vi "state machine plantenna with internal test V2.vi"() -> ()   [LabVIEW 2018]
uses:
  wobbe statemachine.ctl
  Control 1.ctl
  D:/projects/plantenna/stomata programs/plantenna/plantenna/Kinesis_with_LabVIEW_Examples_LV12 - v3/Thorlabs.MotionControl.Controls.dll
  Kinesis_with_LabVIEW_Examples_LV12 - v3/Thorlabs.MotionControl.Controls.dll
  <vilib>/userdefined/High Color/IMAQdx.ctl
  D:/projects/plantenna/stomata programs/plantenna/plantenna/Kinesis_with_LabVIEW_Examples_LV12 - v3/ThorLabs.MotionControl.KCube.DCServoCLI.dll
  Kinesis_with_LabVIEW_Examples_LV12 - v3/ThorLabs.MotionControl.KCube.DCServoCLI.dll
  <vilib>/vision/Image Controls.llb/IMAQ Image.ctl
  <vilib>/Analysis/6fits.llb/Curve Fitting Criteria.ctl
  read settings control.ctl
  write camera.ctl
  <vilib>/Utility/error.llb/DialogType.ctl
  LightStudio 485/labview light studio/chan select.ctl
  <vilib>/vision/driver/IMAQdx.llb/IMAQdx Camera Control Mode.ctl
  <vilib>/Platform/TimedLoop/XDataNode/timing_clust.ctl
  <vilib>/Platform/TimedLoop/XDataNode/nitl_modes.ctl
  <vilib>/Platform/TimedLoop/XDataNode/wakeup.ctl
  <vilib>/DAQmx/write.llb/DAQmx Write (Analog DBL 1Chan 1Samp).vi
  <vilib>/Instr/_visa.llb/VISA Configure Serial Port (Instr).vi
  <vilib>/DAQmx/miscellaneous.llb/DAQmx Fill In Error Info.vi
  <vilib>/Utility/file.llb/Write Delimited Spreadsheet (DBL).vi
  <vilib>/Utility/file.llb/Read Delimited Spreadsheet (string).vi
  <vilib>/platform/TimedLoop/XDataNode/XDataNode.xnode
  <vilib>/vision/driver/NI_Vision_Acquisition_Software.lvlib
  <vilib>/vision/NI_Vision_Development_Module.lvlib
  <vilib>/Analysis/NI_AALPro.lvlib
  <vilib>/Platform/TimedLoop/XDataNode/XDNodeRunTimeDep.lvlib
  <resource>/objmgr/imaqdx.rc
panel:
  out "move error":bool
  out "current state ( setup is idle)":T1=enum."camera settings"
  in  "stopprogram":bool
  in  "User Interface":bool
  in  "control tab":T2(tab)
  in  "blue":bool
  in  "green":bool
  in  "red":bool
  in  "blue":dbl(slide) scale=0.0..100.0
  in  "green":dbl(slide) min=0.0 max=100.0 step=1.0 scale=0.0..100.0
  in  "red":dbl(slide) scale=0.0..100.0
  in  "between meas":bool
  in  "plant light %":dbl(knob) min=0.0 max=100.0 step=0.1 scale=0.0..100.0
  in  "camera settings":bool
  in  "Set ROI":bool
  in  "Microscope light on/off":bool
  in  "StopROI":bool
  in  "use ROI":bool=TRUE
  in  "pics saved":bool
  in  "extra number of steps \nbottom side":dbl=100.0
  in  "extra scan depth \nbottom side(mm)":dbl=0.1
  in  "extra  steps":bool
  in  "extra number of steps \ntop side":dbl=100.0
  in  "extra stepsize (mm)":dbl=0.001
  in  "extra scan depth \ntop side(mm)":dbl=0.1
  out "total scan depth":dbl
  out "total nr of steps":dbl=100.0
  out "step nr":dbl
  out "start":dbl
  out "end":dbl
  in  "set position":dbl
  out "real position":dbl
  in  "number of steps":dbl=100.0
  in  "stepsize (mm)":dbl=0.001 step=0.001
  in  "focus point":dbl step=0.01
  in  "scan depth (mm)":dbl=0.1 min=0.001 step=0.01
  in  "use nonlin steps":bool
  in  "rough extra number \nof steps both sides":dbl=100.0
  in  "rough stepsize (mm)":dbl=0.001
  in  "rough extra scan depth \nboth sides(mm)":dbl=0.1
  in  "max alowed offset":dbl=0.0005
  in  "backlash offset":dbl=0.1
  in  "Test scan\n(no pic. saved)":bool
  in  "Camera settings write":T3={"Pixel format"=1, "exposure time [microsec]"=20.0, "Exposure time setting"=1, "gain [dB]"=0.0, "Auto Gain"=1, "Gamma enable"=FALSE, "gamma "=0.25, "ISP enable "=FALSE, "black level clamping enabled"=FALSE, "black level (%)"=0.0, "binning vertical"=1, "binning hor"=1, "vertical binning mode"=1, "horizontal  binning mode"=1, "width"=8.0, "height "=4.0} {"height" min=0.0 max=2300.0 step=4.0; "width" min=0.0 max=2660.0 step=4.0; "horizontal  binning mode" items=["Additive", "Average"]; "vertical binning mode" items=["Additive", "Average"]; "binning hor" items=["1", "2", "4"]; "binning vertical" items=["1", "2", "4"]; "black level (%)" min=-5.0 max=10.0; "gamma" min=0.25 max=4.0 step=0.1; "Auto Gain" items=["Continuous", "Once", "Off"]; "gain [dB]" min=0.0 max=47.0; "Exposure time setting" items=["Continuous", "Once", "Off"]; "exposure time [microsec]" min=20.0 max=30000000.0; "Pixel format" items=["Mono8", "Mono16", "Mono10Packed", "Mono12Packed", "Mono10p", "Mono12p"]}
  in  "Test Camera settings":bool
  in  "apply settings":bool
  in  "save focus data":bool
  in  "edge detection settings":T4(ring)
  in  "inverse gausian":bool
  in  "Gausian fit method":T5 items=["Least Square", "Least Absolute Residual", "Bisquare"]
  in  "Maximum standard deviation":dbl=0.1
  out "standard deviation 2":dbl
  in  "used for focuspoint":bool=TRUE
  in  "Run with \nexternal \ntiming settings":bool
  out "finished late !\nraise rep time":bool
  in  "start meas now":bool
  out "current time":timestamp format="%<%H:%M:%S>T"
  in  "start fast timer":bool
  in  "start at":timestamp=timestamp(3684335014.687392 s since 1904-01-01) format="%<%H:%M:%S>T"
  out "Last scan time (s)":dbl
  out "rep nr":i32
  out "elapsed time bar  (red idle time)":cluster{dbl, dbl, dbl}(slide)={0.0, 9e-323, 0.0} scale=0.0..60000.0
  out "Elapsed Time (s)":dbl
  in  "nr of repetitions":i32=10 min=1
  in  "repetition time [s]":i64=60 min=1
  in  "load external\n timing settings":bool
  out "plight [%]":i32=1
  out "mlight [%]":i32=1
  in  "serial psi channel":refnum<visa-resource-name>="COM4"
  in  "testrun without psi light":bool
  in  "testrun with pinocam":bool
  in  "Hide test feat.":bool
  in  "testrun without minipam":bool
  in  "testrun without motor":bool
  out "temp rep scan  state array":T1[](array[typedef])
  in  "IR Camera":T6="cam1"
  out "Splitter Position":i32
  in  "motor Serial Number":T7="27600724"
  out "motor prop ref":refnum<k24>
  out "Motor device ref":refnum<k24>
  out "IR camera session ref":T6 caption="Session Out"
  out "filtered image mem loc":T8
  out "Live image mem loc":T8
  out "ROI Mask mem loc":T8
  out "Filename with position":string
  out "filtered image":T8
  out "contrast value array":sgl[](array[numeric])
  out "real position array":dbl[](array[numeric])
  in  "selected path":path
  out "path":path
  out "start time":u32
  out "last scan time (tabs)":u32
  out "rep start time":u32
  in  "first timerscan run ?":bool
  in  "testrun without daq":bool
  in  "plight 100% voltage":dbl=10.0 caption="PLight100%volt" format="%0.2f"
  in  "wait control loop untill init":bool
  out "nrfrep":i32
  out "stop setup loop":bool
  out "rep time":i32
  in  "error in":errorcluster
  out "Initial State":T1=enum."camera settings"
  out "temp scan state array":T1[](array[typedef])
  out "state array":T1[](array[typedef])
  out "cam set read":T9={"Pixel format"=1, "exposure time [microsec]"=20.0, "Exposure time setting"=1, "gain [dB]"=0.0, "Auto Gain"=1, "Gamma enable"=FALSE, "gamma "=0.25, "ISP enable "=FALSE, "black level clamping enabled"=FALSE, "black level (%)"=0.0, "binning vertical"=1, "binning hor"=1, "vertical binning mode"=1, "horizontal  binning mode"=1, "width"=8.0, "height "=4.0, "max width"=8.0, "max height"=8.0, "exposure time vis"=enum."Enabled", "gain vis"=enum."Enabled", "vert binning vis"=[], "hor bin  vis"=[], "gamma vis"=enum."Enabled", "black level vis"=enum."Enabled"} {"max height" min=0.0 max=1330.0; "max width" min=0.0 max=1150.0; "height" min=0.0 max=1330.0; "horizontal  binning mode" items=["Additive", "Average"]; "vertical binning mode" items=["Additive", "Average"]; "binning hor" items=["1", "2", "4"]; "binning vertical" items=["1", "2", "4"]; "black level (%)" min=-5.0 max=10.0; "gamma" min=0.25 max=4.0 step=0.1; "Auto Gain" items=["Continuous", "Once", "Off"]; "gain [dB]" min=0.0 max=47.0; "Exposure time setting" items=["Continuous", "Once", "Off"]; "exposure time [microsec]" min=20.0 max=30000000.0; "Pixel format" items=["Mono8", "Mono16", "Mono10Packed", "Mono12Packed", "Mono10p", "Mono12p"]}
  in  "TIFF Options":T10={"Rows Per Strip"=0, "Photometric"=1, "Compression Type"=0} {"Compression Type" items=["None", "JPEG", "Run Length Encoded", "Zip"]; "Photometric" items=["WhiteIsZero", "BlackIsZero"]}
  out "temp test scan":bool
  out "rep start time 2":timestamp
  in  "io page Visible":bool=TRUE
  out "ROI Descriptor":T11 {"Contours"."Type" items=["No Selection", "Point", "Line", "Rectangle", "Oval", "Polygon", "Freehand Region", "Annulus", "Unused2", "Unused3", "Broken Line", "Freehand Line", "Rotated Rectangle"]}
  in  "encoder counts/rev":i32=34555
  in  "waveform tab":T12(tab)
  out "Waveform Graph":T13(graph)
  out "Live image setup tab":T8(plugin-control)
  in  "initalize motor":refnum<k24>(container)
  out "histogram Mean":sgl format="%#.2f"
  out "histogram Standard Deviation":sgl format="%#.2f"
  out "current time 2":timestamp format="%<%H:%M:%S>T"
  out "timer graph":cluster{cluster{timestamp, dbl}[]}[](graph)
  out "Timer settings array":string[][](array[string])
  out "date from file":string
  out "time from file":string
  out "current date and time":timestamp
  out "next function":string
  out "next function argument":string
  out "focus drift":dbl(graph)
  out "XY Graph":T14(graph)
  out "Gausian fit center":dbl
  out "standard deviation":dbl
  out "max position":dbl
  out "contrast value \n( high is better)":sgl format="%.2f"
  out "Live image camera tab":T8(plugin-control)
  # "nog te doen : microscoop lamp uit tussen de metingen"
  # "PSI light"
  # "settings file: \nYYYY-MM-DD\t    hh:mm:ss    \"command\"    [set]   OR\nDeltaT   hh:mm:ss    \"command\"    [set]\ncommands:\nmlight [on,off, 0-100%] microscope light on/off\nplight     [on,off, 0-100%]  plant light intesity change\nmpam    []  minipam pulse\nredpsiplight[on,off,0-100%] red channel PSI plant light intesity change\ngreenpsiplight[on,off,0-100%] green channel PSI plant light intesity change\nbluepsiplight[on,off,0-100%] blue channel PSI plant light intesity change \nfstack [] do a focus teststack without saving pictures\nrfstack []  do a nonliniar teststack without saving pics\nrstack []  do a single rough non lin stack\nrstack []  do a single stack\nrscan [ number of repetitions   time between meas(sec)] do a single non liniar scan and save the pics \nscan [number of repetitions   time between meas] do a scan and save pics\nexample :\n2020-09-21\t14:08:06\t plight\t80\n2020-09-21\t14:10:00\t mpam\n2020-09-21\t14:10:50  mlight on \n2020-09-21\t14:11:06\t rscan 10  120\n2020-09-21\t14:35:06  fstack\n\nOR\nDeltaT\t 14:08:06\t plight\t80\nDeltaT\t 14:10:00\t mpam\nDeltaT\t\t20:10:50  mlight on \nDeltaT\t 25:11:06\t rscan 10  120\nDeltaT\t\t114:35:06  fstack"
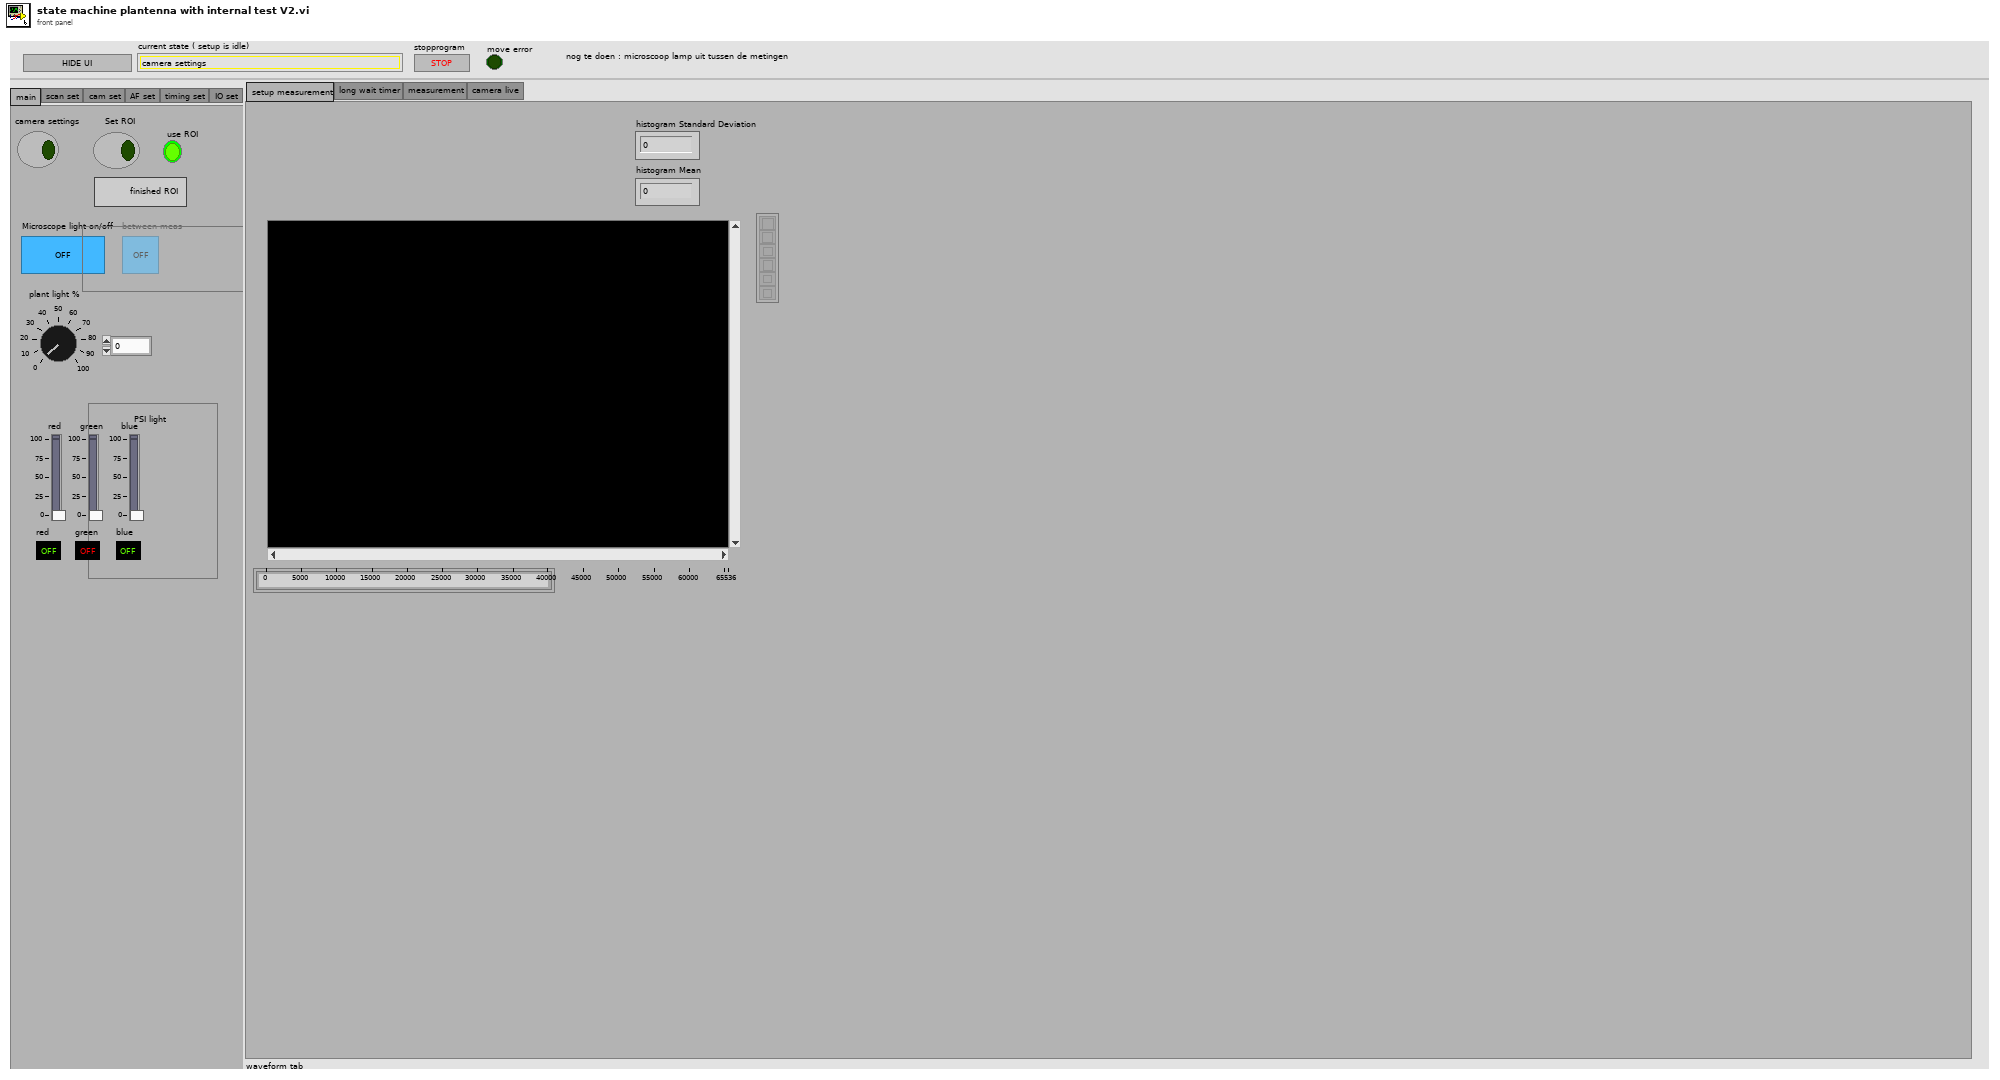
[diagram p1: front panel]
types:
  T1 = typedef "wobbe statemachine.ctl" = enum16{"Initialize", "set up measurement", "camera settings", "set roi", "ad curr date and time to save path", "plight", "mlight", "move to start ", "grab picture without save", "Minipam pulse", "do scan", "do non lin scan", "do test scan", "do non lin test scan", "select save path", "move to position", "grab picture", "focus calculation", "Stop", "timerset", "stop scan timer", "start scan timer", "write scan time", "do multi point scan ", "simple timer", "timerscan", "read temp scan array", "write temp scan state array", "bluepsilight", "greenpsilight", "redpsilight"}
  T2 = enum32{"main", "scan set", "cam set", "AF set", "timing set", "IO set"}
  T3 = typedef "write camera.ctl" = cluster{"Pixel format":u16, "exposure time [microsec]":dbl, "Exposure time setting":u16, "gain [dB]":dbl, "Auto Gain":u16, "Gamma enable":bool, "gamma ":dbl, "ISP enable ":bool, "black level clamping enabled":bool, "black level (%)":dbl, "binning vertical":u16, "binning hor":u16, "vertical binning mode":u16, "horizontal  binning mode":u16, "width":dbl, "height ":dbl}
  T4 = enum16{"Convolution", "Differentiation", "Gradient", "Prewitt", "Roberts", "Sigma", "Sobel"}
  T5 = typedef "NI_AALPro.lvlib/Curve Fitting Criteria.ctl" = u16
  T6 = typedef "IMAQdx.ctl" = refnum<k21>
  T7 = typedef "Control 1.ctl" = string
  T8 = typedef "IMAQ Image.ctl" = refnum<image>
  T9 = typedef "read settings control.ctl" = cluster{"Pixel format":u16, "exposure time [microsec]":dbl, "Exposure time setting":u16, "gain [dB]":dbl, "Auto Gain":u16, "Gamma enable":bool, "gamma ":dbl, "ISP enable ":bool, "black level clamping enabled":bool, "black level (%)":dbl, "binning vertical":u16, "binning hor":u16, "vertical binning mode":u16, "horizontal  binning mode":u16, "width":dbl, "height ":dbl, "max width":dbl, "max height":dbl, "exposure time vis":enum8{"Enabled", "Disabled", "Disabled and Grayed Out"}, "gain vis":enum8{"Enabled", "Disabled", "Disabled and Grayed Out"}, "vert binning vis":i32[], "hor bin  vis":i32[], "gamma vis":enum8{"Enabled", "Disabled", "Disabled and Grayed Out"}, "black level vis":enum8{"Enabled", "Disabled", "Disabled and Grayed Out"}}
  T10 = cluster{"Rows Per Strip":i32, "Photometric":i32, "Compression Type":i32}
  T11 = typedef "ROI Descriptor" = cluster{"Global Rectangle":i32[], "Contours":cluster{"ID":enum32{"External", "Internal"}, "Type":u32, "Coordinates":i32[]}[]}
  T12 = enum32{"setup measurement", "long wait timer", "measurement", "camera live"}
  T13 = cluster{"Starting Value":sgl, "Incremental Value":sgl, "Histogram":u32[]}
  T14 = cluster{"real position array":dbl[], "Best Gaussian Fit":dbl[]}[]
  T15 = enum8{"Enabled", "Disabled", "Disabled and Grayed Out"}
  T16 = typedef "NI_Vision_Acquisition_Software.lvlib/IMAQdx Camera Control Mode.ctl" = enum32{"Controller", "Listener"}
  T17 = typedef "chan select.ctl" = enum16{"red", "green", "blue"}
  T18 = enum32{"Differentiation", "Gradient", "Prewitt", "Roberts", "Sigma", "Sobel"}
  T19 = typedef "XDNodeRunTimeDep.lvlib/timing_clust.ctl" = cluster{"Expected End [f-1]":u64, "Actual End [f-1]":u64, "Finished Late? [f-1]":bool, "Expected End [i-1]":u64, "Actual End [i-1]":u64, "Finished Late? [i-1]":bool, "Expected Start [i]":u64, "Actual Start [i]":u64, "Expected Start [f]":u64, "Actual Start [f]":u64, "Source Name":string, "Structure Name":string, "Period":i64, "Deadline":i64, "Offset":i64, "Start":i64, "Priority":i32, "Timeout":i32, "Mode":T20, "Wakeup Reason":T21, "Error":errorcluster, "Source Type":string, "Secondary Source Type":string, "Global End Time":u64, "Global Start Time":u64, "Frame Duration":u64, "Iteration Duration":u64, "Assigned CPU":i32, "I/O Scan Engine Mode":u32}
  T20 = typedef "XDNodeRunTimeDep.lvlib/nitl_modes.ctl" = enum32{"No Change", "Process missed periods, maintain original phase", "Discard missed periods, maintain original phase", "Process missed periods, ignore original phase", "Discard missed periods, ignore original phase"}
  T21 = typedef "XDNodeRunTimeDep.lvlib/wakeup.ctl" = enum32{"Normal", "Aborted", "Asynchronous wakeup", "Timing source error", "Timed loop error", "Timeout"}
  T22 = enum16{"open", "replace", "create", "open or create", "replace or create", "replace or create with confirmation"}
  T23 = typedef "Image Type" = u32
  T24 = cluster{"last scan time (tabs)":u32, "last scan time (tabs)":u32, u32}
  T25 = typedef "IMAQ Rectangle" = cluster{"Left":i32, "Top":i32, "Right":i32, "Bottom":i32, "Rotation":dbl}
  T26 = cluster{"Global Rectangle":i32[], "Contours":cluster{"Contour Type":u32, "ROI Type":u32, "Points":i32[]}[]}
  T27 = cluster{"real position array":dbl[], "contrast value array":sgl[]}
  T28 = cluster{"real position array":dbl[], "Best Gaussian Fit":dbl[]}
  T29 = cluster{"Timer settings array[0]":string, "Timer settings array[1]":string, "Timer settings array[2]":string, "Timer settings array[3]":string}
  T30 = cluster{"Timer settings array[0]":string, "Timer settings array[1]":string}
  T31 = cluster{"Timer settings array[0]":string, "Timer settings array[1]":string, "Timer settings array[2]":string, "Timer settings array[3]":string, "Timer settings array[4]":string}
  T32 = enum32{"main", "scan set", "camera set", "AF set", "timing set", "IO set"}
  T33 = typedef "DialogType.ctl" = u16
  T34 = enum16{"Always On", "Always Off", "Off While Running"}
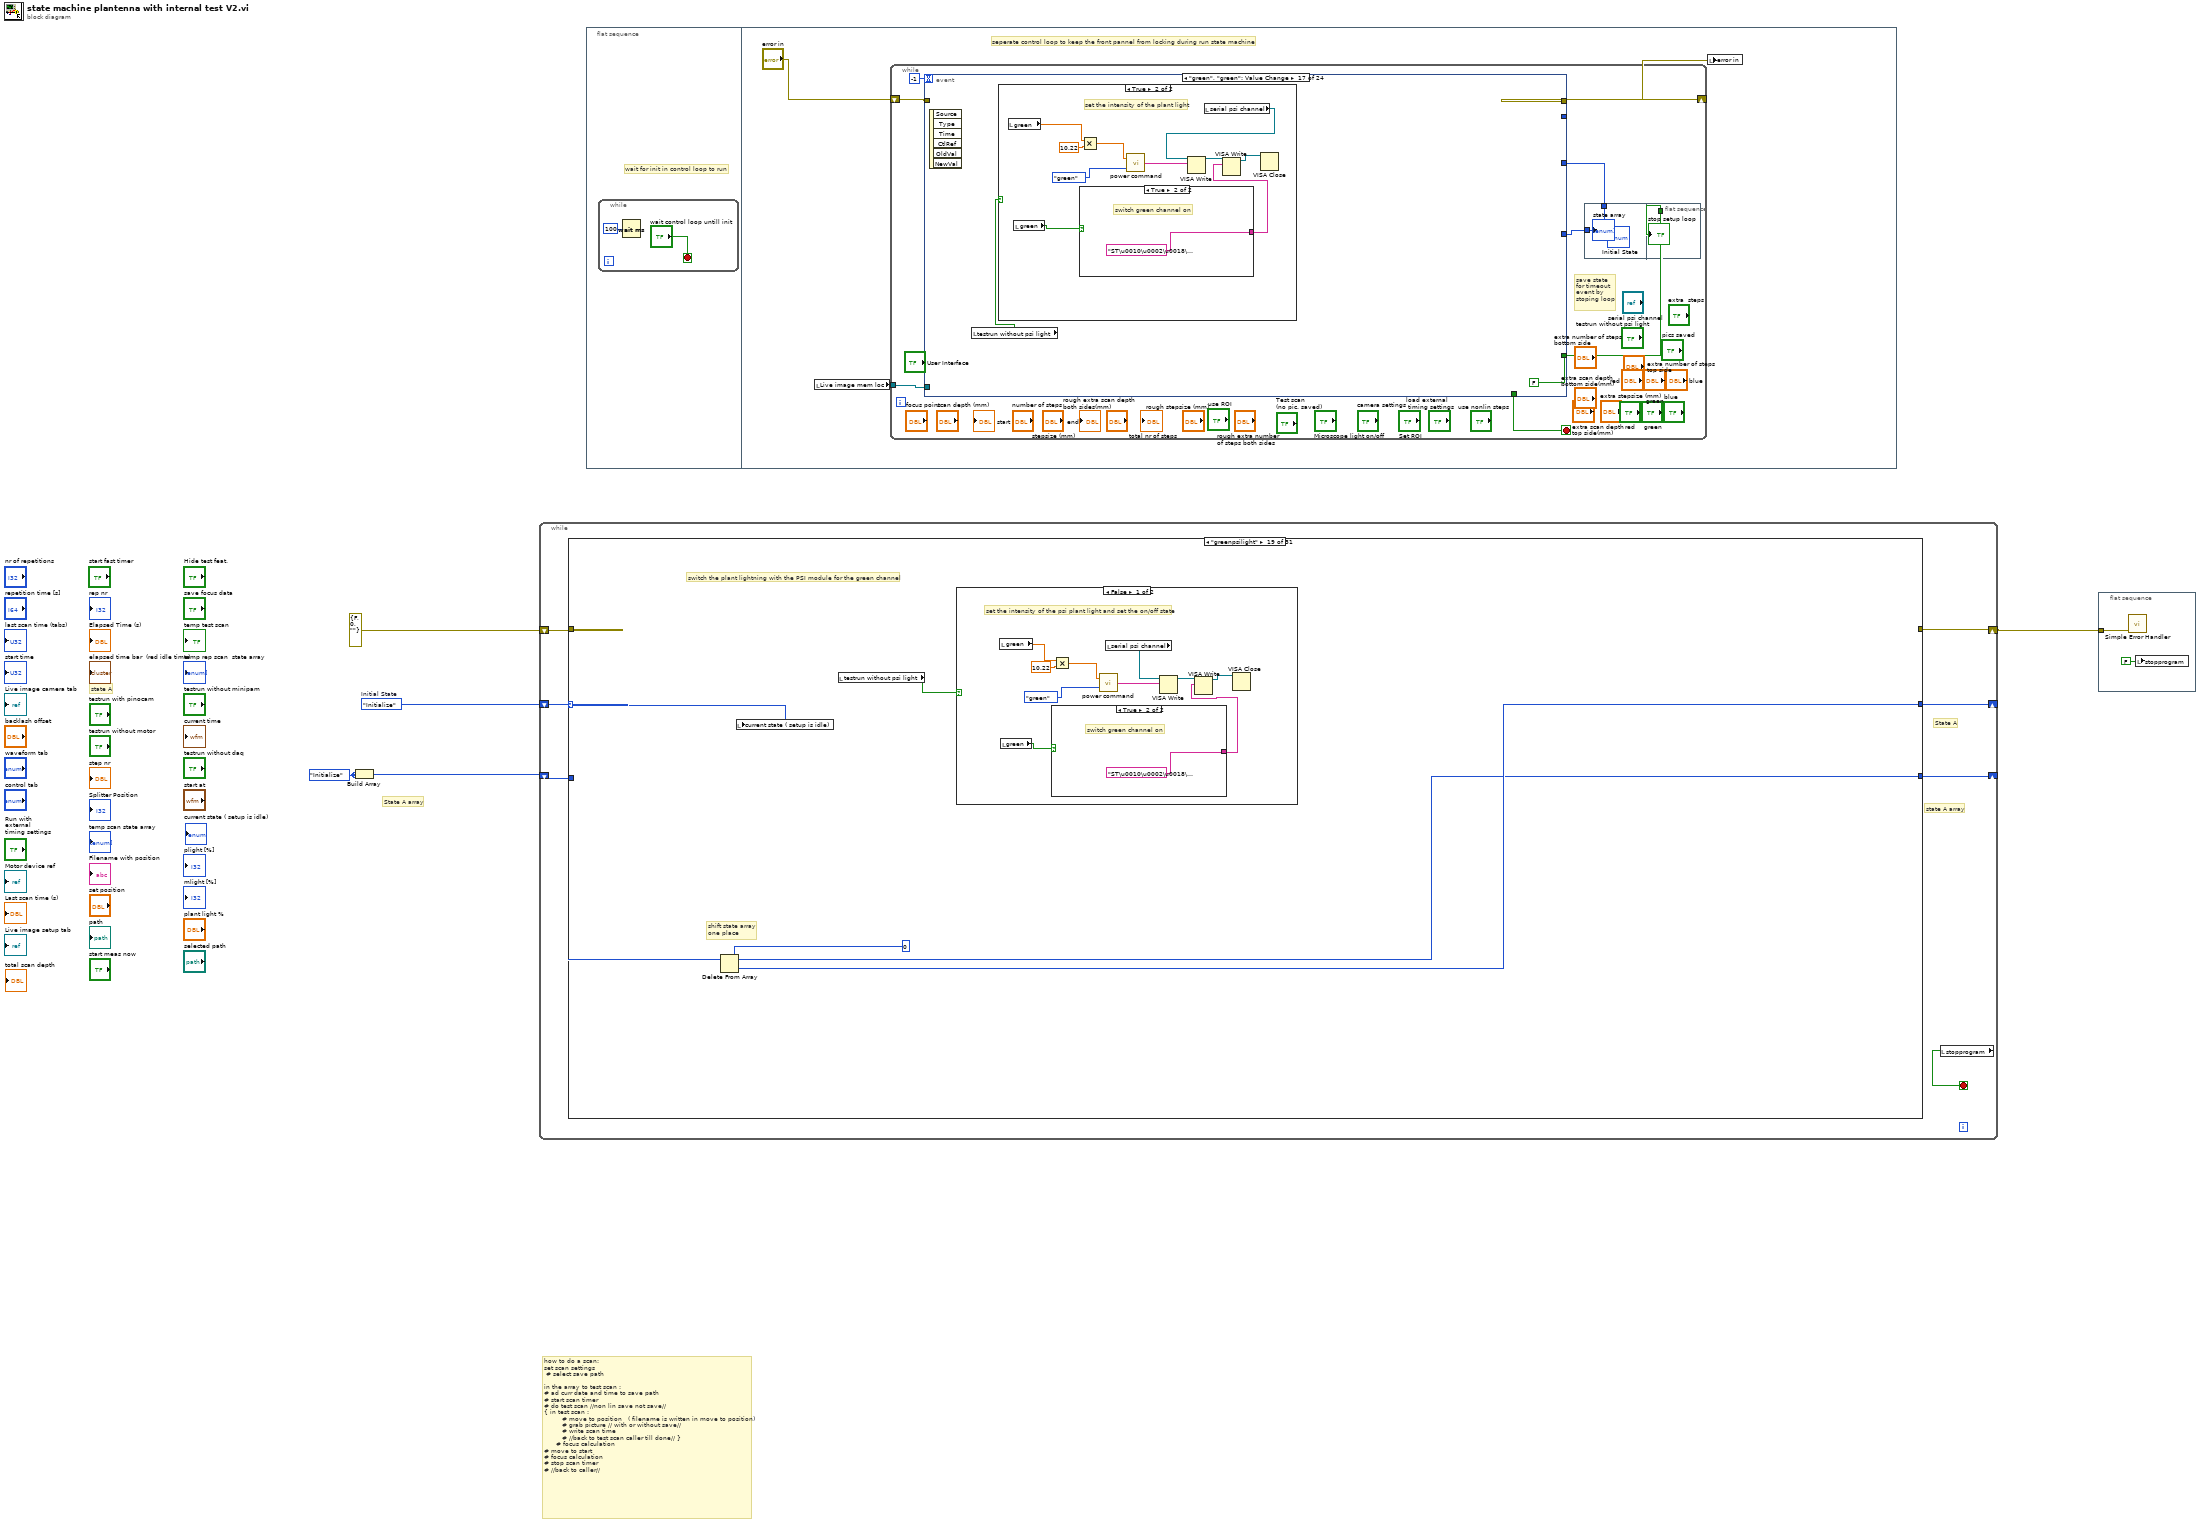
[diagram p0: block diagram]
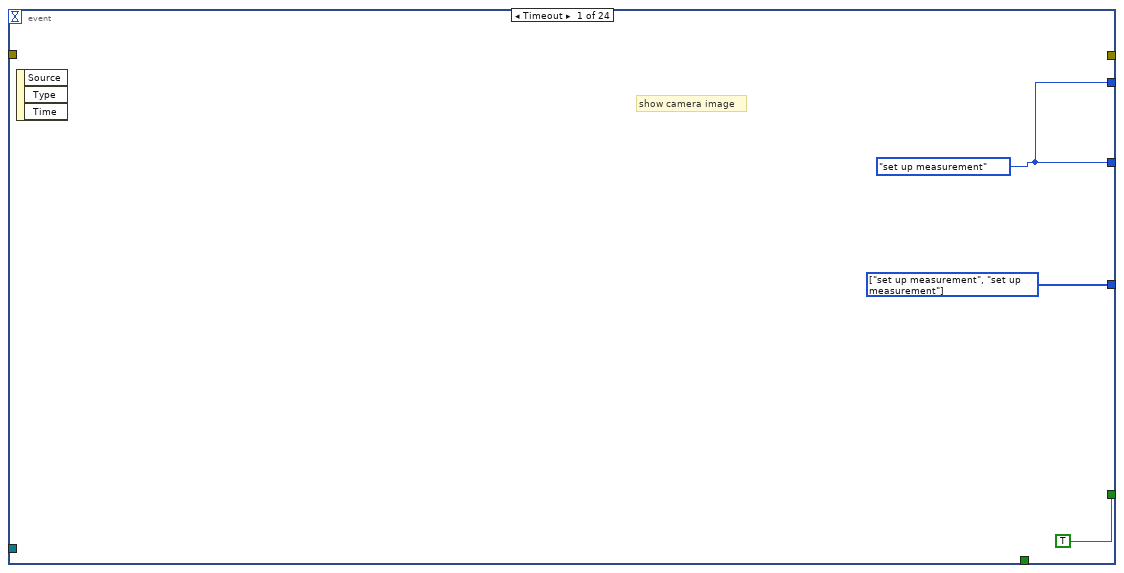
[diagram p2: hidden frame]
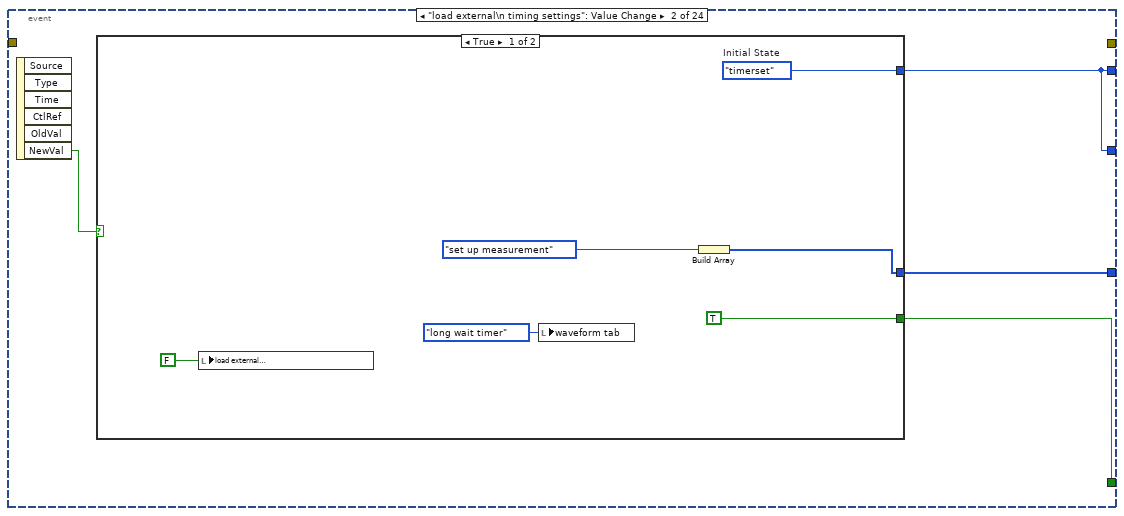
[diagram p3: hidden frame]
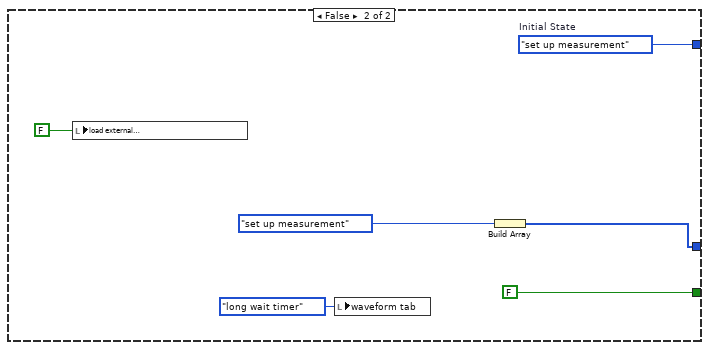
[diagram p4: hidden frame]
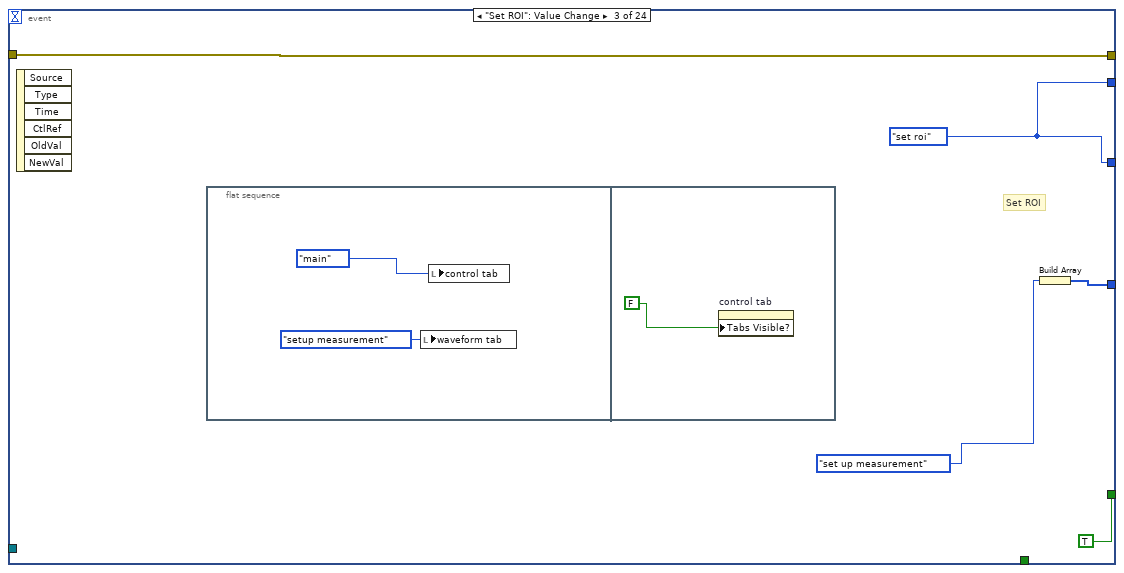
[diagram p5: hidden frame]
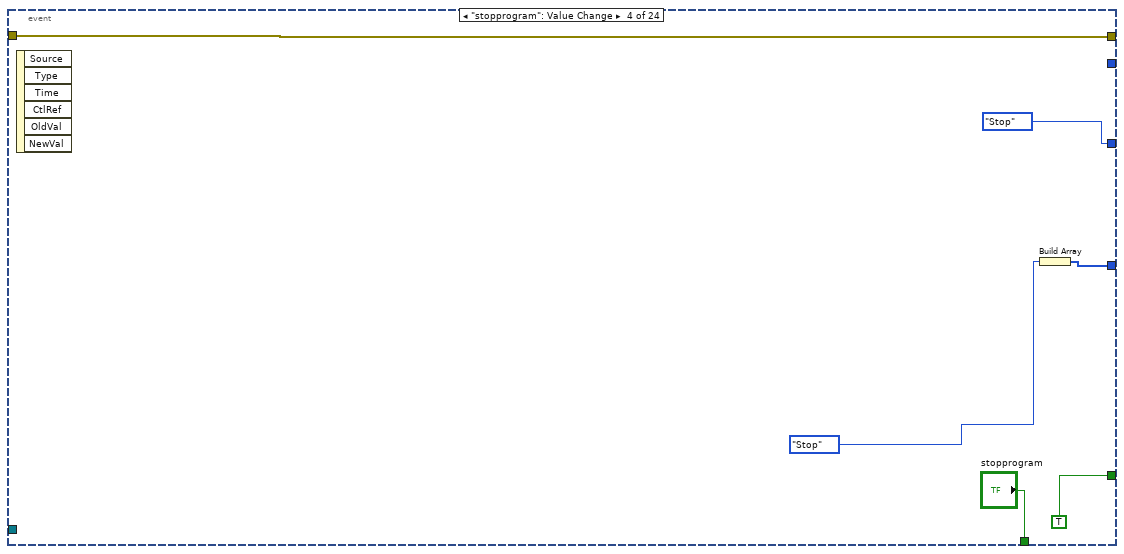
[diagram p6: hidden frame]
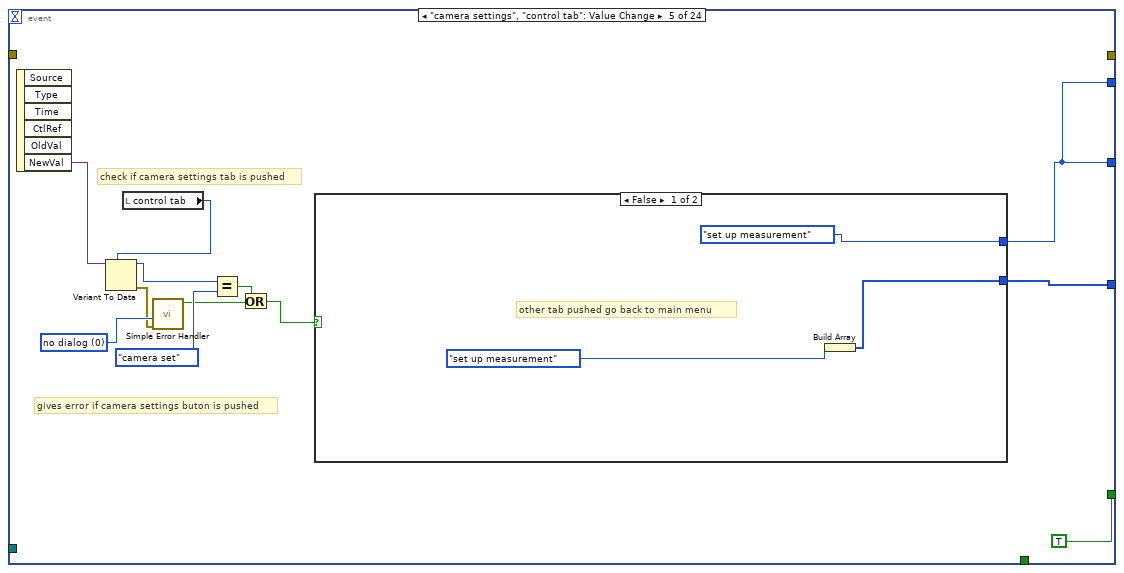
[diagram p7: hidden frame]
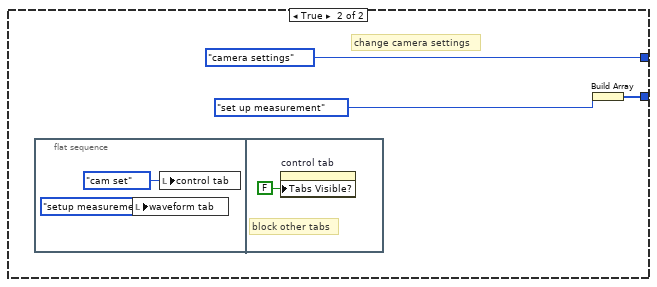
[diagram p8: hidden frame]
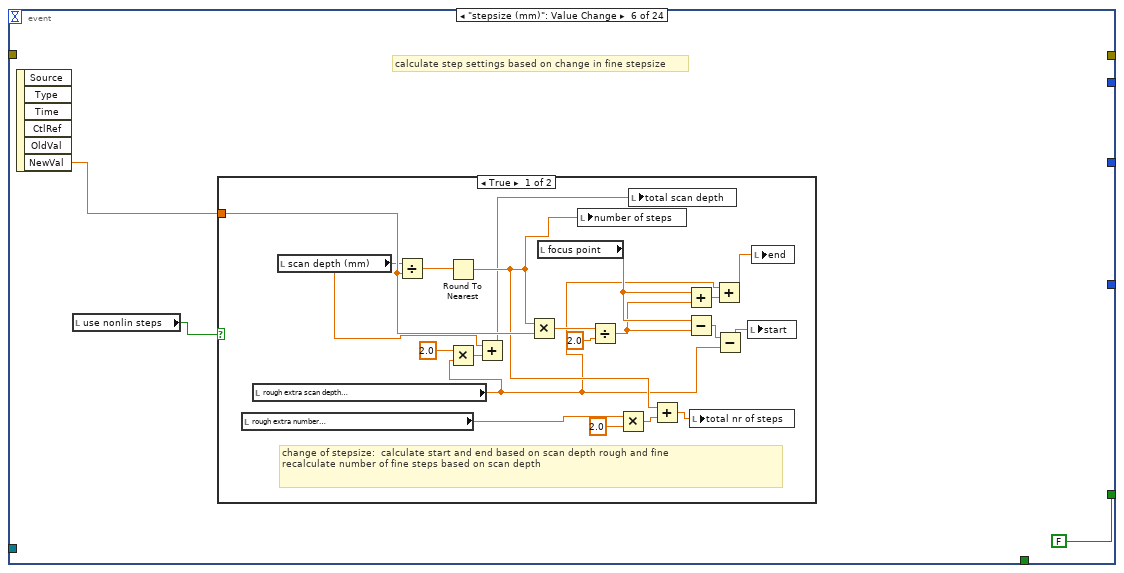
[diagram p9: hidden frame]
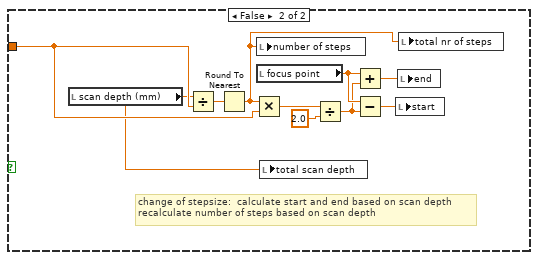
[diagram p10: hidden frame]
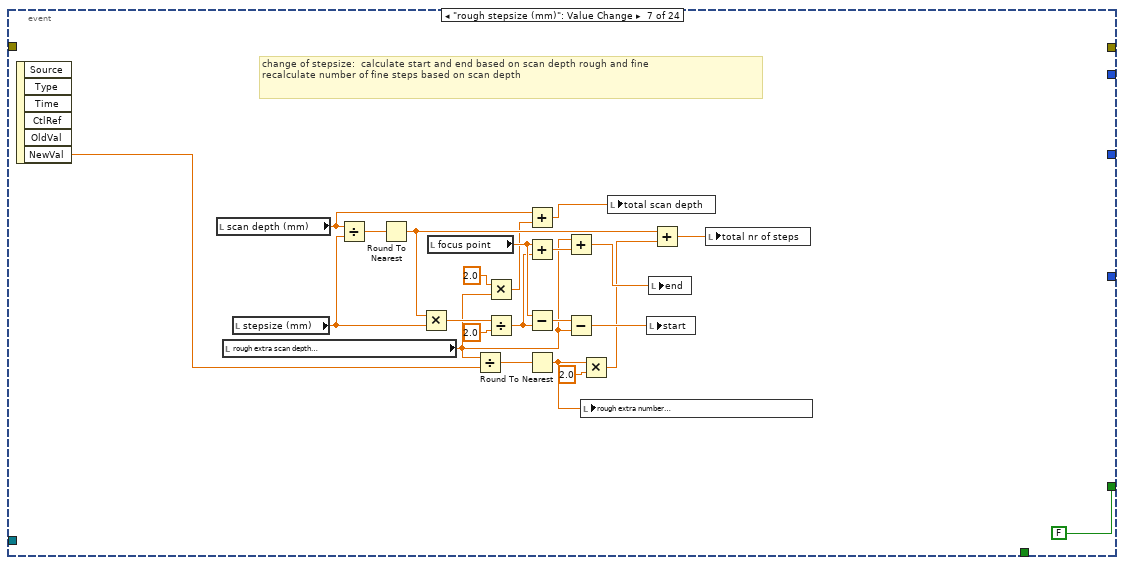
[diagram p11: hidden frame]
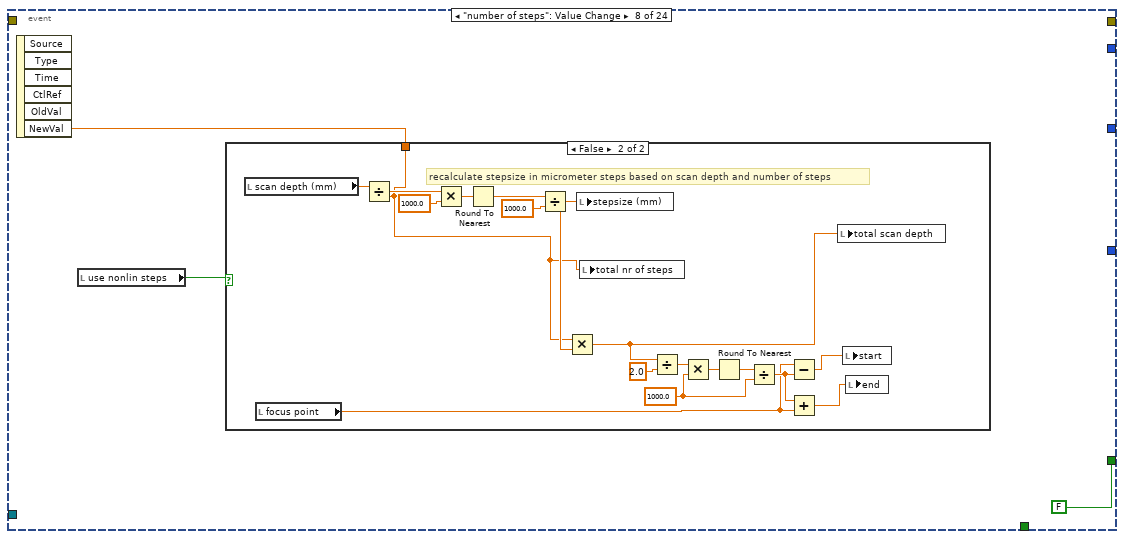
[diagram p12: hidden frame]
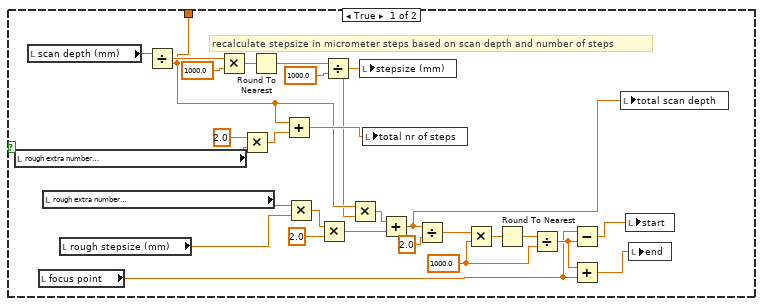
[diagram p13: hidden frame]
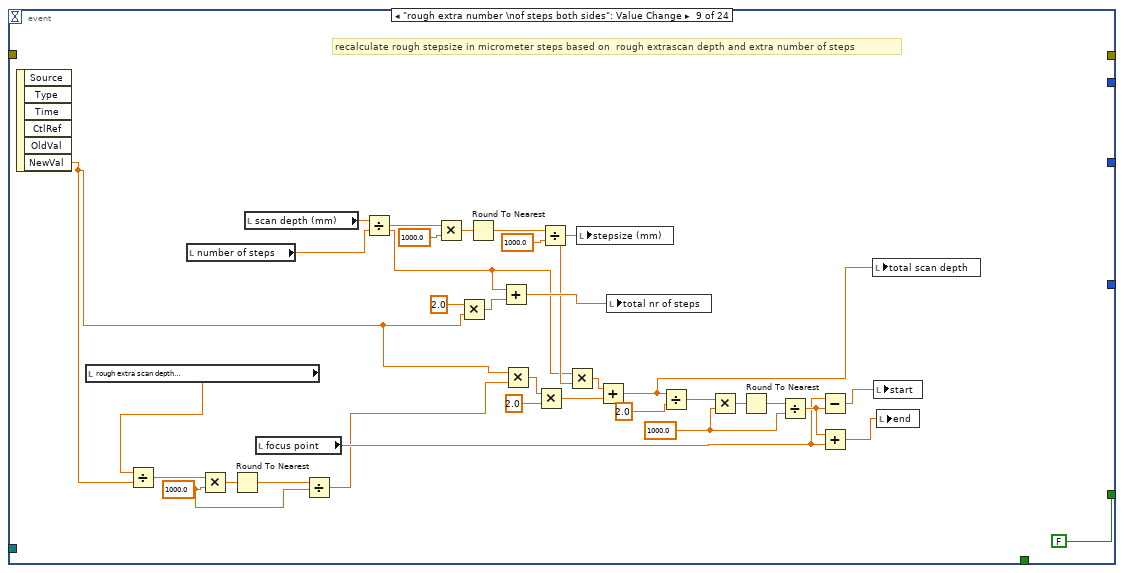
[diagram p14: hidden frame]
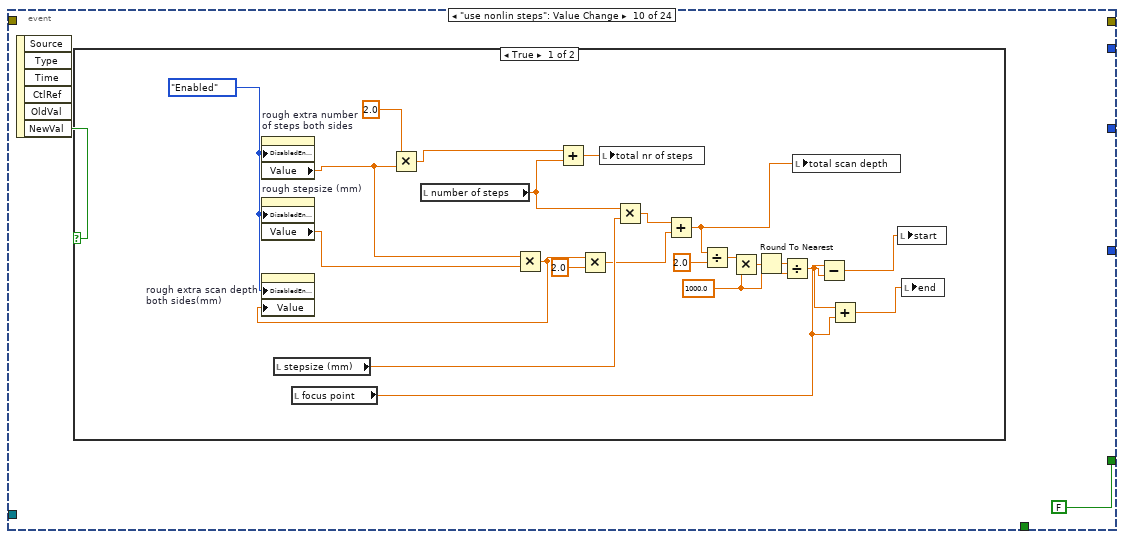
[diagram p15: hidden frame]
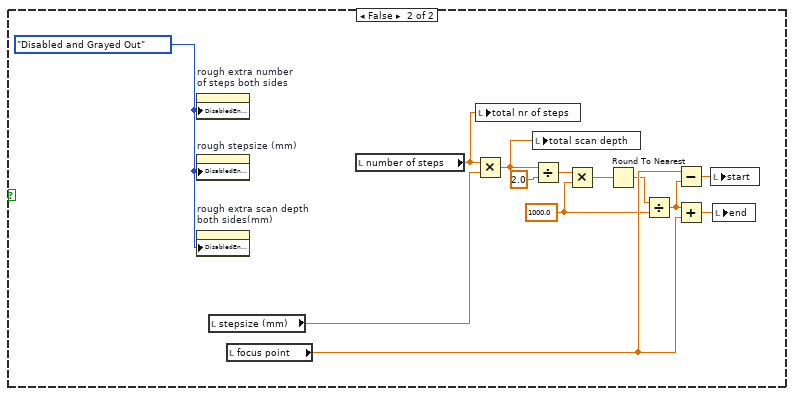
[diagram p16: hidden frame]
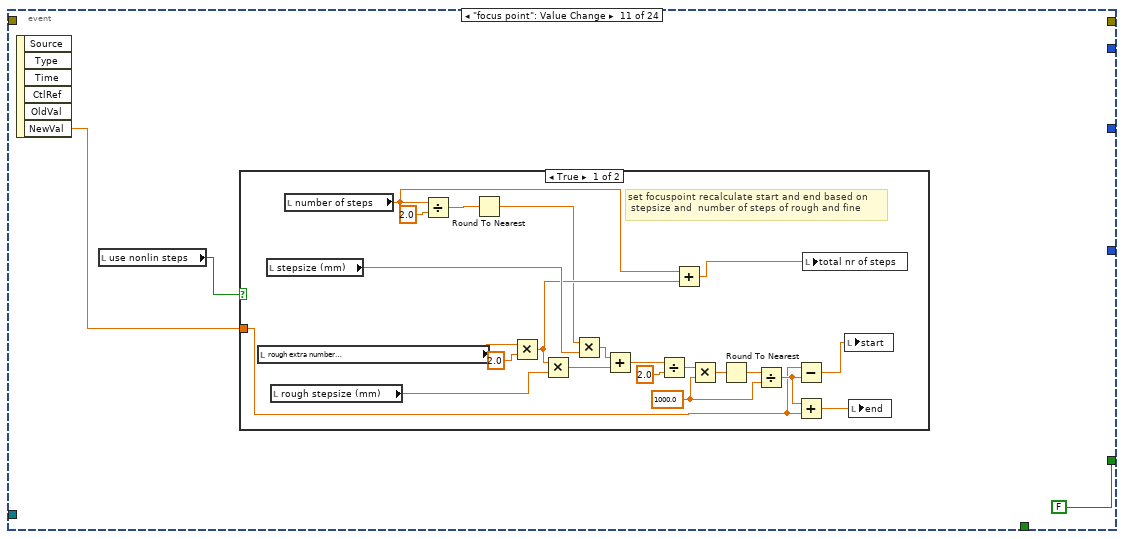
[diagram p17: hidden frame]
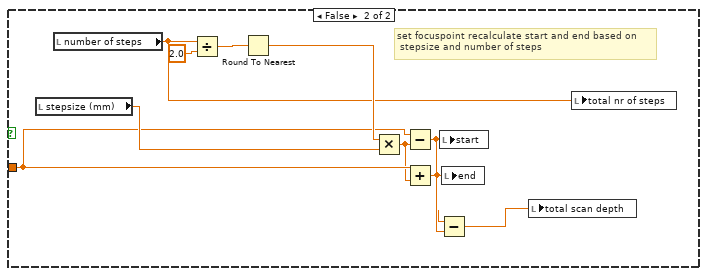
[diagram p18: hidden frame]
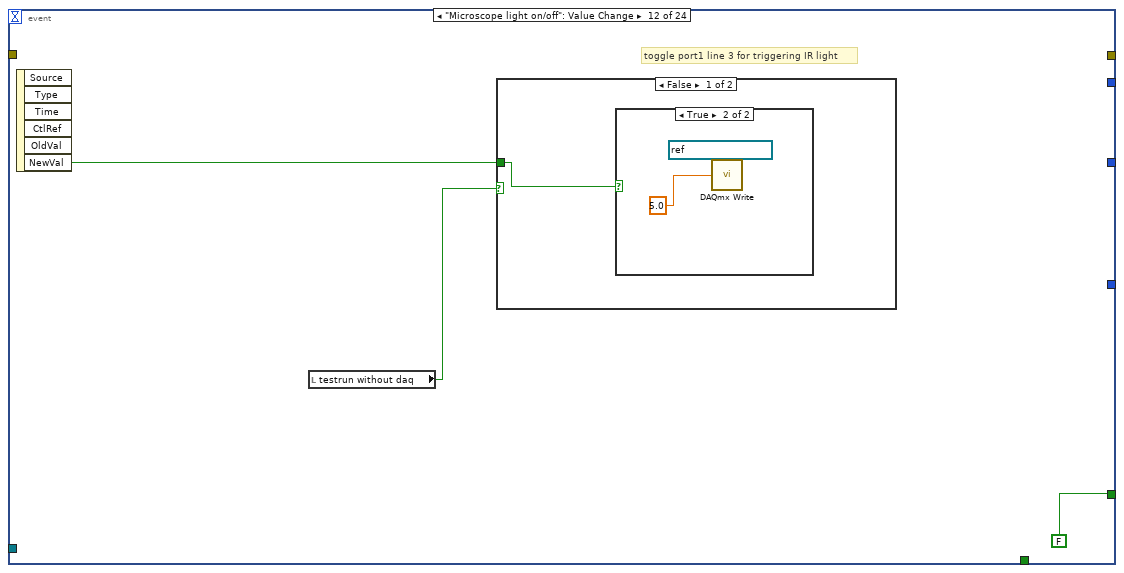
[diagram p19: hidden frame]
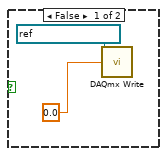
[diagram p20: hidden frame]
diagram:
  w5 = wobbe_statemachine."Initialize" ("Initial State")
  w2 = wobbe_statemachine."Initialize"  # Initial State
  # "how to do a scan:\nset scan settings   \n # select save path\n  \nin the array to test scan : \n# ad curr date and time to save path\n# start scan timer \n# do test scan //non lin save not save//\n{ in test scan :\n         # move to position   ( filename is written in move to position)\n         # grab picture // with or without save//\n         # write scan time\n         # //back to test scan caller till done// }\n      # focus calculation  \n# move to start \n# focus calculation\n# stop scan timer\n# //back to caller//"
  # "State A array"
  # "state A"
  n1 = Build Array(w5, w5) -> (w4:T1[])
  n2 = while {
    shift-right: [w10] -> _
    shift-left: w2 -> [w12]
    shift-right: [w9] -> _
    shift-left: w4 -> [w11]
    shift-right: [w8] -> w1
    shift-left: errorcluster {"status"=FALSE, "code"=0, "source"=""} ("error out") -> [w7]
    stop <- w6 stop-if-true
    # "State A"
    # "state A array"
    n3 = case shown="\"greenpsilight\"" w12 {
      selector: w12 -> [w44 w97 w131 w261 w290 w319 w381 w458 w526 w531 w536 w545 w587 w599 w611 w612 w619 w631 w649 w667 w685 w691 w712 w841 w915 w987 w1059 w1086 w1103 w1118 w1356]
      tunnel: [w42 w100 w143 w257 w286 w316 w378 w455 w523 w528 w534 w541 w584 w596 w608 w614 w621 w633 w651 w669 w687 w693 w706 w838 w912 w972 w1056 w1083 w1105 w1116 wobbe_statemachine."Stop" ("Initial State")] -> w10
      tunnel: w11 -> [w43 _ w146 w256 w285 w315 w377 w454 w524 w529 _ w543 w585 w597 w609 w615 w622 w634 w652 w670 w688 w694 w708 w839 w913 w985 w1057 w1084 w1106 w1115 _]
      tunnel: [w43 w101 w144 w258 w287 w317 w379 w456 w522 w527 w533 w540 w583 w595 w607 w613 w620 w632 w650 w668 w686 w692 w707 w837 w911 w984 w1055 w1082 w1104 w1117 w1353] -> w9
      tunnel: [w19 w98 w130 w253 w282 w312 w374 w453 _ _ _ _ _ _ _ _ _ _ _ _ _ _ w710 w825 w903 w969 _ w1080 _ w1114 _] -> w8
      tunnel: w7 -> [w39 w102 w132 w253 w282 w312 w374 w453 _ _ _ _ _ _ _ _ _ _ _ _ _ _ w711 w833 w907 w980 _ w1081 _ w1114 _]
      frame "Initialize", Default {
        w36 = T23 7 items=["Grayscale (U8)", "Grayscale (I16)", "Grayscale (SGL)", "Complex (CSG)", "RGB (U32)", "HSL (U32)", "RGB (U64)", "Grayscale (U16)"] ("Image Type")
        w42 = wobbe_statemachine."set up measurement"  # Initial State
        n4 = local write "current state ( setup is idle)"(w44) -> ()
        n5 = local read "testrun without psi light"() -> (w13:bool)
        n6 = case shown="False" w13 {
          frame False {
            w51 = u16 0 items=["None", "XON/XOFF", "RTS/CTS", "XON/XOFF & RTS/CTS", "DTR/DSR", "XON/XOFF & DTR/DSR"] ("flow control (0:none)")
            w52 = u16 10 items=["1.0"=10, "1.5"=15, "2.0"=20] ("stop bits (10: 1 bit)")
            n7 = local read "serial psi channel"() -> (w47:refnum<visa-resource-name>)
            n8 = call-poly "VISA Configure Serial Port"("VISA resource name"=w47, "timeout (10sec)"=u32 10000, "termination char\n(0xA = '\\n' = LF)"=u8 10 ("termination char\n(0xA = '\\n' = LF)"), "Enable Termination\nChar (T)"=FALSE ("Enable Termination\nChar (T)"), "baud rate (9600)"=u32 28800, "data bits (8)"=u16 8, "parity (0:none)"=enum16{"None", "Odd", "Even", "Mark", "Space"}."None", "stop bits (10: 1 bit)"=w52, "flow control (0:none)"=w51) -> ("VISA resource name out"=w46:refnum<visa-resource-name>)  [unwired: 5 in, 1 out]
            n9 = local write "serial psi channel"(w46) -> ()
          }
          frame True {
          }
        }
        n10 = local write "rep nr"(0 ("rep nr")) -> ()
        n11 = local write "stop setup loop"(FALSE ("stop setup loop")) -> ()
        n12 = local write "temp test scan"(FALSE ("temp test scan")) -> ()
        n13 = local write "stopprogram"(FALSE ("stop")) -> ()
        n14 = local write "first timerscan run ?"(TRUE ("first timerscan run ?")) -> ()
        n15 = local read "testrun without motor"() -> (w26:bool)
        n16 = local write "Timer settings array"(string[][] [] ("Timer settings array")) -> ()
        n17 = case shown="False" w26 {
          tunnel: [w88 w95] -> w41
          tunnel: w39 -> [w87 w95]
          frame False {
            # "init stage control"
            n18 = property class="KCubeDCServoControl"(reference="initalize motor", error in=w87, "SerialNumber"="motor Serial Number") -> (reference out=w94:refnum<k24>, error out=w91:errorcluster)
            n19 = invoke class="KCubeDCServoControl" method="CreateDevice"(reference=w94, error in=w91) -> (reference out=w93:refnum<k24>, error out=w90:errorcluster)  [unwired: 1 in, 1 out]
            n20 = property class="KCubeDCServoControl"(reference=w93, error in=w90) -> (reference out=→"motor prop ref":refnum<k24>, error out=w88:errorcluster, "Device"=w85:refnum<k24>)
            n21 = local write "Motor device ref"(w85) -> ()
          }
          frame True {
          }
        }
        n22 = local write "step nr"(0.0 ("step nr")) -> ()
        n23 = property on="Splitter 2" class="Splitter"() -> ("Position"=w45:i32)  [unwired: 2 in, 2 out]
        n24 = local write "control tab"(T2."main" ("control tab")) -> ()
        n25 = local write "Splitter Position"(w45) -> ()
        n26 = call "IMAQ Create"("Image Name"="live image", "Image Type"=w36) -> ("New Image"=→"Live image mem loc":T8)  [unwired: 3 in, 1 out]
        n27 = call "IMAQ Create"("Image Name"="filtered image", "Image Type"=w36) -> ("New Image"=→"filtered image mem loc":T8)  [unwired: 3 in, 1 out]
        n28 = call "IMAQ Create"("Image Name"=" Mask") -> ("New Image"=→"ROI Mask mem loc":T8)  [unwired: 4 in, 1 out]
        n29 = property on="focus drift" class="WFChart (strict)"("History Data"=dbl[] []) -> ()  [unwired: 2 in, 2 out]
        n30 = property on="control tab" class="TabCtl (strict)"() -> ("Pages"=w17:refnum<vi>[])  [unwired: 2 in, 2 out]
        n31 = Index Array(array=w17, index=5) -> (element=w14:refnum<vi>)
        n32 = local read "testrun with pinocam"() -> (w23:bool)
        n33 = property class="Page"(reference=w14, "PageVis"="io page Visible") -> ()  [unwired: 1 in, 2 out]
        n34 = case shown="True" w23 {
          tunnel: w41 -> [w71 w83]
          tunnel: "IR Camera" -> [w70 w82]
          tunnel: [w69 w79] -> w25
          tunnel: [w68 w78] -> w20
          frame True {
            # "init camera"
            n35 = property on="control tab" class="TabCtl (strict)"() -> ("Pages"=w61:refnum<vi>[])  [unwired: 2 in, 2 out]
            n36 = call <vilib>:"IMAQdx Open Camera.vi"("Camera Control Mode"=IMAQdx_Camera_Control_Mode."Controller", "error in"=w71, "Session In"=w70) -> ("error out"=w64:errorcluster, "Session Out"=w66:T6)  [unwired: 7 in]
            n37 = Index Array(array=w61, index=2) -> (element=w62:refnum<vi>)
            n38 = property class="IMAQdx"(reference=w66, error in=w64, "VideoMode"=u32 25) -> (reference out=w65:T6, error out=w63:errorcluster)
            n39 = property class="Page"(reference=w62, "PageVis"=FALSE ("Page Visible")) -> ()  [unwired: 1 in, 2 out]
            n40 = property on="camera settings" class="Bool"("DisabledEnum"=T15."Disabled and Grayed Out" ("Disabled")) -> ()  [unwired: 2 in, 2 out]
            n41 = call <vilib>:"IMAQdx Configure Grab.vi"("error in"=w63, "Session In"=w65) -> ("error out"=w68:errorcluster, "Session Out"=w69:T6)  [unwired: 8 in]
          }
          frame False {
            # "init camera"
            n42 = property on="control tab" class="TabCtl (strict)"() -> ("Pages"=w76:refnum<vi>[])  [unwired: 2 in, 2 out]
            n43 = call <vilib>:"IMAQdx Open Camera.vi"("Camera Control Mode"=IMAQdx_Camera_Control_Mode."Controller", "error in"=w83, "Session In"=w82) -> ("error out"=w80:errorcluster, "Session Out"=w81:T6)  [unwired: 7 in]
            n44 = Index Array(array=w76, index=2) -> (element=w77:refnum<vi>)
            n45 = property class="Page"(reference=w77, "PageVis"=TRUE ("Page Visible")) -> ()  [unwired: 1 in, 2 out]
            n46 = property on="camera settings" class="Bool"("DisabledEnum"=T15."Enabled" ("Disabled")) -> ()  [unwired: 2 in, 2 out]
            n47 = call <vilib>:"IMAQdx Configure Grab.vi"("error in"=w80, "Session In"=w81) -> ("error out"=w78:errorcluster, "Session Out"=w79:T6)  [unwired: 8 in]
          }
        }
        "IR camera session ref" <- w25
        n48 = flat-sequence {
          tunnel: w20 -> [w57]
          tunnel: [w57] -> w19
          frame #0 {
            n49 = local write "wait control loop untill init"(TRUE ("start")) -> ()
          }
        }
      }
      frame "set up measurement" {
        n50 = flat-sequence {
          tunnel: w97 -> [w104]
          tunnel: [w104] -> w96
          frame #0 {
            n51 = property on="current state ( setup is idle)" class="Enum (strict)"("RingText.BGColor"=u32 14869218 ("Pane Color")) -> ()  [unwired: 2 in, 2 out]
          }
        }
        n52 = local write "error in"(w102) -> ()
        n53 = local write "current state ( setup is idle)"(w96) -> ()
        n54 = while {
          tunnel: [w123] -> w101
          tunnel: [w122] -> w99
          tunnel: [w121] -> w100
          stop <- w120 stop-if-true
          # "show picture during setup of the measurement"
          # "make testmode webcam pic grayscale"
          n55 = local read "Live image mem loc"() -> (w109:T8)
          n56 = local read "IR camera session ref"() -> (w111:T6)
          n57 = local read "use ROI"() -> (w115:bool)
          n58 = local read "testrun with pinocam"() -> (w119:bool)
          n59 = Wait (ms)(milliseconds to wait=u32 100) -> ()  [unwired: 1 out]
          n60 = case shown="False" w115 {
            tunnel: [_ w128] -> w116
            frame False {
            }
            frame True {
              n61 = local read "ROI Mask mem loc"() -> (w128:T8)
            }
          }
          n62 = call <vilib>:"IMAQdx Grab2.vi"("Image In"=w109, "Session In"=w111) -> ("Image Out"=w117:T8)  [unwired: 6 in, 3 out]
          n63 = case shown="True" w119 {
            tunnel: w117 -> [w124 w126]
            tunnel: [w124 w125] -> w118
            frame False {
            }
            frame True {
              w127 = T23 7 items=["Grayscale (U8)", "Grayscale (I16)", "Grayscale (SGL)", "Complex (CSG)", "RGB (U32)", "HSL (U32)", "RGB (U64)", "Grayscale (U16)"] ("Image Type")
              n64 = call "IMAQ Cast Image"("Image Type"=w127, "Image Src"=w126) -> ("Image Dst Out"=w125:T8)  [unwired: 8 in, 1 out]
            }
          }
          n65 = call "IMAQ Histograph"("Image Mask"=w116, "Image"=w118) -> ("Standard  Deviation"=w113:sgl, "Mean Value"=w114:sgl, "Histogram Graph"=w112:T13)  [unwired: 6 in, 1 out]
          n66 = local write "Live image setup tab"(w117) -> ()
          n67 = local write "Live image camera tab"(w117) -> ()
          n68 = local write "Waveform Graph"(w112) -> ()
          n69 = local write "histogram Standard Deviation"(w113) -> ()
          n70 = local write "histogram Mean"(w114) -> ()
          n71 = local read "stop setup loop"() -> (w120:bool)
          n72 = local read "state array"() -> (w123:T1[])
          n73 = local read "error in"() -> (w122:errorcluster)
          n74 = local read "Initial State"() -> (w121:T1)
        }
        n75 = flat-sequence {
          tunnel: w99 -> [w108]
          tunnel: [w108] -> w98
          frame #0 {
            n76 = property on="current state ( setup is idle)" class="Enum (strict)"("RingText.BGColor"=u32 16774656 ("Ring Text.Colors:BG Color")) -> ()  [unwired: 2 in, 2 out]
            n77 = local write "stop setup loop"(FALSE ("stop setup loop")) -> ()
            n78 = property on="control tab" class="TabCtl (strict)"("Blinking"=FALSE) -> ()  [unwired: 2 in, 2 out]
          }
        }
      }
      frame "camera settings" {
        # "shift state array \none place"
        n79 = flat-sequence {
          tunnel: [w150] -> w142
          tunnel: [w149] -> w141
          tunnel: [w148] -> w140
          tunnel: w132 -> [w148]
          tunnel: w131 -> [w147]
          tunnel: w142 -> [w179]
          tunnel: w141 -> [w180]
          tunnel: w140 -> [w160]
          tunnel: [w180] -> w139
          tunnel: [w161] -> w138
          tunnel: [w159] -> w137
          tunnel: [w158] -> w136
          tunnel: w139 -> [w185]
          tunnel: [w183] -> w135
          tunnel: [w184] -> w134
          tunnel: [w182] -> w133
          tunnel: w138 -> [w187]
          tunnel: w137 -> [w186]
          tunnel: w136 -> [w181]
          tunnel: [w251] -> w130
          tunnel: [w252] -> _
          tunnel: w135 -> [w249]
          tunnel: w134 -> [w252]
          tunnel: w133 -> [w251]
          tunnel: [w249] -> w129
          frame #0 {
            # "open camera\nand init picture"
            n80 = local read "Live image mem loc"() -> (w149:T8)
            n81 = local read "IR camera session ref"() -> (w150:T6)
            n82 = local write "current state ( setup is idle)"(w147) -> ()
          }
          frame #1 {
            # "Read actual camera settings"
            n83 = call "read camera settingssub.vi"("camera session  in"=w179, "error in"=w160) -> ("camera session out"=w161:T6, "error out"=w159:errorcluster, "Camera settings"=w178:T9)
            "cam set read" <- w178
            n84 = Unbundle By Name(w178) -> ("Pixel format"=w158:u16, "exposure time [microsec]"=w177:dbl, "Exposure time setting"=w176:u16, "gain [dB]"=w175:dbl, "Auto Gain"=w174:u16, "Gamma enable"=w173:bool, "gamma"=w172:dbl, "ISP enable"=w171:bool, "black level clamping enabled"=w170:bool, "black level (%)"=w169:dbl, "binning vertical"=w168:u16, "binning hor"=w167:u16, "vertical binning mode"=w166:u16, "horizontal  binning mode"=w165:u16, "width"=w164:dbl, "height"=w163:dbl, "max width"=w156:dbl, "max height"=w155:dbl, "exposure time vis"=w154:T15, "gain vis"=w153:T15, "gamma vis"=w152:T15, "black level vis"=w151:T15)
            n85 = Bundle By Name(cluster="Camera settings write", "Pixel format"=w158, "exposure time [microsec]"=w177, "Exposure time setting"=w176, "gain [dB]"=w175, "Auto Gain"=w174, "Gamma enable"=w173, "gamma"=w172, "ISP enable"=w171, "black level clamping enabled"=w170, "black level (%)"=w169, "binning vertical"=w168, "binning hor"=w167, "vertical binning mode"=w166, "horizontal  binning mode"=w165, "width"=w164, "height"=w163) -> (w162:T3)
            n86 = property on="width" class="DigNum (strict)"("Maximum"=w156) -> ()  [unwired: 2 in, 2 out]
            n87 = property on="gain [dB]" class="DigNum (strict)"("DisabledEnum"=w153) -> ()  [unwired: 2 in, 2 out]
            n88 = property on="height" class="DigNum (strict)"("Maximum"=w155) -> ()  [unwired: 2 in, 2 out]
            n89 = property on="exposure time [microsec]" class="DigNum (strict)"("DisabledEnum"=w154) -> ()  [unwired: 2 in, 2 out]
            n90 = property on="gamma" class="DigNum (strict)"("DisabledEnum"=w152) -> ()  [unwired: 2 in, 2 out]
            n91 = property on="black level (%)" class="DigNum (strict)"("DisabledEnum"=w151) -> ()  [unwired: 2 in, 2 out]
            n92 = local write "Camera settings write"(w162) -> ()
          }
          frame #2 {
            n93 = while {
              shift-right: [w195] -> w183
              shift-left: w187 -> [w198]
              shift-right: [w196] -> w182
              shift-left: w186 -> [w197]
              shift-right: [w193] -> w184
              shift-left: w185 -> [w194]
              shift-right: [w191] -> _
              shift-left: w181 -> [w190]
              stop <- "apply settings" stop-if-true
              # "change histogram x scale"
              # "change camera settings"
              n94 = case shown="True" "Test Camera settings" {
                tunnel: w198 -> [w214 w247]
                tunnel: w197 -> [w213 w246]
                tunnel: [w210 w224] -> w195
                tunnel: [w209 w223] -> w196
                tunnel: w194 -> [w208 w222]
                tunnel: [w207 w222] -> w193
                tunnel: [w206 w221] -> w191
                tunnel: w190 -> [w206 _]
                frame False {
                  n95 = call <vilib>:"IMAQdx Configure Grab.vi"("error in"=w213, "Session In"=w214) -> ("error out"=w211:errorcluster, "Session Out"=w212:T6)  [unwired: 8 in]
                  n96 = call <vilib>:"IMAQdx Grab2.vi"("error in"=w211, "Image In"=w208, "Session In"=w212) -> ("error out"=w209:errorcluster, "Image Out"=w207:T8, "Session Out"=w210:T6)  [unwired: 5 in, 1 out]
                }
                frame True {
                  n97 = local read "Camera settings write"() -> (w226:T3)
                  n98 = local write "Test Camera settings"(FALSE ("Test Camera settings")) -> ()
                  n99 = call "write camera settings.vi"("Camera settings"=w226, "error in"=w246, "camera session  in"=w247) -> ("error out"=w243:errorcluster, "camera session out"=w244:T6)  [unwired: 1 in]
                  n100 = call "read camera settingssub.vi"("camera session  in"=w244, "error in"=w243) -> ("camera session out"=w224:T6, "error out"=w223:errorcluster, "Camera settings"=w227:T9)
                  n101 = Unbundle By Name(w227) -> ("Pixel format"=w221:u16, "exposure time [microsec]"=w242:dbl, "Exposure time setting"=w241:u16, "gain [dB]"=w240:dbl, "Auto Gain"=w239:u16, "Gamma enable"=w238:bool, "gamma"=w237:dbl, "ISP enable"=w236:bool, "black level clamping enabled"=w235:bool, "black level (%)"=w234:dbl, "binning vertical"=w233:u16, "binning hor"=w232:u16, "vertical binning mode"=w231:u16, "horizontal  binning mode"=w230:u16, "width"=w229:dbl, "height"=w228:dbl, "max width"=w220:dbl, "max height"=w219:dbl, "exposure time vis"=w218:T15, "gain vis"=w217:T15, "gamma vis"=w216:T15, "black level vis"=w215:T15)
                  n102 = Bundle By Name(cluster=w226, "Pixel format"=w221, "exposure time [microsec]"=w242, "Exposure time setting"=w241, "gain [dB]"=w240, "Auto Gain"=w239, "Gamma enable"=w238, "gamma"=w237, "ISP enable"=w236, "black level clamping enabled"=w235, "black level (%)"=w234, "binning vertical"=w233, "binning hor"=w232, "vertical binning mode"=w231, "horizontal  binning mode"=w230, "width"=w229, "height"=w228) -> (w225:T3)
                  n103 = local write "Camera settings write"(w225) -> ()
                  n104 = property on="width" class="DigNum (strict)"("Maximum"=w220) -> ()  [unwired: 2 in, 2 out]
                  n105 = property on="gain [dB]" class="DigNum (strict)"("DisabledEnum"=w217) -> ()  [unwired: 2 in, 2 out]
                  n106 = property on="height" class="DigNum (strict)"("Maximum"=w219) -> ()  [unwired: 2 in, 2 out]
                  n107 = property on="exposure time [microsec]" class="DigNum (strict)"("DisabledEnum"=w218) -> ()  [unwired: 2 in, 2 out]
                  n108 = property on="gamma" class="DigNum (strict)"("DisabledEnum"=w216) -> ()  [unwired: 2 in, 2 out]
                  n109 = property on="black level (%)" class="DigNum (strict)"("DisabledEnum"=w215) -> ()  [unwired: 2 in, 2 out]
                }
              }
              n110 = case shown="2, 4" w191 {
                tunnel: [65536 ("Number of Classes") 4096 ("Number of Classes") 256 ("Number of Classes") 1024 ("Number of Classes")] -> w192
                frame 1, Default {
                }
                frame 3, 5 {
                }
                frame 0 {
                }
                frame 2, 4 {
                }
              }
              n111 = call "IMAQ Histograph"("Number of Classes"=w192, "Image"=w193) -> ("Standard  Deviation"=w200:sgl, "Mean Value"=w199:sgl, "Histogram Graph"=→"Waveform Graph":T13)  [unwired: 6 in, 1 out]
              n112 = local write "histogram Standard Deviation"(w200) -> ()
              n113 = local write "histogram Mean"(w199) -> ()
              n114 = local write "Live image setup tab"(w193) -> ()
              n115 = property on="Waveform Graph" class="WFGraph (strict)"("XScale.Maximum"=w192) -> ()  [unwired: 2 in, 2 out]
            }
          }
          frame #3 {
            # "restore tabs"
            n116 = local write "control tab"(T2."main" ("control tab")) -> ()
            n117 = property on="control tab" class="TabCtl (strict)"("Tabs Visible?"=TRUE) -> ()  [unwired: 2 in, 2 out]
          }
        }
        n118 = Delete From Array(array=w146, index=0) -> (deleted portion=w143:T1, array with subset deleted=w144:T1[])  [unwired: 1 in]
        n119 = local write "IR camera session ref"(w129) -> ()
      }
      frame "do scan" {
        # "check if scan is finished"
        n120 = local write "current state ( setup is idle)"(w261) -> ()
        n121 = local read "number of steps"() -> (w260:dbl)
        n122 = local read "step nr"() -> (w255:dbl)
        n123 = Equal To 0?(x=w255) -> (x = 0?=w254:bool)
        n124 = case shown="True" w254 {
          tunnel: w256 -> [_ w264]
          frame False {
          }
          frame True {
            # "reset position array"
            # "reset focus value array"
            # "write temp state array at begin of scan\nto preserve state"
            n125 = local write "temp scan state array"(w264) -> ()
            n126 = local write "contrast value array"(sgl[] [] ("contrast value array")) -> ()
            n127 = local write "real position array"(dbl[] [] ("real position array")) -> ()
          }
        }
        n128 = Less?(x=w255, y=w260) -> (x < y?=w259:bool)
        n129 = case shown="True" w259 {
          tunnel: [w265 w269] -> w258
          tunnel: [wobbe_statemachine."focus calculation" ("Initial State") w268] -> w257
          frame False {
            # "reset counter, do a focus calculation and go resume state array"
            n130 = local write "step nr"(0.0 ("step nr")) -> ()
            n131 = local read "temp scan state array"() -> (w265:T1[])
          }
          frame True {
            n132 = flat-sequence {
              tunnel: [w280] -> w269
              tunnel: [wobbe_statemachine."move to position" ("Initial State")] -> w268
              frame #0 {
                # "calculate next position"
                n133 = local read "start"() -> (w271:dbl)
                n134 = local read "step nr"() -> (w274:dbl)
                n135 = local read "stepsize (mm)"() -> (w273:dbl)
                n136 = Multiply(x=w274, y=w273) -> (x*y=w272:dbl)
                n137 = Add(x=w271, y=w272) -> (x+y=w270:dbl)
                n138 = local write "set position"(w270) -> ()
              }
              frame #1 {
                # "ad step counter"
                n139 = local read "step nr"() -> (w276:dbl)
                n140 = Increment(x=w276) -> (x+1=w275:dbl)
                n141 = local write "step nr"(w275) -> ()
              }
              frame #2 {
                # "do another round"
                n142 = Build Array(wobbe_statemachine."grab picture" ("Initial State"), wobbe_statemachine."write scan time" ("Initial State"), wobbe_statemachine."do scan" ("Initial State")) -> (w280:T1[])
              }
            }
          }
        }
      }
      frame "do test scan" {
        # "check if scan is finished"
        n143 = local read "number of steps"() -> (w289:dbl)
        n144 = local read "step nr"() -> (w284:dbl)
        n145 = Equal To 0?(x=w284) -> (x = 0?=w283:bool)
        n146 = case shown="True" w283 {
          tunnel: w285 -> [_ w293]
          frame False {
          }
          frame True {
            # "reset position array"
            # "reset focus value array"
            # "write temp state array at begin of scan\nto preserve state"
            n147 = local write "temp scan state array"(w293) -> ()
            n148 = local write "contrast value array"(sgl[] [] ("contrast value array")) -> ()
            n149 = local write "real position array"(dbl[] [] ("real position array")) -> ()
          }
        }
        n150 = local write "current state ( setup is idle)"(w290) -> ()
        n151 = Less?(x=w284, y=w289) -> (x < y?=w288:bool)
        n152 = case shown="False" w288 {
          tunnel: [w294 w298] -> w287
          tunnel: [wobbe_statemachine."focus calculation" ("Initial State") w297] -> w286
          frame False {
            # "reset counter, do a focus calculation and go resume state array"
            n153 = local write "step nr"(0.0 ("step nr")) -> ()
            n154 = local read "temp scan state array"() -> (w294:T1[])
          }
          frame True {
            n155 = flat-sequence {
              tunnel: [w309] -> w298
              tunnel: [wobbe_statemachine."move to position" ("Initial State")] -> w297
              frame #0 {
                # "calculate next position"
                n156 = local read "start"() -> (w300:dbl)
                n157 = local read "step nr"() -> (w303:dbl)
                n158 = local read "stepsize (mm)"() -> (w302:dbl)
                n159 = Multiply(x=w303, y=w302) -> (x*y=w301:dbl)
                n160 = Add(x=w300, y=w301) -> (x+y=w299:dbl)
                n161 = local write "set position"(w299) -> ()
              }
              frame #1 {
                # "ad step counter"
                n162 = local read "step nr"() -> (w305:dbl)
                n163 = Increment(x=w305) -> (x+1=w304:dbl)
                n164 = local write "step nr"(w304) -> ()
              }
              frame #2 {
                # "do another round"
                n165 = Build Array(wobbe_statemachine."grab picture without save" ("Initial State"), wobbe_statemachine."write scan time" ("Initial State"), wobbe_statemachine."do test scan" ("Initial State")) -> (w309:T1[])
              }
            }
          }
        }
      }
      frame "do non lin test scan" {
        # "test scan with non lineair steps"
        # "check if scan is finished"
        n166 = local write "current state ( setup is idle)"(w319) -> ()
        n167 = local read "step nr"() -> (w314:dbl)
        n168 = local read "total nr of steps"() -> (w311:dbl)
        n169 = Equal To 0?(x=w314) -> (x = 0?=w313:bool)
        n170 = case shown="True" w313 {
          tunnel: w315 -> [_ w322]
          frame False {
          }
          frame True {
            # "reset position array"
            # "reset focus value array"
            # "write temp state array at begin of scan\nto preserve state"
            n171 = local write "temp scan state array"(w322) -> ()
            n172 = local write "contrast value array"(sgl[] [] ("contrast value array")) -> ()
            n173 = local write "real position array"(dbl[] [] ("real position array")) -> ()
          }
        }
        n174 = Less?(x=w314, y=w311) -> (x < y?=w318:bool)
        n175 = case shown="True" w318 {
          tunnel: [w323 w327] -> w317
          tunnel: [wobbe_statemachine."focus calculation" ("Initial State") w326] -> w316
          frame False {
            # "reset counter, do a focus calculation and  resume state array"
            n176 = local write "step nr"(0.0 ("step nr")) -> ()
            n177 = local read "temp scan state array"() -> (w323:T1[])
          }
          frame True {
            n178 = flat-sequence {
              tunnel: [w371] -> w327
              tunnel: [wobbe_statemachine."move to position" ("Initial State")] -> w326
              frame #0 {
                n179 = local read "rough extra number \nof steps both sides"() -> (w329:dbl)
                n180 = local read "step nr"() -> (w330:dbl)
                n181 = Less?(x=w330, y=w329) -> (x < y?=w328:bool)
                n182 = case shown="False" w328 {
                  frame True {
                    # "calculate next position in start"
                    n183 = local read "rough stepsize (mm)"() -> (w334:dbl)
                    n184 = local read "start"() -> (w332:dbl)
                    n185 = local read "step nr"() -> (w335:dbl)
                    n186 = Multiply(x=w335, y=w334) -> (x*y=w333:dbl)
                    n187 = Add(x=w332, y=w333) -> (x+y=w331:dbl)
                    n188 = local write "set position"(w331) -> ()
                  }
                  frame False {
                    n189 = local read "number of steps"() -> (w338:dbl)
                    n190 = local read "rough extra number \nof steps both sides"() -> (w337:dbl)
                    n191 = local read "step nr"() -> (w339:dbl)
                    n192 = Add(x=w338, y=w337) -> (x+y=w336:dbl)
                    n193 = Less?(x=w339, y=w336) -> (x < y?=w340:bool)
                    n194 = case shown="True" w340 {
                      tunnel: w336 -> [w341 _]
                      frame False {
                        # "calculate last steps rough"
                        n195 = local read "rough extra number \nof steps both sides"() -> (w345:dbl)
                        n196 = local read "rough stepsize (mm)"() -> (w347:dbl)
                        n197 = local read "number of steps"() -> (w349:dbl)
                        n198 = local read "stepsize (mm)"() -> (w350:dbl)
                        n199 = local read "step nr"() -> (w352:dbl)
                        n200 = Multiply(x=w350, y=w349) -> (x*y=w348:dbl)
                        n201 = Subtract(x=w352, y=w341) -> (x-y=w354:dbl)
                        n202 = Multiply(x=w345, y=w347) -> (x*y=w351:dbl)
                        n203 = Multiply(x=w354, y=w347) -> (x*y=w353:dbl)
                        n204 = Add(x=w351, y=w348) -> (x+y=w346:dbl)
                        n205 = Add(x=w346, y=w353) -> (x+y=w344:dbl)
                        n206 = local read "start"() -> (w343:dbl)
                        n207 = Add(x=w343, y=w344) -> (x+y=w342:dbl)
                        n208 = local write "set position"(w342) -> ()
                      }
                      frame True {
                        # "calculate next position in fine scan region"
                        n209 = local read "rough extra number \nof steps both sides"() -> (w355:dbl)
                        n210 = local read "rough extra number \nof steps both sides"() -> (w361:dbl)
                        n211 = local read "step nr"() -> (w362:dbl)
                        n212 = local read "rough stepsize (mm)"() -> (w360:dbl)
                        n213 = local read "stepsize (mm)"() -> (w359:dbl)
                        n214 = Subtract(x=w362, y=w355) -> (x-y=w365:dbl)
                        n215 = Multiply(x=w361, y=w360) -> (x*y=w363:dbl)
                        n216 = Multiply(x=w365, y=w359) -> (x*y=w364:dbl)
                        n217 = Add(x=w363, y=w364) -> (x+y=w358:dbl)
                        n218 = local read "start"() -> (w357:dbl)
                        n219 = Add(x=w357, y=w358) -> (x+y=w356:dbl)
                        n220 = local write "set position"(w356) -> ()
                      }
                    }
                  }
                }
              }
              frame #1 {
                # "ad step counter"
                n221 = local read "step nr"() -> (w367:dbl)
                n222 = Increment(x=w367) -> (x+1=w366:dbl)
                n223 = local write "step nr"(w366) -> ()
              }
              frame #2 {
                # "do another round"
                n224 = Build Array(wobbe_statemachine."grab picture without save" ("Initial State"), wobbe_statemachine."write scan time" ("Initial State"), wobbe_statemachine."do non lin test scan" ("Initial State")) -> (w371:T1[])
              }
            }
          }
        }
      }
      frame "do non lin scan" {
        # "test scan with non lineair steps"
        # "check if scan is finished"
        n225 = local write "current state ( setup is idle)"(w381) -> ()
        n226 = local read "step nr"() -> (w376:dbl)
        n227 = local read "total nr of steps"() -> (w373:dbl)
        n228 = Equal To 0?(x=w376) -> (x = 0?=w375:bool)
        n229 = case shown="True" w375 {
          tunnel: w377 -> [_ w384]
          frame False {
          }
          frame True {
            # "reset position array"
            # "reset focus value array"
            # "write temp state array at begin of scan\nto preserve state"
            n230 = local write "temp scan state array"(w384) -> ()
            n231 = local write "contrast value array"(sgl[] [] ("contrast value array")) -> ()
            n232 = local write "real position array"(dbl[] [] ("real position array")) -> ()
          }
        }
        n233 = Less?(x=w376, y=w373) -> (x < y?=w380:bool)
        n234 = case shown="True" w380 {
          tunnel: [w385 w391] -> w379
          tunnel: [wobbe_statemachine."focus calculation" ("Initial State") w390] -> w378
          frame False {
            # "reset counter, do a focus calculation and  resume state array"
            n235 = local write "step nr"(0.0 ("step nr")) -> ()
            n236 = local read "temp scan state array"() -> (w385:T1[])
          }
          frame True {
            n237 = flat-sequence {
              tunnel: [w392] -> w388
              tunnel: [w434] -> w389
              tunnel: w388 -> [w434]
              tunnel: [w439] -> w391
              tunnel: [w438] -> w390
              tunnel: w389 -> [w437]
              frame #0 {
                n238 = local read "rough extra number \nof steps both sides"() -> (w394:dbl)
                n239 = local read "step nr"() -> (w395:dbl)
                n240 = Less?(x=w395, y=w394) -> (x < y?=w393:bool)
                n241 = case shown="False" w393 {
                  tunnel: [FALSE w402] -> w392
                  frame True {
                    # "first"
                    # "calculate next position in start"
                    n242 = local read "rough stepsize (mm)"() -> (w400:dbl)
                    n243 = local read "start"() -> (w398:dbl)
                    n244 = local read "step nr"() -> (w401:dbl)
                    n245 = Multiply(x=w401, y=w400) -> (x*y=w399:dbl)
                    n246 = Add(x=w398, y=w399) -> (x+y=w397:dbl)
                    n247 = local write "set position"(w397) -> ()
                  }
                  frame False {
                    n248 = local read "number of steps"() -> (w405:dbl)
                    n249 = local read "rough extra number \nof steps both sides"() -> (w404:dbl)
                    n250 = local read "step nr"() -> (w406:dbl)
                    n251 = Add(x=w405, y=w404) -> (x+y=w403:dbl)
                    n252 = Less?(x=w406, y=w403) -> (x < y?=w407:bool)
                    n253 = case shown="True" w407 {
                      tunnel: w403 -> [w409 _]
                      tunnel: [FALSE TRUE] -> w402
                      frame False {
                        # "calculate last steps rough"
                        n254 = local read "rough extra number \nof steps both sides"() -> (w410:dbl)
                        n255 = local read "rough stepsize (mm)"() -> (w415:dbl)
                        n256 = local read "number of steps"() -> (w417:dbl)
                        n257 = local read "stepsize (mm)"() -> (w418:dbl)
                        n258 = local read "step nr"() -> (w420:dbl)
                        n259 = Multiply(x=w418, y=w417) -> (x*y=w416:dbl)
                        n260 = Subtract(x=w420, y=w409) -> (x-y=w422:dbl)
                        n261 = Multiply(x=w410, y=w415) -> (x*y=w419:dbl)
                        n262 = Multiply(x=w422, y=w415) -> (x*y=w421:dbl)
                        n263 = Add(x=w419, y=w416) -> (x+y=w414:dbl)
                        n264 = Add(x=w414, y=w421) -> (x+y=w413:dbl)
                        n265 = local read "start"() -> (w412:dbl)
                        n266 = Add(x=w412, y=w413) -> (x+y=w411:dbl)
                        n267 = local write "set position"(w411) -> ()
                      }
                      frame True {
                        # "calculate next position in fine scan region"
                        n268 = local read "rough extra number \nof steps both sides"() -> (w429:dbl)
                        n269 = local read "step nr"() -> (w430:dbl)
                        n270 = local read "rough stepsize (mm)"() -> (w428:dbl)
                        n271 = local read "stepsize (mm)"() -> (w427:dbl)
                        n272 = Subtract(x=w430, y=w429) -> (x-y=w433:dbl)
                        n273 = Multiply(x=w429, y=w428) -> (x*y=w431:dbl)
                        n274 = Multiply(x=w433, y=w427) -> (x*y=w432:dbl)
                        n275 = Add(x=w431, y=w432) -> (x+y=w426:dbl)
                        n276 = local read "start"() -> (w425:dbl)
                        n277 = Add(x=w425, y=w426) -> (x+y=w424:dbl)
                        n278 = local write "set position"(w424) -> ()
                      }
                    }
                  }
                }
              }
              frame #1 {
                # "ad step counter"
                n279 = local read "step nr"() -> (w436:dbl)
                n280 = Increment(x=w436) -> (x+1=w435:dbl)
                n281 = local write "step nr"(w435) -> ()
              }
              frame #2 {
                n282 = case shown="True" w437 {
                  tunnel: [w443 w448] -> w439
                  tunnel: [wobbe_statemachine."move to position" ("Initial State") wobbe_statemachine."move to position" ("Initial State")] -> w438
                  frame True {
                    # "do another round"
                    n283 = Build Array(wobbe_statemachine."grab picture" ("Initial State"), wobbe_statemachine."write scan time" ("Initial State"), wobbe_statemachine."do non lin scan" ("Initial State")) -> (w443:T1[])
                  }
                  frame False {
                    # "do another round\nwithout saving pic"
                    n284 = Build Array(wobbe_statemachine."grab picture without save" ("Initial State"), wobbe_statemachine."write scan time" ("Initial State"), wobbe_statemachine."do non lin scan" ("Initial State")) -> (w448:T1[])
                  }
                }
              }
            }
          }
        }
      }
      frame "do multi point scan " {
        # "do several repetive  scans with timing settings"
        # "check if scan is finished"
        n285 = local write "current state ( setup is idle)"(w458) -> ()
        n286 = local read "rep nr"() -> (w452:i32)
        n287 = local read "nr of repetitions"() -> (w451:i32)
        n288 = Equal To 0?(x=w452) -> (x = 0?=w450:bool)
        n289 = case shown="True" w450 {
          tunnel: w454 -> [_ w462]
          frame False {
          }
          frame True {
            # "write rep start time"
            # "reset rep nr"
            # "write temp state array at begin of scan\nto preserve state"
            n290 = local write "temp rep scan  state array"(w462) -> ()
            n291 = Get Date/Time In Seconds() -> (seconds since 1Jan1904=→"rep start time 2":timestamp)
            n292 = Tick Count (ms)() -> (millisecond timer value=→"rep start time":u32)
            n293 = local write "rep nr"(0 ("rep nr")) -> ()
          }
        }
        n294 = Less?(x=w452, y=w451) -> (x < y?=w457:bool)
        n295 = case shown="True" w457 {
          tunnel: [w464 w471] -> w456
          tunnel: [w463 w470] -> w455
          tunnel: w450 -> [_ w468]
          frame False {
            # "shift state array \none place"
            # "reset counter, and  resume state array"
            n296 = local read "temp rep scan  state array"() -> (w465:T1[])
            n297 = local write "rep nr"(0 ("rep nr")) -> ()
            n298 = Delete From Array(array=w465, index=0) -> (deleted portion=w463:T1, array with subset deleted=w464:T1[])  [unwired: 1 in]
          }
          frame True {
            n299 = flat-sequence {
              tunnel: [w472] -> w469
              tunnel: w468 -> [w472]
              tunnel: w469 -> [w480]
              tunnel: [w510] -> w471
              tunnel: [wobbe_statemachine."ad curr date and time to save path" ("Initial State")] -> w470
              frame #0 {
                n300 = local read "repetition time [s]"() -> (w475:i64)
                n301 = local read "rep start time"() -> (w478:u32)
                n302 = Multiply(x=w475, y=i64 1000) -> (x*y=w477:i64)
                n303 = Tick Count (ms)() -> (millisecond timer value=w479:u32)
                n304 = Subtract(x=w479, y=w478) -> (x-y=w476:u32)
                n305 = Greater Or Equal?(x=w476, y=w477) -> (x >= y?=→"finished late !\nraise rep time":bool)
              }
              frame #1 {
                # "Rep timer not first time use"
                n306 = case shown="False" w480 {
                  frame False {
                    n307 = while {
                      stop <- w481 stop-if-true
                      n308 = local read "rep start time"() -> (w495:u32)
                      n309 = Get Date/Time In Seconds() -> (seconds since 1Jan1904=w483:timestamp)
                      n310 = local read "last scan time (tabs)"() -> (w493:u32)
                      n311 = local read "repetition time [s]"() -> (w486:i64)
                      n312 = local read "rep start time 2"() -> (w485:timestamp)
                      n313 = Tick Count (ms)() -> (millisecond timer value=w496:u32)
                      n314 = local write "current time 2"(w483) -> ()
                      n315 = local read "rep nr"() -> (w487:i32)
                      n316 = To Double Precision Float(number=w483) -> (double precision float=w488:dbl)
                      n317 = Subtract(x=w496, y=w495) -> (x-y=w492:u32)
                      n318 = Bundle("last scan time (tabs)"=w493, "last scan time (tabs)"=w493, w492) -> (w494:T24)  [unwired: 1 in]
                      n319 = local write "elapsed time bar  (red idle time)"(w494) -> ()
                      n320 = Multiply(x=w487, y=w486) -> (x*y=w484:i64)
                      n321 = Divide(x=w492, y=u32 1000) -> (x/y=w491:dbl)
                      n322 = local write "Elapsed Time (s)"(w491) -> ()
                      n323 = Add(x=w485, y=w484) -> (x+y=w482:timestamp)
                      n324 = property on="timer graph" class="XYGraph (strict)"("Cursor.Cursor X"=w488) -> ()  [unwired: 2 in, 2 out]
                      n325 = Wait (ms)(milliseconds to wait=u32 100) -> ()  [unwired: 1 out]
                      n326 = Greater Or Equal?(x=w483, y=w482) -> (x >= y?=w481:bool)
                    }
                  }
                  frame True {
                    n327 = Wait (ms)(milliseconds to wait=u32 100) -> ()  [unwired: 1 out]
                  }
                }
              }
              frame #2 {
                # "ad rep counter"
                n328 = local read "rep nr"() -> (w501:i32)
                n329 = Get Date/Time In Seconds() -> (seconds since 1Jan1904=w498:timestamp)
                n330 = To Double Precision Float(number=w498) -> (double precision float=w499:dbl)
                n331 = property on="timer graph" class="XYGraph (strict)"("Cursor.Cursor X"=w499) -> ()  [unwired: 2 in, 2 out]
                n332 = Increment(x=w501) -> (x+1=w500:i32)
                n333 = local write "rep nr"(w500) -> ()
              }
              frame #3 {
                # "write rep start time"
                # "do a scan and save pics with scan settings"
                n334 = local read "use nonlin steps"() -> (w507:bool)
                n335 = case shown="False" w507 {
                  tunnel: [wobbe_statemachine."do non lin scan" ("Initial State") wobbe_statemachine."do scan" ("Initial State")] -> w508
                  frame True {
                  }
                  frame False {
                  }
                }
                n336 = Tick Count (ms)() -> (millisecond timer value=w502:u32)
                n337 = local write "rep start time"(w502) -> ()
                n338 = Build Array(wobbe_statemachine."start scan timer" ("Initial State"), w508, wobbe_statemachine."move to start " ("Initial State"), wobbe_statemachine."focus calculation" ("Initial State"), wobbe_statemachine."stop scan timer" ("Initial State"), wobbe_statemachine."do multi point scan " ("Initial State")) -> (w510:T1[])
              }
            }
          }
        }
      }
      frame "ad curr date and time to save path" {
        # "change and name dir before scan"
        # "shift state array \none place"
        n339 = local read "selected path"() -> (w515:path)
        n340 = local write "current state ( setup is idle)"(w526) -> ()
        n341 = Get Date/Time In Seconds() -> (seconds since 1Jan1904=w521:timestamp)
        n342 = Path To String(path=w515) -> (string=w519:string)
        n343 = Format Date/Time String(time format string (%c)="\\%Y%m%d_%H%M%S", seconds (now)=w521) -> (date/time string=w518:string)  [unwired: 1 in]
        n344 = Concatenate Strings(w519, w518) -> (w517:string)
        n345 = Delete From Array(array=w524, index=0) -> (deleted portion=w523:T1, array with subset deleted=w522:T1[])  [unwired: 1 in]
        n346 = String To Path(string=w517) -> (path=w516:path)
        n347 = Create Folder(path (use dialog)=w516) -> (created path=w514:path)  [unwired: 2 in, 2 out]
        n348 = local write "path"(w514) -> ()
      }
      frame "read temp scan array" {
        # "shift state array \none place"
        n349 = local write "current state ( setup is idle)"(w531) -> ()
        n350 = Delete From Array(array=w529, index=0) -> (deleted portion=w528:T1, array with subset deleted=w527:T1[])  [unwired: 1 in]
        n351 = local write "temp rep scan  state array"(w527) -> ()
      }
      frame "write temp scan state array" {
        # "shift state array \none place"
        n352 = local read "temp rep scan  state array"() -> (w532:T1[])
        n353 = local write "current state ( setup is idle)"(w536) -> ()
        n354 = Delete From Array(array=w532, index=0) -> (deleted portion=w534:T1, array with subset deleted=w533:T1[])  [unwired: 1 in]
      }
      frame "simple timer" {
        # "shift state array \none place"
        n355 = local read "start at"() -> (w538:timestamp)
        n356 = Get Date/Time In Seconds() -> (seconds since 1Jan1904=w539:timestamp)
        n357 = Greater?(x=w539, y=w538) -> (0:w537:bool)
        n358 = local write "current state ( setup is idle)"(w545) -> ()
        n359 = Delete From Array(array=w543, index=0) -> (deleted portion=w542:T1, array with subset deleted=w540:T1[])  [unwired: 1 in]
        n360 = case shown="False" w537 {
          tunnel: w542 -> [w548 w558]
          tunnel: [w547 w557] -> w541
          tunnel: w540 -> [w546 w556]
          frame True {
            n361 = flat-sequence {
              tunnel: w548 -> [_]
              tunnel: [w553] -> w549
              tunnel: w546 -> [w552]
              tunnel: w549 -> [w554]
              tunnel: [w554] -> w547
              frame #0 {
                n362 = One Button Dialog(message="Time is in the past !") -> ()  [unwired: 1 in, 1 out]
              }
              frame #1 {
                # "if timer canceled \ngo to last state (caller)"
                n363 = Array Size(array=w552) -> (size(s)=w551:i32)
                n364 = Delete From Array(array=w552, index=w551) -> (deleted portion=w553:T1)  [unwired: 1 in, 1 out]
              }
              frame #2 {
                n365 = local write "start fast timer"(FALSE ("start fast timer")) -> ()
              }
            }
          }
          frame False {
            n366 = flat-sequence {
              tunnel: [w561] -> w560
              tunnel: w558 -> [w571]
              tunnel: [w570] -> w559
              tunnel: w556 -> [w569]
              tunnel: w560 -> [w568]
              tunnel: w559 -> [w576]
              tunnel: [w576] -> w557
              frame #0 {
                n367 = while {
                  tunnel: [w563] -> w561
                  stop <- w565 stop-if-true
                  n368 = local read "start at"() -> (w567:timestamp)
                  n369 = Get Date/Time In Seconds() -> (seconds since 1Jan1904=w562:timestamp)
                  n370 = local read "start fast timer"() -> (w563:bool)
                  n371 = local write "current date and time"(w562) -> ()
                  n372 = Greater?(x=w562, y=w567) -> (0:w566:bool)
                  n373 = local write "current time"(w562) -> ()
                  n374 = Not(x=w563) -> (.not. x?=w564:bool)
                  n375 = Or(x=w566, y=w564) -> (x .or. y?=w565:bool)
                }
              }
              frame #1 {
                n376 = case shown="True" w568 {
                  tunnel: w571 -> [_ w575]
                  tunnel: [w572 w575] -> w570
                  tunnel: w569 -> [w573 _]
                  frame False {
                    # "if timer canceled \ngo to last state (caller)"
                    n377 = Array Size(array=w573) -> (size(s)=w574:i32)
                    n378 = Delete From Array(array=w573, index=w574) -> (deleted portion=w572:T1)  [unwired: 1 in, 1 out]
                  }
                  frame True {
                    # "if timer is done start state array"
                  }
                }
              }
              frame #2 {
                n379 = local write "start fast timer"(FALSE ("start fast timer")) -> ()
              }
            }
          }
        }
      }
      frame "start scan timer" {
        # "reset de start time at start of a scan and writes minimum scale ( now) and maximum scale  ( set scan time )"
        # "shift state array \none place"
        n380 = local write "current state ( setup is idle)"(w587) -> ()
        n381 = local read "repetition time [s]"() -> (w582:i64)
        n382 = Delete From Array(array=w585, index=0) -> (deleted portion=w584:T1, array with subset deleted=w583:T1[])  [unwired: 1 in]
        n383 = Tick Count (ms)() -> (millisecond timer value=w580:u32)
        n384 = local write "start time"(w580) -> ()
        n385 = Multiply(x=w582, y=i64 1000) -> (x*y=w578:i64)
        n386 = property on="elapsed time bar  (red idle time)" class="Slide (strict)"("Scale.Minimum"=0.0 ("Scale.Range:Minimum"), "Scale.Maximum"=w578) -> ()  [unwired: 2 in, 2 out]
      }
      frame "write scan time" {
        # "increase the time bar and writes the elapsed time"
        # "shift state array \none place"
        n387 = local write "current state ( setup is idle)"(w599) -> ()
        n388 = local read "start time"() -> (w589:u32)
        n389 = local read "last scan time (tabs)"() -> (w591:u32)
        n390 = Tick Count (ms)() -> (millisecond timer value=w590:u32)
        n391 = Subtract(x=w590, y=w589) -> (x-y=w588:u32)
        n392 = Delete From Array(array=w597, index=0) -> (deleted portion=w596:T1, array with subset deleted=w595:T1[])  [unwired: 1 in]
        n393 = Divide(x=w588, y=u32 1000) -> (x/y=w592:dbl)
        n394 = Bundle("last scan time (tabs)"=w591, w588, w588) -> (w594:cluster{"last scan time (tabs)":u32, u32, u32})  [unwired: 1 in]
        n395 = local write "elapsed time bar  (red idle time)"(w594) -> ()
        n396 = local write "Elapsed Time (s)"(w592) -> ()
      }
      frame "stop scan timer" {
        # "writes the last scantime to an indicator"
        # "shift state array \none place"
        n397 = local write "current state ( setup is idle)"(w611) -> ()
        n398 = local read "start time"() -> (w603:u32)
        n399 = local read "last scan time (tabs)"() -> (w601:u32)
        n400 = Delete From Array(array=w609, index=0) -> (deleted portion=w608:T1, array with subset deleted=w607:T1[])  [unwired: 1 in]
        n401 = Tick Count (ms)() -> (millisecond timer value=w604:u32)
        n402 = Subtract(x=w604, y=w603) -> (x-y=w600:u32)
        n403 = Bundle("last scan time (tabs)"=w601, w600, w600) -> (w602:cluster{"last scan time (tabs)":u32, u32, u32})  [unwired: 1 in]
        n404 = Divide(x=w600, y=u32 1000) -> (x/y=w605:dbl)
        n405 = local write "Last scan time (s)"(w605) -> ()
        n406 = local write "elapsed time bar  (red idle time)"(w602) -> ()
      }
      frame "select save path" {
        # "select main directory for scan data"
        # "shift state array \none place"
        n407 = Delete From Array(array=w615, index=0) -> (deleted portion=w614:T1, array with subset deleted=w613:T1[])  [unwired: 1 in]
        n408 = local write "current state ( setup is idle)"(w612) -> ()
        n409 = call "File Dialog"() -> ("selected path"=w617:path)  [unwired: 12 in, 3 out]
        n410 = local write "selected path"(w617) -> ()
      }
      frame "plight" {
        # "switch the plant lightning"
        # "shift state array \none place"
        n411 = Delete From Array(array=w622, index=0) -> (deleted portion=w621:T1, array with subset deleted=w620:T1[])  [unwired: 1 in]
        n412 = local write "current state ( setup is idle)"(w619) -> ()
        n413 = local read "testrun without daq"() -> (w618:bool)
        n414 = case shown="False" w618 {
          frame False {
            # "set the intensity of the plant light"
            n415 = local read "plight [%]"() -> (w628:i32)
            n416 = Divide(x=w628, y=100) -> (x/y=w625:dbl)
            n417 = Multiply(x=w625, y="plight 100% voltage") -> (x*y=w626:dbl)
            n418 = local write "plant light %"(w628) -> ()
            n419 = call-poly <vilib>:"DAQmx Write.vi"("task/channels in"=refnum<k21> "plantlight(red)", "data"=w626) -> ()  [unwired: 11 in, 3 out]
          }
          frame True {
          }
        }
      }
      frame "bluepsilight" {
        # "switch the plant lightning with the PSI module for the blue channel"
        # "shift state array \none place"
        n420 = Delete From Array(array=w634, index=0) -> (deleted portion=w633:T1, array with subset deleted=w632:T1[])  [unwired: 1 in]
        n421 = local write "current state ( setup is idle)"(w631) -> ()
        n422 = local read "testrun without psi light"() -> (w630:bool)
        n423 = case shown="False" w630 {
          frame False {
            # "set the intensity of the psi plant light and set the on/off state"
            n424 = local read "blue"() -> (w639:bool)
            n425 = local read "blue"() -> (w642:dbl)
            n426 = case shown="False" w639 {
              tunnel: ["ST\u0010\u00028\u0000-" ("write buffer") "ST\u0010\u00028\u0001," ("write buffer")] -> w636
              frame False {
                # "switch blue channel off"
              }
              frame True {
                # "switch blue channel on"
              }
            }
            n427 = Multiply(x=w642, y=10.22) -> (x*y=w643:dbl)
            n428 = call "power command.vi"("channel"=chan_select."blue", "power [0-1022]"=w643) -> ("resulting string incl crc"=w641:string)
            n429 = local read "serial psi channel"() -> (w640:refnum<visa-resource-name>)
            n430 = VISA Write(VISA resource name=w640, write buffer=w641) -> (VISA resource name out=w638:refnum<visa-resource-name>)  [unwired: 1 in, 2 out]
            n431 = VISA Write(VISA resource name=w638, write buffer=w636) -> (VISA resource name out=w637:refnum<visa-resource-name>)  [unwired: 1 in, 2 out]
            n432 = VISA Close(VISA resource name=w637) -> ()  [unwired: 1 in, 1 out]
          }
          frame True {
          }
        }
      }
      frame "greenpsilight" {
        # "switch the plant lightning with the PSI module for the green channel"
        # "shift state array \none place"
        n433 = Delete From Array(array=w652, index=0) -> (deleted portion=w651:T1, array with subset deleted=w650:T1[])  [unwired: 1 in]
        n434 = local write "current state ( setup is idle)"(w649) -> ()
        n435 = local read "testrun without psi light"() -> (w648:bool)
        n436 = case shown="False" w648 {
          frame False {
            # "set the intensity of the psi plant light and set the on/off state"
            n437 = local read "green"() -> (w660:dbl)
            n438 = local read "green"() -> (w657:bool)
            n439 = case shown="True" w657 {
              tunnel: ["ST\u0010\u0002\u0018\u0000\r" ("write buffer") "ST\u0010\u0002\u0018\u0001\f" ("write buffer")] -> w654
              frame False {
                # "switch green channel off"
              }
              frame True {
                # "switch green channel on"
              }
            }
            n440 = Multiply(x=w660, y=10.22) -> (x*y=w661:dbl)
            n441 = call "power command.vi"("channel"=chan_select."green", "power [0-1022]"=w661) -> ("resulting string incl crc"=w659:string)
            n442 = local read "serial psi channel"() -> (w658:refnum<visa-resource-name>)
            n443 = VISA Write(VISA resource name=w658, write buffer=w659) -> (VISA resource name out=w656:refnum<visa-resource-name>)  [unwired: 1 in, 2 out]
            n444 = VISA Write(VISA resource name=w656, write buffer=w654) -> (VISA resource name out=w655:refnum<visa-resource-name>)  [unwired: 1 in, 2 out]
            n445 = VISA Close(VISA resource name=w655) -> ()  [unwired: 1 in, 1 out]
          }
          frame True {
          }
        }
      }
      frame "redpsilight" {
        # "switch the plant lightning with the PSI module for the red channel"
        # "shift state array \none place"
        n446 = Delete From Array(array=w670, index=0) -> (deleted portion=w669:T1, array with subset deleted=w668:T1[])  [unwired: 1 in]
        n447 = local write "current state ( setup is idle)"(w667) -> ()
        n448 = local read "testrun without psi light"() -> (w666:bool)
        n449 = case shown="False" w666 {
          frame False {
            # "set the intensity of the psi plant light and set the on/off state"
            n450 = local read "red"() -> (w672:bool)
            n451 = local read "red"() -> (w678:dbl)
            n452 = case shown="True" w672 {
              tunnel: ["ST\u0010\u00028\u0000-" ("write buffer") "ST\u0010\u00028\u0001," ("write buffer")] -> w673
              frame False {
                # "switch red channel off"
              }
              frame True {
                # "switch red channel on"
              }
            }
            n453 = Multiply(x=w678, y=10.22) -> (x*y=w679:dbl)
            n454 = call "power command.vi"("channel"=chan_select."red", "power [0-1022]"=w679) -> ("resulting string incl crc"=w677:string)
            n455 = local read "serial psi channel"() -> (w676:refnum<visa-resource-name>)
            n456 = VISA Write(VISA resource name=w676, write buffer=w677) -> (VISA resource name out=w675:refnum<visa-resource-name>)  [unwired: 1 in, 2 out]
            n457 = VISA Write(VISA resource name=w675, write buffer=w673) -> (VISA resource name out=w674:refnum<visa-resource-name>)  [unwired: 1 in, 2 out]
            n458 = VISA Close(VISA resource name=w674) -> ()  [unwired: 1 in, 1 out]
          }
          frame True {
          }
        }
      }
      frame "Minipam pulse" {
        # "exec minipam pulse"
        # "shift state array \none place"
        n459 = Delete From Array(array=w688, index=0) -> (deleted portion=w687:T1, array with subset deleted=w686:T1[])  [unwired: 1 in]
        n460 = local read "testrun without minipam"() -> (w684:bool)
        n461 = local write "current state ( setup is idle)"(w685) -> ()
        n462 = case shown="False" w684 {
          frame False {
            # "mini pam pulse program"
            n463 = call "minipampulse.vi"() -> ()  [unwired: 12 in]
          }
          frame True {
          }
        }
      }
      frame "mlight" {
        # "switch the miroscope lightning"
        # "shift state array \none place"
        n464 = Delete From Array(array=w694, index=0) -> (deleted portion=w693:T1, array with subset deleted=w692:T1[])  [unwired: 1 in]
        n465 = local write "current state ( setup is idle)"(w691) -> ()
        n466 = local read "testrun without daq"() -> (w690:bool)
        n467 = case shown="False" w690 {
          frame False {
            # "switch on or off the microscope light"
            n468 = local read "mlight [%]"() -> (w696:i32)
            n469 = case shown="0" w696 {
              frame 5, Default {
                n470 = call-poly <vilib>:"DAQmx Write.vi"("task/channels in"=refnum<k21> "ringlight(blue)", "data"=0.0) -> ()  [unwired: 11 in, 3 out]
              }
              frame 0 {
                n471 = local write "Microscope light on/off"(FALSE ("Micorcope light on/off")) -> ()
                n472 = call-poly <vilib>:"DAQmx Write.vi"("task/channels in"=refnum<k21> "ringlight(blue)", "data"=0.0) -> ()  [unwired: 11 in, 3 out]
              }
              frame 100 {
                n473 = local write "Microscope light on/off"(TRUE ("Micorcope light on/off")) -> ()
                n474 = call-poly <vilib>:"DAQmx Write.vi"("task/channels in"=refnum<k21> "ringlight(blue)", "data"=5.0) -> ()  [unwired: 11 in, 3 out]
              }
            }
          }
          frame True {
          }
        }
      }
      frame "move to position" {
        # "shift state array \none place"
        n475 = local read "testrun without motor"() -> (w705:bool)
        n476 = case shown="False" w705 {
          tunnel: w711 -> [w716 w750]
          tunnel: [w715 w749] -> w710
          frame True {
            n477 = flat-sequence {
              tunnel: w716 -> [w720]
              tunnel: [w721] -> w719
              tunnel: [w720] -> w713
              tunnel: [w723] -> w718
              tunnel: w719 -> [w722]
              tunnel: [w722] -> w717
              tunnel: w713 -> [w723]
              tunnel: [w732] -> w715
              tunnel: w718 -> [w733]
              tunnel: w717 -> [w734]
              tunnel: [w724] -> w714
              frame #0 {
                # "move stage to position"
                n478 = local read "set position"() -> (w721:dbl)
              }
              frame #1 {
              }
              frame #2 {
                # "create filename with pos and time"
                # "check if stage position is within offset range"
                n479 = while {
                  shift-right: [w739] -> w732
                  shift-left: w733 -> [w739]
                  tunnel: [w738] -> w735
                  tunnel: [w741] -> w737
                  tunnel: w734 -> [w738]
                  tunnel: [w738] -> w726
                  stop <- w744 stop-if-true
                  n480 = Wait (ms)(milliseconds to wait=u32 100) -> ()  [unwired: 1 out]
                  n481 = Add(x=w738, y="max alowed offset") -> (x+y=w743:dbl)
                  n482 = Subtract(x=w738, y="max alowed offset") -> (x-y=w742:dbl)
                  n483 = In Range and Coerce(upper limit=w743, x=w738, lower limit=w742) -> (In Range?=w744:bool)  [unwired: 1 out]
                  n484 = Get Date/Time In Seconds() -> (seconds since 1Jan1904=w741:timestamp)
                  "real position" <- w738
                }
                n485 = Format Date/Time String(time format string (%c)="%Y%m%d_%H%M%S%1u_pos", seconds (now)=w737) -> (date/time string=w730:string)  [unwired: 1 in]
                n486 = local read "real position array"() -> (w727:dbl[])
                n487 = Number To Fractional String(number=w735) -> (F-format string=w731:string)  [unwired: 3 in]
                n488 = Build Array (concatenate)(w727, w726) -> (→"real position array":dbl[])
                n489 = Concatenate Strings(w730, w731, ".tiff" ("string")) -> (w728:string)
                n490 = local write "Filename with position"(w728) -> ()
                n491 = local read "Motor device ref"() -> (w724:refnum<k24>)
              }
            }
            n492 = local write "Motor device ref"(w714) -> ()
          }
          frame False {
            n493 = flat-sequence {
              tunnel: w750 -> [w761]
              tunnel: [w755] -> w754
              tunnel: [w757] -> w747
              tunnel: [w756] -> w746
              tunnel: [w783] -> w753
              tunnel: w754 -> [w782]
              tunnel: [w782] -> w752
              tunnel: [w781] -> w751
              tunnel: w747 -> [w783]
              tunnel: w746 -> [w781]
              tunnel: [w793] -> w749
              tunnel: w753 -> [w794]
              tunnel: w752 -> [w795]
              tunnel: w751 -> [w792]
              tunnel: [w788] -> w748
              frame #0 {
                # "move stage to position"
                n494 = local read "set position"() -> (w755:dbl)
                n495 = local read "Motor device ref"() -> (w763:refnum<k24>)
                n496 = invoke class="KCubeDCServo" method="SetMoveAbsolutePosition"(reference=w763, error in=w761, "position"=w755) -> (reference out=w765:refnum<k24>, error out=w764:errorcluster)  [unwired: 1 in, 2 out]
                n497 = invoke class="KCubeDCServo" method="MoveAbsolute"(reference=w765, error in=w764, "waitTimeout"=0) -> (reference out=w760:refnum<k24>, error out=w758:errorcluster)  [unwired: 1 in, 2 out]
                n498 = Unbundle By Name(w758) -> ("status"=w759:bool)
                "move error" <- w759
                n499 = case shown="True" w759 {
                  tunnel: w760 -> [w767 w772]
                  tunnel: w758 -> [w766 w771]
                  tunnel: [w766 w769] -> w757
                  tunnel: [w767 w768] -> w756
                  tunnel: w755 -> [_ w770]
                  frame False {
                  }
                  frame True {
                    n500 = while {
                      tunnel: w772 -> [w777]
                      tunnel: w771 -> [_]
                      tunnel: w770 -> [w776]
                      tunnel: [w774] -> w769
                      tunnel: [w775] -> w768
                      stop <- w773 continue-if-true
                      n501 = invoke class="KCubeDCServo" method="SetMoveAbsolutePosition"(reference=w777, "position"=w776) -> (reference out=w780:refnum<k24>, error out=w779:errorcluster)  [unwired: 2 in, 2 out]
                      n502 = invoke class="KCubeDCServo" method="MoveAbsolute"(reference=w780, error in=w779, "waitTimeout"=0) -> (reference out=w775:refnum<k24>, error out=w774:errorcluster)  [unwired: 1 in, 2 out]
                      n503 = Unbundle By Name(w774) -> ("status"=w773:bool)
                      n504 = local write "move error"(w773) -> ()
                    }
                  }
                }
              }
              frame #1 {
              }
              frame #2 {
                # "create filename with pos and time"
                # "check if stage position is within offset range"
                n505 = while {
                  shift-right: [w812] -> w788
                  shift-left: w792 -> [w809]
                  shift-right: [w811] -> w793
                  shift-left: w794 -> [w810]
                  tunnel: [w799] -> w796
                  tunnel: [w802] -> w798
                  tunnel: w795 -> [w801]
                  tunnel: [w799] -> w786
                  stop <- w805 stop-if-true
                  n506 = local read "max alowed offset"() -> (w800:dbl)
                  n507 = Wait (ms)(milliseconds to wait=u32 100) -> ()  [unwired: 1 out]
                  n508 = invoke class="KCubeDCServo" method="GetPositionCounter"(reference=w809, error in=w810) -> (reference out=w812:refnum<k24>, error out=w811:errorcluster, "GetPositionCounter"=w807:i32)  [unwired: 1 in]
                  n509 = Add(x=w801, y=w800) -> (x+y=w804:dbl)
                  n510 = Subtract(x=w801, y=w800) -> (x-y=w803:dbl)
                  n511 = Divide(x=w807, y="encoder counts/rev") -> (x/y=w799:dbl)
                  n512 = In Range and Coerce(upper limit=w804, x=w799, lower limit=w803) -> (In Range?=w805:bool)  [unwired: 1 out]
                  n513 = Get Date/Time In Seconds() -> (seconds since 1Jan1904=w802:timestamp)
                  n514 = local write "real position"(w799) -> ()
                }
                n515 = Format Date/Time String(time format string (%c)="%Y%m%d_%H%M%S%1u_pos", seconds (now)=w798) -> (date/time string=w790:string)  [unwired: 1 in]
                n516 = local read "real position array"() -> (w784:dbl[])
                n517 = Number To Fractional String(number=w796) -> (F-format string=w791:string)  [unwired: 3 in]
                n518 = Build Array (concatenate)(w784, w786) -> (w785:dbl[])
                n519 = Concatenate Strings(w790, w791, ".tiff" ("string")) -> (w787:string)
                n520 = local write "Filename with position"(w787) -> ()
                n521 = local write "real position array"(w785) -> ()
              }
            }
            n522 = local write "Motor device ref"(w748) -> ()
          }
        }
        n523 = local write "current state ( setup is idle)"(w712) -> ()
        n524 = Delete From Array(array=w708, index=0) -> (deleted portion=w706:T1, array with subset deleted=w707:T1[])  [unwired: 1 in]
      }
      frame "grab picture" {
        w830 = T23 7 items=["Grayscale (U8)", "Grayscale (I16)", "Grayscale (SGL)", "Complex (CSG)", "RGB (U32)", "HSL (U32)", "RGB (U64)", "Grayscale (U16)"] ("Image Type")
        # "grab and save picture"
        # "find edges for focus value"
        # "filename = time +pos"
        # "shift state array \none place"
        n525 = local read "Filename with position"() -> (w817:string)
        n526 = local read "path"() -> (w819:path)
        n527 = local write "current state ( setup is idle)"(w841) -> ()
        n528 = Delete From Array(array=w839, index=0) -> (deleted portion=w838:T1, array with subset deleted=w837:T1[])  [unwired: 1 in]
        n529 = local read "Live image mem loc"() -> (w835:T8)
        n530 = Build Path(base path=w819, name or relative path=w817) -> (appended path=w818:path)
        n531 = local read "IR camera session ref"() -> (w836:T6)
        n532 = call <vilib>:"IMAQdx Grab2.vi"("error in"=w833, "Image In"=w835, "Session In"=w836) -> ("error out"=w828:errorcluster, "Image Out"=w829:T8, "Session Out"=w834:T6)  [unwired: 5 in, 1 out]
        n533 = local write "IR camera session ref"(w834) -> ()
        n534 = call-poly "IMAQ Write File 2"("error in (no error)"=w828, "TIFF Options"="TIFF Options", "File Path"=w818, "Image"=w829) -> ("error out"=w827:errorcluster)  [unwired: 6 in, 1 out]
        n535 = local write "Live image setup tab"(w829) -> ()
        n536 = local write "Live image camera tab"(w829) -> ()
        n537 = call "IMAQ Cast Image"("Image Type"=w830, "error in (no error)"=w827, "Image Src"=w829) -> ("error out"=w826:errorcluster, "Image Dst Out"=w814:T8)  [unwired: 7 in]
        n538 = local read "filtered image mem loc"() -> (w823:T8)
        n539 = local read "use ROI"() -> (w816:bool)
        n540 = case shown="True" w816 {
          tunnel: [_ w842] -> w813
          frame False {
          }
          frame True {
            n541 = local read "ROI Mask mem loc"() -> (w842:T8)
          }
        }
        n542 = case shown="\"Convolution\", Default" "edge detection settings" {
          tunnel: w814 -> [w848 w855 w862 w869 w876 w883 w890]
          tunnel: w826 -> [w847 w854 w861 w868 w875 w882 w889]
          tunnel: w823 -> [w846 w856 w863 w870 w877 w884 w891]
          tunnel: [w845 w851 w858 w865 w872 w879 w886] -> w824
          tunnel: [w844 w852 w859 w866 w873 w880 w887] -> w815
          tunnel: w813 -> [w843 w850 w857 w864 w871 w878 w885]
          frame "Convolution", Default {
            n543 = call "IMAQ Convolute"("Kernel"=sgl[][] [[0.0, -1.0, 0.0], [-1.0, 0.0, 1.0], [0.0, 1.0, 0.0]], "error in (no error)"=w847, "Image Dst"=w846, "Image Mask"=w843, "Image Src"=w848) -> ("error out"=w845:errorcluster, "Image Dst Out"=w844:T8)  [unwired: 5 in]
          }
          frame "Differentiation" {
            n544 = call "IMAQ EdgeDetection"("Method"=T18."Differentiation", "error in (no error)"=w854, "Image Dst"=w856, "Image Mask"=w850, "Image Src"=w855) -> ("error out"=w851:errorcluster, "Image Dst Out"=w852:T8)  [unwired: 5 in]
          }
          frame "Gradient" {
            n545 = call "IMAQ EdgeDetection"("Method"=T18."Gradient", "error in (no error)"=w861, "Image Dst"=w863, "Image Mask"=w857, "Image Src"=w862) -> ("error out"=w858:errorcluster, "Image Dst Out"=w859:T8)  [unwired: 5 in]
          }
          frame "Prewitt" {
            n546 = call "IMAQ EdgeDetection"("Method"=T18."Prewitt", "error in (no error)"=w868, "Image Dst"=w870, "Image Mask"=w864, "Image Src"=w869) -> ("error out"=w865:errorcluster, "Image Dst Out"=w866:T8)  [unwired: 5 in]
          }
          frame "Roberts" {
            n547 = call "IMAQ EdgeDetection"("Method"=T18."Roberts", "error in (no error)"=w875, "Image Dst"=w877, "Image Mask"=w871, "Image Src"=w876) -> ("error out"=w872:errorcluster, "Image Dst Out"=w873:T8)  [unwired: 5 in]
          }
          frame "Sigma" {
            n548 = call "IMAQ EdgeDetection"("Method"=T18."Sigma", "error in (no error)"=w882, "Image Dst"=w884, "Image Mask"=w878, "Image Src"=w883) -> ("error out"=w879:errorcluster, "Image Dst Out"=w880:T8)  [unwired: 5 in]
          }
          frame "Sobel" {
            n549 = call "IMAQ EdgeDetection"("Method"=T18."Sobel", "error in (no error)"=w889, "Image Dst"=w891, "Image Mask"=w885, "Image Src"=w890) -> ("error out"=w886:errorcluster, "Image Dst Out"=w887:T8)  [unwired: 5 in]
          }
        }
        n550 = local read "contrast value array"() -> (w820:sgl[])
        n551 = call "IMAQ Histograph"("error in (no error)"=w824, "Image Mask"=w813, "Image"=w815) -> ("error out"=w825:errorcluster, "Mean Value"=w822:sgl)  [unwired: 5 in, 2 out]
        "contrast value \n( high is better)" <- w822
        n552 = Build Array (concatenate)(w820, w822) -> (→"contrast value array":sgl[])
      }
      frame "grab picture without save" {
        w906 = T23 7 items=["Grayscale (U8)", "Grayscale (I16)", "Grayscale (SGL)", "Complex (CSG)", "RGB (U32)", "HSL (U32)", "RGB (U64)", "Grayscale (U16)"] ("Image Type")
        # "grab picture"
        # "find edges for focus value"
        # "shift state array \none place"
        n553 = local read "IR camera session ref"() -> (w910:T6)
        n554 = local read "Live image mem loc"() -> (w909:T8)
        n555 = local write "current state ( setup is idle)"(w915) -> ()
        n556 = call <vilib>:"IMAQdx Grab2.vi"("error in"=w907, "Image In"=w909, "Session In"=w910) -> ("error out"=w898:errorcluster, "Image Out"=w899:T8, "Session Out"=w908:T6)  [unwired: 5 in, 1 out]
        n557 = local write "IR camera session ref"(w908) -> ()
        n558 = Delete From Array(array=w913, index=0) -> (deleted portion=w912:T1, array with subset deleted=w911:T1[])  [unwired: 1 in]
        n559 = local write "Live image setup tab"(w899) -> ()
        n560 = call "IMAQ Cast Image"("Image Type"=w906, "error in (no error)"=w898, "Image Src"=w899) -> ("error out"=w904:errorcluster, "Image Dst Out"=w892:T8)  [unwired: 7 in]
        n561 = local write "Live image camera tab"(w899) -> ()
        n562 = local read "filtered image mem loc"() -> (w901:T8)
        n563 = local read "use ROI"() -> (w894:bool)
        n564 = local read "edge detection settings"() -> (w896:T4)
        n565 = case shown="True" w894 {
          tunnel: [_ w916] -> w893
          frame False {
          }
          frame True {
            n566 = local read "ROI Mask mem loc"() -> (w916:T8)
          }
        }
        n567 = case shown="\"Convolution\", Default" w896 {
          tunnel: w892 -> [w922 w929 w936 w943 w950 w957 w964]
          tunnel: w904 -> [w921 w928 w935 w942 w949 w956 w963]
          tunnel: w901 -> [w920 w930 w937 w944 w951 w958 w965]
          tunnel: [w919 w925 w932 w939 w946 w953 w960] -> w902
          tunnel: [w918 w926 w933 w940 w947 w954 w961] -> w905
          tunnel: w893 -> [w917 w924 w931 w938 w945 w952 w959]
          frame "Convolution", Default {
            n568 = call "IMAQ Convolute"("Kernel"=sgl[][] [[0.0, -1.0, 0.0], [-1.0, 0.0, 1.0], [0.0, 1.0, 0.0]], "error in (no error)"=w921, "Image Dst"=w920, "Image Mask"=w917, "Image Src"=w922) -> ("error out"=w919:errorcluster, "Image Dst Out"=w918:T8)  [unwired: 5 in]
          }
          frame "Differentiation" {
            n569 = call "IMAQ EdgeDetection"("Method"=T18."Differentiation", "error in (no error)"=w928, "Image Dst"=w930, "Image Mask"=w924, "Image Src"=w929) -> ("error out"=w925:errorcluster, "Image Dst Out"=w926:T8)  [unwired: 5 in]
          }
          frame "Gradient" {
            n570 = call "IMAQ EdgeDetection"("Method"=T18."Gradient", "error in (no error)"=w935, "Image Dst"=w937, "Image Mask"=w931, "Image Src"=w936) -> ("error out"=w932:errorcluster, "Image Dst Out"=w933:T8)  [unwired: 5 in]
          }
          frame "Prewitt" {
            n571 = call "IMAQ EdgeDetection"("Method"=T18."Prewitt", "error in (no error)"=w942, "Image Dst"=w944, "Image Mask"=w938, "Image Src"=w943) -> ("error out"=w939:errorcluster, "Image Dst Out"=w940:T8)  [unwired: 5 in]
          }
          frame "Roberts" {
            n572 = call "IMAQ EdgeDetection"("Method"=T18."Roberts", "error in (no error)"=w949, "Image Dst"=w951, "Image Mask"=w945, "Image Src"=w950) -> ("error out"=w946:errorcluster, "Image Dst Out"=w947:T8)  [unwired: 5 in]
          }
          frame "Sigma" {
            n573 = call "IMAQ EdgeDetection"("Method"=T18."Sigma", "error in (no error)"=w956, "Image Dst"=w958, "Image Mask"=w952, "Image Src"=w957) -> ("error out"=w953:errorcluster, "Image Dst Out"=w954:T8)  [unwired: 5 in]
          }
          frame "Sobel" {
            n574 = call "IMAQ EdgeDetection"("Method"=T18."Sobel", "error in (no error)"=w963, "Image Dst"=w965, "Image Mask"=w959, "Image Src"=w964) -> ("error out"=w960:errorcluster, "Image Dst Out"=w961:T8)  [unwired: 5 in]
          }
        }
        n575 = local read "contrast value array"() -> (w900:sgl[])
        n576 = call "IMAQ Histograph"("error in (no error)"=w902, "Image Mask"=w893, "Image"=w905) -> ("error out"=w903:errorcluster, "Mean Value"=w897:sgl)  [unwired: 5 in, 2 out]
        n577 = local write "contrast value \n( high is better)"(w897) -> ()
        n578 = Build Array (concatenate)(w900, w897) -> (w895:sgl[])
        n579 = local write "contrast value array"(w895) -> ()
      }
      frame "set roi" {
        w976 = T25 {"Left"=1230, "Top"=1050, "Right"=1430, "Bottom"=1250, "Rotation"=0.0}  # Default Rectangle
        w975 = i32[] [2] items=["No  event", "Click event", "Draw event", "Move event", "Size event", "Scroll event", "Activate event", "Close event", "Double click event"] ("Events list (all)")
        # "Initialize ROI to default"
        # "When a \"draw event\" is detected, get the Region of Interest, build an image mask from it, and compute the histogram of the original image for everything inside the mask."
        # "grab picture"
        # "shift state array \none place"
        n580 = local write "current state ( setup is idle)"(w987) -> ()
        n581 = local read "testrun with pinocam"() -> (w966:bool)
        n582 = local read "IR camera session ref"() -> (w983:T6)
        n583 = local read "Live image mem loc"() -> (w982:T8)
        n584 = call <vilib>:"IMAQdx Grab2.vi"("error in"=w980, "Image In"=w982, "Session In"=w983) -> ("error out"=w970:errorcluster, "Image Out"=w968:T8, "Session Out"=w981:T6)  [unwired: 5 in, 1 out]
        n585 = case shown="True" w966 {
          tunnel: w968 -> [w988 w990]
          tunnel: [w988 w989] -> w967
          frame False {
          }
          frame True {
            w991 = T23 7 items=["Grayscale (U8)", "Grayscale (I16)", "Grayscale (SGL)", "Complex (CSG)", "RGB (U32)", "HSL (U32)", "RGB (U64)", "Grayscale (U16)"] ("Image Type")
            n586 = call "IMAQ Cast Image"("Image Type"=w991, "Image Src"=w990) -> ("Image Dst Out"=w989:T8)  [unwired: 8 in, 1 out]
          }
        }
        n587 = local write "IR camera session ref"(w981) -> ()
        n588 = property on="StopROI" class="Bool"(error in=w970, "Blinking"=TRUE) -> (error out=w969:errorcluster)  [unwired: 1 in, 1 out]
        n589 = call "IMAQ Convert Rectangle to ROI"("Rectangle"=w976) -> ("error out"=w977:errorcluster, "ROI Descriptor"=w978:T11)  [unwired: 8 in]
        "ROI Descriptor" <- w978
        n590 = Delete From Array(array=w985, index=0) -> (deleted portion=w972:T1, array with subset deleted=w984:T1[])  [unwired: 1 in]
        n591 = local read "ROI Mask mem loc"() -> (w979:T8)
        n592 = local write "Live image setup tab"(w967) -> ()
        n593 = property on="Live image setup tab" class="ImageControl"(error in=w977, "ROI"=w978) -> ()  [unwired: 1 in, 2 out]
        n594 = local write "Live image camera tab"(w967) -> ()
        n595 = while {
          tunnel: w967 -> [w1002]
          tunnel: w979 -> [w1003]
          tunnel: [w1005] -> w974
          tunnel: [w1004] -> _
          tunnel: w975 -> [w995]
          i -> [w999]
          stop <- "StopROI" stop-if-true
          n596 = invoke on="Live image setup tab" class="ImageControl" method="Get Last Event"("Which Events"=w995) -> ("Type"=w996:i32)  [unwired: 7 in, 7 out]
          n597 = Not Equal To 0?(x=w996) -> (x != 0?=w1001:bool)
          n598 = Equal To 0?(x=w999) -> (x = 0?=w998:bool)
          n599 = Or(x=w998, y=w1001) -> (x .or. y?=w1000:bool)
          n600 = case shown="True" w1000 {
            tunnel: w1002 -> [w1007 w1015]
            tunnel: w1003 -> [w1006 w1012]
            tunnel: [w1006 w1010] -> w1005
            tunnel: [w1007 w1015] -> w1004
            frame False {
              n601 = Wait (ms)(milliseconds to wait=u32 100) -> ()  [unwired: 1 out]
            }
            frame True {
              n602 = property on="Live image setup tab" class="ImageControl"() -> ("ROI"=w1009:T26)  [unwired: 2 in, 2 out]
              n603 = call "IMAQ ROIToMask 2"("Image Model"=w1015, "ROI Descriptor"=w1009, "Image"=w1012) -> ("error out"=w1016:errorcluster, "Image Out"=w1010:T8)  [unwired: 6 in, 1 out]
              n604 = local write "ROI Descriptor"(w1009) -> ()
              n605 = call "IMAQ Histograph"("error in (no error)"=w1016, "Image Mask"=w1010, "Image"=w1015) -> ("Standard  Deviation"=→"histogram Standard Deviation":sgl, "Mean Value"=→"histogram Mean":sgl, "Histogram Graph"=w1011:T13)  [unwired: 5 in, 1 out]
              n606 = property on="Live image camera tab" class="ImageControl"("ROI"=w1009) -> ()  [unwired: 2 in, 2 out]
              n607 = local write "Waveform Graph"(w1011) -> ()
            }
          }
        }
        n608 = flat-sequence {
          tunnel: w974 -> [w994]
          tunnel: [w994] -> w973
          frame #0 {
            n609 = property on="control tab" class="TabCtl (strict)"("Tabs Visible?"=TRUE) -> ()  [unwired: 2 in, 2 out]
            n610 = property on="StopROI" class="Bool"("Blinking"=FALSE) -> ()  [unwired: 2 in, 2 out]
          }
        }
        n611 = local write "ROI Mask mem loc"(w973) -> ()
      }
      frame "focus calculation" {
        w1021 = 1000.0 ("y")
        w1043 = 1000.0 ("y")
        # "if save focus data is true but scan is test scan don't save data\nbecause of \"no path error\" WERKT NOG NIET IN TIMING MODE !!"
        # "round focus point to um resolution"
        # "recalculate new start and end point"
        # "determine if fit is in good enough\nto use"
        # "Inverse plot for inversed gausian data"
        # "determine highest point in contrast values"
        # "save focus data to txt file"
        # "shift state array \none place"
        n612 = local read "temp test scan"() -> (w1030:bool)
        n613 = local read "save focus data"() -> (w1028:bool)
        n614 = local read "real position array"() -> (w1025:dbl[])
        n615 = Not(x=w1030) -> (.not. x?=w1027:bool)
        n616 = And(x=w1028, y=w1027) -> (x .and. y?=w1029:bool)
        n617 = local read "contrast value array"() -> (w1026:sgl[])
        n618 = case shown="True" w1029 {
          tunnel: w1026 -> [_ w1067]
          tunnel: w1025 -> [_ w1068]
          frame False {
          }
          frame True {
            n619 = local read "path"() -> (w1071:path)
            n620 = Build Path(base path=w1071, name or relative path="focusdata.txt") -> (appended path=w1070:path)
            n621 = Build Array(w1068, w1067) -> (w1072:dbl[][])
            n622 = call-poly <vilib>:"Write Delimited Spreadsheet.vi"("file path (dialog if empty)"=w1070, "2D data"=w1072, "transpose? (no:F)"=TRUE) -> ()  [unwired: 11 in, 2 out]
          }
        }
        n623 = local write "current state ( setup is idle)"(w1059) -> ()
        n624 = Delete From Array(array=w1057, index=0) -> (deleted portion=w1056:T1, array with subset deleted=w1055:T1[])  [unwired: 1 in]
        n625 = Array Max & Min(array=w1026) -> (max value=w1053:sgl, max index (indices)=w1054:i32)  [unwired: 2 out]
        n626 = Index Array(array=w1025, index=w1054) -> (element=w1024:dbl)
        n627 = local write "waveform tab"(T12."measurement" ("waveform tab")) -> ()
        n628 = case shown="True" "inverse gausian" {
          tunnel: w1026 -> [w1074 w1078]
          tunnel: [w1074 w1076] -> w1047
          tunnel: w1053 -> [_ w1075]
          frame False {
          }
          frame True {
            n629 = Negate(x=w1078) -> (-x=w1077:sgl[])
            n630 = Add(x=w1077, y=w1075) -> (x+y=w1076:sgl[])
          }
        }
        n631 = Multiply(x=w1024, y=w1021) -> (x*y=w1023:dbl)
        n632 = Round To Nearest(number=w1023) -> (nearest integer value=w1022:dbl)
        n633 = Divide(x=w1022, y=w1021) -> (x/y=w1018:dbl)
        "max position" <- w1018
        n634 = call <vilib>:"Gaussian Peak Fit.vi"("Y"=w1047, "X"=w1025, "method"="Gausian fit method") -> ("Best Gaussian Fit"=w1048:dbl[], "center"=w1042:dbl, "standard deviation"=w1033:dbl)  [unwired: 6 in, 4 out]
        "standard deviation" <- w1033
        "standard deviation 2" <- w1033
        n635 = Bundle("real position array"=w1025, "contrast value array"=w1047) -> (w1051:T27)  [unwired: 1 in]
        n636 = Bundle("real position array"=w1025, "Best Gaussian Fit"=w1048) -> (w1050:T28)  [unwired: 1 in]
        n637 = Build Array(w1051, w1050) -> (→"XY Graph":T14)
        n638 = Greater?(x=w1033, y="Maximum standard deviation") -> (0:w1036:bool)
        n639 = Multiply(x=w1042, y=w1043) -> (x*y=w1045:dbl)
        n640 = Round To Nearest(number=w1045) -> (nearest integer value=w1044:dbl)
        n641 = Divide(x=w1044, y=w1043) -> (x/y=w1019:dbl)
        "Gausian fit center" <- w1019
        n642 = property on="XY Graph" class="XYGraph (strict)"("Active Cursor"=u32 0, "Cursor.Cursor X"=w1019, "Active Cursor"=u32 1, "Cursor.Cursor X"=w1024) -> ()  [unwired: 2 in, 2 out]
        n643 = case shown="True" "used for focuspoint" {
          tunnel: w1019 -> [w1060 _]
          tunnel: w1018 -> [_ w1061]
          tunnel: [w1060 w1061] -> w1017
          frame False {
            # "guasian fit"
          }
          frame True {
            # "max position"
          }
        }
        "focus drift" <- w1017
        n644 = local read "total scan depth"() -> (w1035:dbl)
        n645 = Divide(x=w1035, y=2.0) -> (x/y=w1039:dbl)
        n646 = Subtract(x=w1017, y=w1039) -> (x-y=w1032:dbl)
        n647 = Add(x=w1017, y=w1039) -> (x+y=w1031:dbl)
        n648 = case shown="False" w1036 {
          tunnel: w1031 -> [w1063 _]
          tunnel: w1032 -> [w1062 _]
          tunnel: w1017 -> [w1065 _]
          frame False {
            n649 = local write "focus point"(w1065) -> ()
            n650 = local write "start"(w1062) -> ()
            n651 = local write "end"(w1063) -> ()
            n652 = local write "temp test scan"(TRUE ("temp test scan")) -> ()
          }
          frame True {
            n653 = local write "temp test scan"(TRUE ("temp test scan")) -> ()
          }
        }
      }
      frame "move to start " {
        n654 = Delete From Array(array=w1084, index=0) -> (deleted portion=w1083:T1, array with subset deleted=w1082:T1[])  [unwired: 1 in]
        n655 = local read "testrun without motor"() -> (w1079:bool)
        n656 = local write "current state ( setup is idle)"(w1086) -> ()
        n657 = case shown="False" w1079 {
          tunnel: w1081 -> [w1088 w1096]
          tunnel: [w1087 w1096] -> w1080
          frame False {
            # "move stage back to start pos - extra offset against backlash"
            n658 = local read "Motor device ref"() -> (w1089:refnum<k24>)
            n659 = local read "backlash offset"() -> (w1091:dbl)
            n660 = local read "start"() -> (w1090:dbl)
            n661 = Subtract(x=w1090, y=w1091) -> (x-y=w1093:dbl)
            n662 = invoke class="KCubeDCServo" method="SetMoveAbsolutePosition"(reference=w1089, error in=w1088, "position"=w1093) -> (reference out=w1094:refnum<k24>, error out=w1095:errorcluster)  [unwired: 1 in, 2 out]
            n663 = invoke class="KCubeDCServo" method="MoveAbsolute"(reference=w1094, error in=w1095, "waitTimeout"=0) -> (error out=w1087:errorcluster)  [unwired: 1 in, 3 out]
          }
          frame True {
          }
        }
      }
      frame "timerset" {
        # "add extra 2% at begin and end of the graph"
        # "open array  timer data"
        # "shift state array \none place"
        n664 = local write "current state ( setup is idle)"(w1103) -> ()
        n665 = call-poly <vilib>:"Read Delimited Spreadsheet.vi"() -> ("all rows"=w1098:string[][])  [unwired: 10 in, 5 out]
        n666 = call "strip settings file.vi"("strip array in"=w1098) -> ("settings array out"=→"Timer settings array":string[][], "timer graph"=→"timer graph":cluster{cluster{timestamp, dbl}[]}[], "Xscalemax"=w1102:dbl, "cursor position"=w1101:dbl, "Xscle min"=w1100:dbl)  [unwired: 1 out]
        n667 = property on="timer graph" class="XYGraph (strict)"("XScale.Maximum"=w1102, "XScale.Minimum"=w1100, "Cursor.Cursor X"=w1101) -> ()  [unwired: 2 in, 2 out]
        n668 = Delete From Array(array=w1106, index=0) -> (deleted portion=w1105:T1, array with subset deleted=w1104:T1[])  [unwired: 1 in]
      }
      frame "timerscan" {
        # "check empty array"
        # "do scan based on file"
        # "check if scan is finished"
        n669 = local write "current state ( setup is idle)"(w1118) -> ()
        n670 = local read "Timer settings array"() -> (w1111:string[][])
        n671 = case shown="True" "first timerscan run ?" {
          tunnel: w1115 -> [_ w1119]
          frame False {
          }
          frame True {
            # "todo make state for this !"
            # "write temp state array at begin of scan\nto preserve state"
            n672 = local write "temp rep scan  state array"(w1119) -> ()
          }
        }
        n673 = Delete From Array(array=w1111, index (row)=0) -> (deleted portion=w1112:string[], array with subset deleted=w1109:string[][])  [unwired: 2 in]
        n674 = local write "Timer settings array"(w1109) -> ()
        n675 = Empty Array?(array=w1109) -> (empty?=w1108:bool)
        n676 = case shown="False" w1108 {
          tunnel: [w1121 w1338] -> w1117
          tunnel: [w1120 w1337] -> w1116
          tunnel: w1112 -> [w1123 _]
          frame False {
            # "settings file: \nYYYY-MM-DD\t    hh:mm:ss    \"command\"    [set]   OR\nDeltaT   hh:mm:ss    \"command\"    [set]\n\n\ncommands:\nmlight [on,off, 0-100%] microscope light on/off\nplight     [on,off, 0-100%]  plant light intesity change\nmpam    []  minipam pulse\nredpsiplight[on,off,0-100%] red channel PSI plant light intesity change\ngreenpsiplight[on,off,0-100%] green channel PSI plant light intesity change\nbluepsiplight[on,off,0-100%] blue channel PSI plant light intesity change\nfstack [] do a focus teststack without saving pictures\nrfstack []  do a nonliniar teststack without saving pics\nrstack []  do a single rough non lin stack\nrstack []  do a single stack\nrscan [ number of repetitions   time between meas(sec)] do a single non liniar scan and save the pics \nscan [number of repetitions   time between meas] do a scan and save pics\nexample :\n2020-09-21\t14:08:06\t plight\t80\n2020-09-21\t14:10:00\t mpam\n2020-09-21\t14:10:50  mlight on \n2020-09-21\t14:11:06\t rscan 10  120\n2020-09-21\t14:35:06  fstack\n\nOR\nDeltaT\t 14:08:06\t plight\t80\nDeltaT\t 14:10:00\t mpam\nDeltaT\t\t20:10:50  mlight on \nDeltaT\t 25:11:06\t rscan 10  120\nDeltaT\t\t114:35:06  fstack"
            # "do a scan and save pics with scan settings"
            n677 = disable-structure shown="Disabled" {
              frame Disabled {
                n678 = local write "waveform tab"(T12."long wait timer" ("waveform tab")) -> ()
              }
              frame Enabled {
              }
            }
            n679 = flat-sequence {
              tunnel: w1123 -> [w1128]
              tunnel: [w1130] -> w1124
              tunnel: w1124 -> [w1157]
              tunnel: [w1156] -> w1121
              tunnel: [w1155] -> w1120
              frame #0 {
                # "run till time and date match"
                n680 = node-c288() -> (w1132:T19)  [unwired: 4 in]
                n681 = Array To Cluster(array=w1128) -> (cluster=w1129:T29)
                n682 = Unbundle(w1129) -> ("Timer settings array[2]"=→"next function":string, "Timer settings array[3]"=→"next function argument":string)  [unwired: 2 out]
                n683 = timed-loop {
                  timing: w1132 -> [_]
                  timing-out: [_] -> w1131
                  tunnel: w1128 -> [w1141]
                  tunnel: [w1141] -> w1130
                  stop <- w1136 stop-if-true
                  n684 = node-c288() -> ()  [unwired: 1 in, 1 out]
                  n685 = Get Date/Time In Seconds() -> (seconds since 1Jan1904=w1133:timestamp)
                  "current date and time" <- w1133
                  "current time 2" <- w1133
                  n686 = Array To Cluster(array=w1141) -> (cluster=w1147:T30)
                  n687 = Unbundle(w1147) -> ("Timer settings array[0]"=w1143:string, "Timer settings array[1]"=w1145:string)
                  "time from file" <- w1145
                  "date from file" <- w1143
                  n688 = property on="control tab" class="TabCtl (strict)" props=["Value"]() -> ()  [unwired: 2 in, 3 out]
                  n689 = To Double Precision Float(number=w1133) -> (double precision float=w1134:dbl)
                  n690 = Format Date/Time String(time format string (%c)="%Y-%m-%d " ("format string"), seconds (now)=w1133) -> (date/time string=w1139:string)  [unwired: 1 in]
                  n691 = Get Date/Time String(seconds (now)=w1133, want seconds? (F)=TRUE) -> (time string=w1144:string)  [unwired: 1 in, 1 out]
                  n692 = Greater?(x=w1144, y=w1145) -> (0:w1146:bool)
                  n693 = property on="timer graph" class="XYGraph (strict)"("Cursor.Cursor X"=w1134) -> ()  [unwired: 2 in, 2 out]
                  n694 = call <vilib>:"Trim Whitespace.vi"("string"=w1139) -> ("trimmed string"=w1138:string)  [unwired: 1 in]
                  n695 = Equal?(x=w1143, y=w1138) -> (x = y?=w1142:bool)
                  n696 = And(x=w1146, y=w1142) -> (x .and. y?=w1137:bool)
                  n697 = local write "current time"(w1133) -> ()
                  n698 = Or(x=w1137, y=FALSE) -> (x .or. y?=w1136:bool)
                  n699 = node-c288() -> ()  [unwired: 1 in, 1 out]
                }
                n700 = node-c288(w1131) -> ()  [unwired: 1 out]
              }
              frame #1 {
                n701 = Array To Cluster(array=w1157) -> (cluster=w1158:T29)
                n702 = Unbundle(w1158) -> ("Timer settings array[2]"=w1159:string)  [unwired: 3 out]
                n703 = To Lower Case(string=w1159) -> (all lower case string=w1154:string)
                n704 = call <vilib>:"Trim Whitespace.vi"("string"=w1154) -> ("trimmed string"=w1153:string)  [unwired: 1 in]
                n705 = case shown="\"bluepsilight\"" w1153 {
                  tunnel: w1157 -> [_ w1179 _ _ _ _ w1225 w1238 _ w1270 w1290 w1310 w1330]
                  tunnel: [w1160 w1173 w1190 w1198 w1206 w1216 w1231 w1242 w1248 w1264 w1284 w1304 w1324] -> w1156
                  tunnel: [w1161 wobbe_statemachine."plight" ("Initial State") wobbe_statemachine."Minipam pulse" ("Initial State") wobbe_statemachine."start scan timer" ("Initial State") wobbe_statemachine."start scan timer" ("Initial State") wobbe_statemachine."ad curr date and time to save path" ("Initial State") wobbe_statemachine."do multi point scan " ("Initial State") wobbe_statemachine."do multi point scan " ("Initial State") wobbe_statemachine."ad curr date and time to save path" ("Initial State") wobbe_statemachine."mlight" ("Initial State") wobbe_statemachine."redpsilight" ("Initial State") wobbe_statemachine."greenpsilight" ("Initial State") wobbe_statemachine."bluepsilight" ("Initial State")] -> w1155
                  frame "False", Default {
                    n706 = local read "temp rep scan  state array"() -> (w1162:T1[])
                    n707 = Delete From Array(array=w1162, index=0) -> (deleted portion=w1161:T1, array with subset deleted=w1160:T1[])  [unwired: 1 in]
                  }
                  frame "plight" {
                    n708 = Index Array(array=w1179, index=3) -> (element=w1177:string)
                    n709 = Get Date/Time In Seconds() -> (seconds since 1Jan1904=w1171:timestamp)
                    n710 = call <vilib>:"Trim Whitespace.vi"("string"=w1177) -> ("trimmed string"=w1176:string)  [unwired: 1 in]
                    n711 = To Lower Case(string=w1176) -> (all lower case string=w1168:string)
                    n712 = case shown="Default" w1168 {
                      selector: w1168 -> [_ w1182 _]
                      frame "off" {
                        n713 = local write "plight [%]"(1) -> ()
                      }
                      frame Default {
                        n714 = Decimal String To Number(string=w1182) -> (number=w1181:i32)  [unwired: 2 in, 1 out]
                        n715 = local write "plight [%]"(w1181) -> ()
                      }
                      frame "on" {
                        n716 = local write "plight [%]"(100) -> ()
                      }
                    }
                    n717 = Format Date/Time String(time format string (%c)="%Y%m%d_%H%M%S%1u_Plight_", seconds (now)=w1171) -> (date/time string=w1169:string)  [unwired: 1 in]
                    n718 = local read "selected path"() -> (w1170:path)
                    n719 = Build Array(wobbe_statemachine."timerscan" ("Initial State")) -> (w1173:T1[])
                    n720 = Concatenate Strings(w1169, w1168, ".dat" ("string")) -> (w1166:string)
                    n721 = Build Path(base path=w1170, name or relative path=w1166) -> (appended path=w1165:path)
                    n722 = Open/Create/Replace File(file path (use dialog)=w1165, operation (0:open)=T22."create") -> ()  [unwired: 4 in, 3 out]
                  }
                  frame "mpam" {
                    n723 = Get Date/Time In Seconds() -> (seconds since 1Jan1904=w1188:timestamp)
                    n724 = local read "selected path"() -> (w1184:path)
                    n725 = Format Date/Time String(time format string (%c)="%Y%m%d_%H%M%S%1u_mpam.dat", seconds (now)=w1188) -> (date/time string=w1185:string)  [unwired: 1 in]
                    n726 = Build Array(wobbe_statemachine."timerscan" ("Initial State")) -> (w1190:T1[])
                    n727 = Build Path(base path=w1184, name or relative path=w1185) -> (appended path=w1187:path)
                    n728 = Open/Create/Replace File(file path (use dialog)=w1187, operation (0:open)=T22."create") -> ()  [unwired: 4 in, 3 out]
                  }
                  frame "fstack" {
                    # "do scan without saving pics"
                    n729 = local write "use nonlin steps"(FALSE ("use nonlin steps")) -> ()
                    n730 = local write "save focus data"(TRUE ("save focus data")) -> ()
                    n731 = Build Array(wobbe_statemachine."ad curr date and time to save path" ("Initial State"), wobbe_statemachine."do test scan" ("Initial State"), wobbe_statemachine."move to start " ("Initial State"), wobbe_statemachine."focus calculation" ("Initial State"), wobbe_statemachine."stop scan timer" ("Initial State"), wobbe_statemachine."timerscan" ("Initial State")) -> (w1198:T1[])
                  }
                  frame "rfstack" {
                    # "do an rough non liniar stack  without saving pics"
                    n732 = local write "save focus data"(TRUE ("save focus data")) -> ()
                    n733 = local write "use nonlin steps"(TRUE ("use nonlin steps")) -> ()
                    n734 = Build Array(wobbe_statemachine."ad curr date and time to save path" ("Initial State"), wobbe_statemachine."do non lin test scan" ("Initial State"), wobbe_statemachine."move to start " ("Initial State"), wobbe_statemachine."focus calculation" ("Initial State"), wobbe_statemachine."stop scan timer" ("Initial State"), wobbe_statemachine."timerscan" ("Initial State")) -> (w1206:T1[])
                  }
                  frame "rstack" {
                    # "do an rough  non liniair stack"
                    n735 = local write "use nonlin steps"(TRUE ("use nonlin steps")) -> ()
                    n736 = local write "save focus data"(TRUE ("save focus data")) -> ()
                    n737 = Build Array(wobbe_statemachine."start scan timer" ("Initial State"), wobbe_statemachine."do non lin scan" ("Initial State"), wobbe_statemachine."move to start " ("Initial State"), wobbe_statemachine."focus calculation" ("Initial State"), wobbe_statemachine."stop scan timer" ("Initial State"), wobbe_statemachine."timerscan" ("Initial State")) -> (w1216:T1[])
                  }
                  frame "rscan" {
                    # "do an rough  non liniair stack"
                    n738 = Array To Cluster(array=w1225) -> (cluster=w1228:T31)
                    n739 = Unbundle(w1228) -> ("Timer settings array[3]"=w1227:string, "Timer settings array[4]"=w1226:string)  [unwired: 3 out]
                    n740 = local write "use nonlin steps"(TRUE ("use nonlin steps")) -> ()
                    n741 = local write "save focus data"(TRUE ("save focus data")) -> ()
                    n742 = Decimal String To Number(string=w1226) -> (number=w1223:i32)  [unwired: 2 in, 1 out]
                    "rep time" <- w1223
                    n743 = Decimal String To Number(string=w1227) -> (number=w1224:i32)  [unwired: 2 in, 1 out]
                    "nrfrep" <- w1224
                    n744 = local write "repetition time [s]"(w1223) -> ()
                    n745 = local write "nr of repetitions"(w1224) -> ()
                    n746 = Build Array(wobbe_statemachine."timerscan" ("Initial State")) -> (w1231:T1[])
                  }
                  frame "scan" {
                    # "time between meas (sec)"
                    # "number of repetitions"
                    # "do a single stack"
                    n747 = Array To Cluster(array=w1238) -> (cluster=w1239:T31)
                    n748 = Unbundle(w1239) -> ("Timer settings array[3]"=w1237:string, "Timer settings array[4]"=w1235:string)  [unwired: 3 out]
                    n749 = local write "use nonlin steps"(FALSE ("use nonlin steps")) -> ()
                    n750 = local write "save focus data"(TRUE ("save focus data")) -> ()
                    n751 = Decimal String To Number(string=w1235) -> (number=w1234:i32)  [unwired: 2 in, 1 out]
                    n752 = Decimal String To Number(string=w1237) -> (number=w1236:i32)  [unwired: 2 in, 1 out]
                    n753 = local write "repetition time [s]"(w1234) -> ()
                    n754 = local write "nr of repetitions"(w1236) -> ()
                    n755 = Build Array(wobbe_statemachine."timerscan" ("Initial State")) -> (w1242:T1[])
                  }
                  frame "stack" {
                    # "do a scan and save pics with scan settings"
                    n756 = local write "save focus data"(TRUE ("save focus data")) -> ()
                    n757 = local write "use nonlin steps"(FALSE ("use nonlin steps")) -> ()
                    n758 = Build Array(wobbe_statemachine."start scan timer" ("Initial State"), wobbe_statemachine."do scan" ("Initial State"), wobbe_statemachine."move to start " ("Initial State"), wobbe_statemachine."focus calculation" ("Initial State"), wobbe_statemachine."stop scan timer" ("Initial State"), wobbe_statemachine."timerscan" ("Initial State")) -> (w1248:T1[])
                  }
                  frame "mlight" {
                    n759 = Index Array(array=w1270, index=3) -> (element=w1268:string)
                    n760 = call <vilib>:"Trim Whitespace.vi"("string"=w1268) -> ("trimmed string"=w1267:string)  [unwired: 1 in]
                    n761 = To Lower Case(string=w1267) -> (all lower case string=w1256:string)
                    n762 = Get Date/Time In Seconds() -> (seconds since 1Jan1904=w1262:timestamp)
                    n763 = local read "selected path"() -> (w1255:path)
                    n764 = case shown="\"off\"" w1256 {
                      selector: w1256 -> [_ w1273 _]
                      frame "off" {
                        n765 = local write "mlight [%]"(1) -> ()
                      }
                      frame Default {
                        n766 = Decimal String To Number(string=w1273) -> (number=w1272:i32)  [unwired: 2 in, 1 out]
                        n767 = local write "mlight [%]"(w1272) -> ()
                      }
                      frame "on" {
                        n768 = local write "mlight [%]"(100) -> ()
                      }
                    }
                    n769 = Format Date/Time String(time format string (%c)="%Y%m%d_%H%M%S%1u_Mlight_", seconds (now)=w1262) -> (date/time string=w1261:string)  [unwired: 1 in]
                    n770 = Build Array(wobbe_statemachine."timerscan" ("Initial State")) -> (w1264:T1[])
                    n771 = Concatenate Strings(w1261, w1256, ".dat" ("string")) -> (w1259:string)
                    n772 = Build Path(base path=w1255, name or relative path=w1259) -> (appended path=w1258:path)
                    n773 = Open/Create/Replace File(file path (use dialog)=w1258, operation (0:open)=T22."create") -> ()  [unwired: 4 in, 3 out]
                  }
                  frame "redpsilight" {
                    n774 = Index Array(array=w1290, index=3) -> (element=w1288:string)
                    n775 = call <vilib>:"Trim Whitespace.vi"("string"=w1288) -> ("trimmed string"=w1287:string)  [unwired: 1 in]
                    n776 = To Lower Case(string=w1287) -> (all lower case string=w1276:string)
                    n777 = Get Date/Time In Seconds() -> (seconds since 1Jan1904=w1282:timestamp)
                    n778 = local read "selected path"() -> (w1275:path)
                    n779 = case shown="\"on\"" w1276 {
                      selector: w1276 -> [_ w1293 _]
                      frame "off" {
                        n780 = local write "red"(FALSE ("red")) -> ()
                      }
                      frame Default {
                        n781 = Decimal String To Number(string=w1293) -> (number=w1292:i32)  [unwired: 2 in, 1 out]
                        n782 = local write "red"(w1292) -> ()
                      }
                      frame "on" {
                        n783 = local write "red"(TRUE ("red")) -> ()
                      }
                    }
                    n784 = Format Date/Time String(time format string (%c)="%Y%m%d_%H%M%S%1u_Mlight_", seconds (now)=w1282) -> (date/time string=w1281:string)  [unwired: 1 in]
                    n785 = Build Array(wobbe_statemachine."timerscan" ("Initial State")) -> (w1284:T1[])
                    n786 = Concatenate Strings(w1281, w1276, ".dat" ("string")) -> (w1279:string)
                    n787 = Build Path(base path=w1275, name or relative path=w1279) -> (appended path=w1278:path)
                    n788 = Open/Create/Replace File(file path (use dialog)=w1278, operation (0:open)=T22."create") -> ()  [unwired: 4 in, 3 out]
                  }
                  frame "greenpsilight" {
                    n789 = Index Array(array=w1310, index=3) -> (element=w1308:string)
                    n790 = call <vilib>:"Trim Whitespace.vi"("string"=w1308) -> ("trimmed string"=w1307:string)  [unwired: 1 in]
                    n791 = To Lower Case(string=w1307) -> (all lower case string=w1296:string)
                    n792 = Get Date/Time In Seconds() -> (seconds since 1Jan1904=w1302:timestamp)
                    n793 = local read "selected path"() -> (w1295:path)
                    n794 = case shown="\"on\"" w1296 {
                      selector: w1296 -> [_ w1313 _]
                      frame "off" {
                        n795 = local write "green"(FALSE ("green")) -> ()
                      }
                      frame Default {
                        n796 = Decimal String To Number(string=w1313) -> (number=w1312:i32)  [unwired: 2 in, 1 out]
                        n797 = local write "green"(w1312) -> ()
                      }
                      frame "on" {
                        n798 = local write "green"(TRUE ("green")) -> ()
                      }
                    }
                    n799 = Format Date/Time String(time format string (%c)="%Y%m%d_%H%M%S%1u_Mlight_", seconds (now)=w1302) -> (date/time string=w1301:string)  [unwired: 1 in]
                    n800 = Build Array(wobbe_statemachine."timerscan" ("Initial State")) -> (w1304:T1[])
                    n801 = Concatenate Strings(w1301, w1296, ".dat" ("string")) -> (w1299:string)
                    n802 = Build Path(base path=w1295, name or relative path=w1299) -> (appended path=w1298:path)
                    n803 = Open/Create/Replace File(file path (use dialog)=w1298, operation (0:open)=T22."create") -> ()  [unwired: 4 in, 3 out]
                  }
                  frame "bluepsilight" {
                    n804 = Index Array(array=w1330, index=3) -> (element=w1328:string)
                    n805 = call <vilib>:"Trim Whitespace.vi"("string"=w1328) -> ("trimmed string"=w1327:string)  [unwired: 1 in]
                    n806 = To Lower Case(string=w1327) -> (all lower case string=w1316:string)
                    n807 = Get Date/Time In Seconds() -> (seconds since 1Jan1904=w1322:timestamp)
                    n808 = local read "selected path"() -> (w1315:path)
                    n809 = case shown="\"on\"" w1316 {
                      selector: w1316 -> [_ w1333 _]
                      frame "off" {
                        n810 = local write "blue"(FALSE ("blue")) -> ()
                      }
                      frame Default {
                        n811 = Decimal String To Number(string=w1333) -> (number=w1332:i32)  [unwired: 2 in, 1 out]
                        n812 = local write "blue"(w1332) -> ()
                      }
                      frame "on" {
                        n813 = local write "blue"(TRUE ("blue")) -> ()
                      }
                    }
                    n814 = Format Date/Time String(time format string (%c)="%Y%m%d_%H%M%S%1u_Mlight_", seconds (now)=w1322) -> (date/time string=w1321:string)  [unwired: 1 in]
                    n815 = Build Array(wobbe_statemachine."timerscan" ("Initial State")) -> (w1324:T1[])
                    n816 = Concatenate Strings(w1321, w1316, ".dat" ("string")) -> (w1319:string)
                    n817 = Build Path(base path=w1315, name or relative path=w1319) -> (appended path=w1318:path)
                    n818 = Open/Create/Replace File(file path (use dialog)=w1318, operation (0:open)=T22."create") -> ()  [unwired: 4 in, 3 out]
                  }
                }
              }
            }
            n819 = local write "first timerscan run ?"(FALSE ("first timerscan run ?")) -> ()
          }
          frame True {
            # "shift state array \none place"
            # "reset counter, and  resume state array"
            n820 = local write "first timerscan run ?"(TRUE ("first timerscan run ?")) -> ()
            n821 = local write "Run with \nexternal \ntiming settings"(FALSE ("Run with \nexternal \ntiming settings")) -> ()
            n822 = local read "temp rep scan  state array"() -> (w1339:T1[])
            n823 = Delete From Array(array=w1339, index=0) -> (deleted portion=w1337:T1, array with subset deleted=w1338:T1[])  [unwired: 1 in]
          }
        }
      }
      frame "Stop" {
        w1353 = T1[] [enum."Stop"] items=["Initialize", "set up measurement", "camera settings", "set roi", "ad curr date and time to save path", "plight", "mlight", "move to start ", "grab picture without save", "Minipam pulse", "do scan", "do non lin scan", "do test scan", "do non lin test scan", "select save path", "move to position", "grab picture", "focus calculation", "Stop", "timerset", "stop scan timer", "start scan timer", "write scan time", "do multi point scan ", "simple timer", "timerscan", "read temp scan array", "write temp scan state array", "bluepsilight", "greenpsilight", "redpsilight"] ("temp rep scan  state array")
        n824 = local write "current state ( setup is idle)"(w1356) -> ()
        n825 = property on="control tab" class="TabCtl (strict)"() -> ("Pages"=w1342:refnum<vi>[])  [unwired: 2 in, 2 out]
        n826 = local read "IR camera session ref"() -> (w1352:T6)
        n827 = local read "filtered image mem loc"() -> (w1350:T8)
        n828 = local read "Live image mem loc"() -> (w1349:T8)
        n829 = local read "ROI Mask mem loc"() -> (w1351:T8)
        n830 = Index Array(array=w1342, index=2) -> (element=w1346:refnum<vi>)
        n831 = property on="camera settings" class="Bool"("DisabledEnum"=T15."Enabled" ("Disabled")) -> ()  [unwired: 2 in, 2 out]
        n832 = Index Array(array=w1342, index=5) -> (element=w1341:refnum<vi>)
        n833 = property class="Page"(reference=w1346, "PageVis"=TRUE ("Page Visible")) -> ()  [unwired: 1 in, 2 out]
        n834 = property class="Page"(reference=w1341, "PageVis"=TRUE ("Page Visible")) -> ()  [unwired: 1 in, 2 out]
        n835 = call "IMAQ Dispose"("Image"=w1349) -> ()  [unwired: 5 in, 1 out]
        n836 = call <vilib>:"IMAQdx Close Camera.vi"("Session In"=w1352) -> ()  [unwired: 10 in, 1 out]
        n837 = call "IMAQ Dispose"("Image"=w1351) -> ()  [unwired: 5 in, 1 out]
        n838 = call "IMAQ Dispose"("Image"=w1350) -> ()  [unwired: 5 in, 1 out]
        n839 = local write "stopprogram"(TRUE ("stop")) -> ()
      }
    }
    n840 = local read "stopprogram"() -> (w6:bool)
  }
  n841 = flat-sequence {
    frame #0 {
      # "wait for init in control loop to run"
      n842 = while {
        stop <- "wait control loop untill init" stop-if-true
        n843 = Wait (ms)(milliseconds to wait=u32 100) -> ()  [unwired: 1 out]
      }
    }
    frame #1 {
      # "seperate control loop to keep the front pannel from locking during run state machine"
      n844 = local read "Live image mem loc"() -> (w1359:T8)
      n845 = while {
        shift-right: [w1368] -> w1361
        shift-left: "error in" -> [w1369]
        tunnel: w1359 -> [w1367]
        stop <- w1365 stop-if-true
        # "save state \nfor timeout\nevent by \nstoping loop"
        n846 = event shown="[16] \"green\", \"green\": Value Change" {
          selector: _ -> [_ _ _ _ _ _ _ _ _ _ _ _ _ _ _ _ _ _ _ _ _ _ _ _]
          dyn-events: _ -> [_ _ _ _ _ _ _ _ _ _ _ _ _ _ _ _ _ _ _ _ _ _ _ _]
          timeout: -1 -> [_ _ _ _ _ _ _ _ _ _ _ _ _ _ _ _ _ _ _ _ _ _ _ _]
          tunnel: w1369 -> [_ _ w1396 w1405 _ _ _ _ _ _ _ _ _ _ _ _ _ _ _ _ _ _ _ _]
          tunnel: [_ _ w1396 w1405 _ _ _ _ _ _ _ _ _ _ _ _ _ _ _ _ _ _ _ _] -> w1368
          tunnel: w1367 -> [_ _ _ _ _ _ _ _ _ _ _ _ _ _ _ _ _ _ _ _ _ _ _ _]
          tunnel: [w1374 w1379 w1395 w1403 w1417 _ _ _ _ _ _ _ _ _ _ _ _ _ _ _ w1770 w1793 w1797 w1815] -> w1364
          tunnel: [w1373 w1377 w1392 wobbe_statemachine."Stop" ("Initial State") w1406 _ _ _ _ _ _ _ _ _ _ _ _ _ _ _ w1766 wobbe_statemachine."select save path" ("Initial State") w1796 wobbe_statemachine."select save path" ("Initial State")] -> w1363
          tunnel: [TRUE ("stop setup loop") w1378 TRUE ("stop setup loop") TRUE ("stop setup loop") TRUE ("stop setup loop") FALSE ("stop setup loop") FALSE ("stop setup loop") FALSE ("stop setup loop") FALSE ("stop setup loop") FALSE ("stop setup loop") FALSE ("stop setup loop") FALSE ("stop setup loop") FALSE ("stop setup loop") FALSE ("stop setup loop") FALSE ("stop setup loop") FALSE ("stop setup loop") FALSE ("stop setup loop") FALSE ("stop setup loop") FALSE ("stop setup loop") FALSE ("stop setup loop") TRUE ("stop setup loop") TRUE ("stop setup loop") w1795 TRUE ("stop setup loop")] -> w1362
          tunnel: [w1373 w1377 w1392 _ w1406 _ _ _ _ _ _ _ _ _ _ _ _ _ _ _ w1766 _ _ _] -> _
          tunnel: [_ _ _ "stopprogram" _ _ _ _ _ _ _ _ _ _ _ _ _ _ _ _ _ _ _ _] -> w1365
          event Timeout {
            w1374 = T1[] [enum."set up measurement", enum."set up measurement"] items=["Initialize", "set up measurement", "camera settings", "set roi", "ad curr date and time to save path", "plight", "mlight", "move to start ", "grab picture without save", "Minipam pulse", "do scan", "do non lin scan", "do test scan", "do non lin test scan", "select save path", "move to position", "grab picture", "focus calculation", "Stop", "timerset", "stop scan timer", "start scan timer", "write scan time", "do multi point scan ", "simple timer", "timerscan", "read temp scan array", "write temp scan state array", "bluepsilight", "greenpsilight", "redpsilight"]
            w1373 = wobbe_statemachine."set up measurement" ("Initial State")
            # "show camera image"
            n847 = event-data() -> ()  [unwired: 1 in, 3 out]
          }
          event "load external\n timing settings": Value Change {
            n848 = event-data() -> ("NewVal"=w1376:bool)  [unwired: 1 in, 5 out]
            n849 = case shown="True" w1376 {
              tunnel: [w1384 w1390] -> w1379
              tunnel: [TRUE ("stop setup loop") FALSE ("stop setup loop")] -> w1378
              tunnel: [w1381 w1387] -> w1377
              frame True {
                w1381 = wobbe_statemachine."timerset"  # Initial State
                n850 = local write "load external\n timing settings"(FALSE ("Run with \nexternal \ntiming settings")) -> ()
                n851 = local write "waveform tab"(T12."long wait timer" ("waveform tab")) -> ()
                n852 = Build Array(wobbe_statemachine."set up measurement" ("Initial State")) -> (w1384:T1[])
              }
              frame False {
                w1387 = wobbe_statemachine."set up measurement"  # Initial State
                n853 = local write "load external\n timing settings"(FALSE ("Run with \nexternal \ntiming settings")) -> ()
                n854 = local write "waveform tab"(T12."long wait timer" ("waveform tab")) -> ()
                n855 = Build Array(wobbe_statemachine."set up measurement" ("Initial State")) -> (w1390:T1[])
              }
            }
          }
          event "Set ROI": Value Change {
            w1392 = wobbe_statemachine."set roi" ("Initial State")
            # "Set ROI"
            n856 = event-data() -> ()  [unwired: 1 in, 6 out]
            n857 = flat-sequence {
              frame #0 {
                n858 = local write "waveform tab"(T12."setup measurement" ("waveform tab")) -> ()
                n859 = local write "control tab"(T2."main" ("control tab")) -> ()
              }
              frame #1 {
                n860 = property on="control tab" class="TabCtl (strict)"("Tabs Visible?"=FALSE) -> ()  [unwired: 2 in, 2 out]
              }
            }
            n861 = Build Array(wobbe_statemachine."set up measurement" ("Initial State")) -> (w1395:T1[])
          }
          event "stopprogram": Value Change {
            n862 = event-data() -> ()  [unwired: 1 in, 6 out]
            n863 = Build Array(wobbe_statemachine."Stop" ("Initial State")) -> (w1403:T1[])
          }
          event "camera settings", "control tab": Value Change {
            w1414 = T33 0 items=["no dialog", "OK message", "continue or stop message", "OK message + warnings", "continue/stop + warnings"] ("type of dialog (OK msg:1)")
            # "gives error if camera settings buton is pushed"
            # "check if camera settings tab is pushed"
            n864 = event-data() -> ("NewVal"=w1416:variant)  [unwired: 1 in, 5 out]
            n865 = local read "control tab"() -> (w1415:T2)
            n866 = Variant To Data(type=w1415, Variant=w1416) -> (data=w1412:T2, error out=w1413:errorcluster)  [unwired: 1 in]
            n867 = call <vilib>:"Simple Error Handler.vi"("type of dialog (OK msg:1)"=w1414, "error in (no error)"=w1413) -> ("error?"=w1409:bool)  [unwired: 3 in, 4 out]
            n868 = Equal?(x=w1412, y=T32."camera set") -> (x = y?=w1410:bool)
            n869 = Or(x=w1410, y=w1409) -> (x .or. y?=w1408:bool)
            n870 = case shown="False" w1408 {
              tunnel: [w1418 w1422] -> w1417
              tunnel: [wobbe_statemachine."set up measurement" ("Initial State") wobbe_statemachine."camera settings" ("Initial State")] -> w1406
              frame False {
                # "other tab pushed go back to main menu"
                n871 = Build Array(wobbe_statemachine."set up measurement" ("Initial State")) -> (w1418:T1[])
              }
              frame True {
                # "change camera settings"
                n872 = flat-sequence {
                  frame #0 {
                    n873 = local write "waveform tab"(T12."setup measurement" ("waveform tab")) -> ()
                    n874 = local write "control tab"(T2."cam set" ("control tab")) -> ()
                  }
                  frame #1 {
                    # "block other tabs"
                    n875 = property on="control tab" class="TabCtl (strict)"("Tabs Visible?"=FALSE) -> ()  [unwired: 2 in, 2 out]
                  }
                }
                n876 = Build Array(wobbe_statemachine."set up measurement" ("Initial State")) -> (w1422:T1[])
              }
            }
          }
          event "stepsize (mm)": Value Change {
            # "calculate step settings based on change in fine stepsize"
            n877 = event-data() -> ("NewVal"=w1429:dbl)  [unwired: 1 in, 5 out]
            n878 = local read "use nonlin steps"() -> (w1428:bool)
            n879 = case shown="True" w1428 {
              tunnel: w1429 -> [w1442 w1452]
              frame True {
                # "change of stepsize:  calculate start and end based on scan depth rough and fine\nrecalculate number of fine steps based on scan depth"
                n880 = local read "rough extra number \nof steps both sides"() -> (w1439:dbl)
                n881 = local read "rough extra scan depth \nboth sides(mm)"() -> (w1434:dbl)
                n882 = local read "scan depth (mm)"() -> (w1431:dbl)
                n883 = Divide(x=w1431, y=w1442) -> (x/y=w1449:dbl)
                n884 = Round To Nearest(number=w1449) -> (nearest integer value=w1435:dbl)
                n885 = Multiply(x=2.0, y=w1434) -> (x*y=w1432:dbl)
                n886 = Add(x=w1431, y=w1432) -> (x+y=w1430:dbl)
                n887 = Multiply(x=w1435, y=w1442) -> (x*y=w1448:dbl)
                n888 = local read "focus point"() -> (w1446:dbl)
                n889 = local write "number of steps"(w1435) -> ()
                n890 = Divide(x=w1448, y=2.0) -> (x/y=w1445:dbl)
                n891 = Multiply(x=w1439, y=2.0) -> (x*y=w1437:dbl)
                n892 = local write "total scan depth"(w1430) -> ()
                n893 = Add(x=w1435, y=w1437) -> (x+y=w1436:dbl)
                n894 = Add(x=w1446, y=w1445) -> (x+y=w1443:dbl)
                n895 = Subtract(x=w1446, y=w1445) -> (x-y=w1444:dbl)
                n896 = local write "total nr of steps"(w1436) -> ()
                n897 = Add(x=w1434, y=w1443) -> (x+y=w1440:dbl)
                n898 = Subtract(x=w1444, y=w1434) -> (x-y=w1441:dbl)
                n899 = local write "start"(w1441) -> ()
                n900 = local write "end"(w1440) -> ()
              }
              frame False {
                # "change of stepsize:  calculate start and end based on scan depth\nrecalculate number of steps based on scan depth"
                n901 = local read "scan depth (mm)"() -> (w1451:dbl)
                n902 = Divide(x=w1451, y=w1452) -> (x/y=w1459:dbl)
                n903 = Round To Nearest(number=w1459) -> (nearest integer value=w1450:dbl)
                n904 = Multiply(x=w1450, y=w1452) -> (x*y=w1458:dbl)
                n905 = local write "number of steps"(w1450) -> ()
                n906 = local read "focus point"() -> (w1456:dbl)
                n907 = local write "total scan depth"(w1451) -> ()
                n908 = Divide(x=w1458, y=2.0) -> (x/y=w1455:dbl)
                n909 = Add(x=w1456, y=w1455) -> (x+y=w1453:dbl)
                n910 = Subtract(x=w1456, y=w1455) -> (x-y=w1454:dbl)
                n911 = local write "start"(w1454) -> ()
                n912 = local write "end"(w1453) -> ()
                n913 = local write "total nr of steps"(w1450) -> ()
              }
            }
          }
          event "rough stepsize (mm)": Value Change {
            # "change of stepsize:  calculate start and end based on scan depth rough and fine\nrecalculate number of fine steps based on scan depth"
            n914 = event-data() -> ("NewVal"=w1464:dbl)  [unwired: 1 in, 5 out]
            n915 = local read "scan depth (mm)"() -> (w1467:dbl)
            n916 = local read "rough extra scan depth \nboth sides(mm)"() -> (w1463:dbl)
            n917 = local read "stepsize (mm)"() -> (w1465:dbl)
            n918 = Divide(x=w1467, y=w1465) -> (x/y=w1482:dbl)
            n919 = Round To Nearest(number=w1482) -> (nearest integer value=w1470:dbl)
            n920 = Multiply(x=w1470, y=w1465) -> (x*y=w1481:dbl)
            n921 = local read "focus point"() -> (w1479:dbl)
            n922 = Divide(x=w1463, y=w1464) -> (x/y=w1462:dbl)
            n923 = Multiply(x=2.0, y=w1463) -> (x*y=w1468:dbl)
            n924 = Divide(x=w1481, y=2.0) -> (x/y=w1478:dbl)
            n925 = Add(x=w1467, y=w1468) -> (x+y=w1466:dbl)
            n926 = Add(x=w1479, y=w1478) -> (x+y=w1476:dbl)
            n927 = Subtract(x=w1479, y=w1478) -> (x-y=w1477:dbl)
            n928 = Round To Nearest(number=w1462) -> (nearest integer value=w1461:dbl)
            n929 = Add(x=w1463, y=w1476) -> (x+y=w1474:dbl)
            n930 = Subtract(x=w1477, y=w1463) -> (x-y=w1475:dbl)
            n931 = Multiply(x=w1461, y=2.0) -> (x*y=w1472:dbl)
            n932 = local write "rough extra number \nof steps both sides"(w1461) -> ()
            n933 = local write "total scan depth"(w1466) -> ()
            n934 = local write "start"(w1475) -> ()
            n935 = local write "end"(w1474) -> ()
            n936 = Add(x=w1470, y=w1472) -> (x+y=w1471:dbl)
            n937 = local write "total nr of steps"(w1471) -> ()
          }
          event "number of steps": Value Change {
            n938 = event-data() -> ("NewVal"=w1485:dbl)  [unwired: 1 in, 5 out]
            n939 = local read "use nonlin steps"() -> (w1484:bool)
            n940 = case shown="False" w1484 {
              tunnel: w1485 -> [w1494 w1515]
              frame True {
                w1497 = 1000.0 ("y")
                # "recalculate stepsize in micrometer steps based on scan depth and number of steps"
                n941 = local read "rough extra number \nof steps both sides"() -> (w1507:dbl)
                n942 = local read "scan depth (mm)"() -> (w1508:dbl)
                n943 = local read "focus point"() -> (w1492:dbl)
                n944 = local read "rough extra number \nof steps both sides"() -> (w1490:dbl)
                n945 = local read "rough stepsize (mm)"() -> (w1491:dbl)
                n946 = Divide(x=w1508, y=w1494) -> (x/y=w1513:dbl)
                n947 = Multiply(x=w1513, y=1000.0) -> (x*y=w1511:dbl)
                n948 = Multiply(x=2.0, y=w1507) -> (x*y=w1505:dbl)
                n949 = Round To Nearest(number=w1511) -> (nearest integer value=w1510:dbl)
                n950 = Add(x=w1494, y=w1505) -> (x+y=w1504:dbl)
                n951 = Multiply(x=w1490, y=w1491) -> (x*y=w1489:dbl)
                n952 = Multiply(x=w1489, y=2.0) -> (x*y=w1501:dbl)
                n953 = Divide(x=w1510, y=1000.0) -> (x/y=w1493:dbl)
                n954 = Multiply(x=w1494, y=w1493) -> (x*y=w1502:dbl)
                n955 = local write "stepsize (mm)"(w1493) -> ()
                n956 = local write "total nr of steps"(w1504) -> ()
                n957 = Add(x=w1502, y=w1501) -> (x+y=w1488:dbl)
                n958 = Divide(x=w1488, y=2.0) -> (x/y=w1487:dbl)
                n959 = Multiply(x=w1487, y=w1497) -> (x*y=w1500:dbl)
                n960 = Round To Nearest(number=w1500) -> (nearest integer value=w1499:dbl)
                n961 = Divide(x=w1499, y=w1497) -> (x/y=w1498:dbl)
                n962 = Subtract(x=w1492, y=w1498) -> (x-y=w1496:dbl)
                n963 = Add(x=w1498, y=w1492) -> (x+y=w1495:dbl)
                n964 = local write "total scan depth"(w1488) -> ()
                n965 = local write "start"(w1496) -> ()
                n966 = local write "end"(w1495) -> ()
              }
              frame False {
                w1520 = 1000.0 ("y")
                # "recalculate stepsize in micrometer steps based on scan depth and number of steps"
                n967 = local read "scan depth (mm)"() -> (w1526:dbl)
                n968 = local read "focus point"() -> (w1516:dbl)
                n969 = Divide(x=w1526, y=w1515) -> (x/y=w1531:dbl)
                n970 = Multiply(x=w1531, y=1000.0) -> (x*y=w1529:dbl)
                n971 = Round To Nearest(number=w1529) -> (nearest integer value=w1528:dbl)
                n972 = Divide(x=w1528, y=1000.0) -> (x/y=w1517:dbl)
                n973 = Multiply(x=w1515, y=w1517) -> (x*y=w1514:dbl)
                n974 = local write "stepsize (mm)"(w1517) -> ()
                n975 = local write "total nr of steps"(w1515) -> ()
                n976 = Divide(x=w1514, y=2.0) -> (x/y=w1524:dbl)
                n977 = Multiply(x=w1524, y=w1520) -> (x*y=w1523:dbl)
                n978 = Round To Nearest(number=w1523) -> (nearest integer value=w1522:dbl)
                n979 = Divide(x=w1522, y=w1520) -> (x/y=w1521:dbl)
                n980 = Subtract(x=w1516, y=w1521) -> (x-y=w1519:dbl)
                n981 = Add(x=w1521, y=w1516) -> (x+y=w1518:dbl)
                n982 = local write "total scan depth"(w1514) -> ()
                n983 = local write "start"(w1519) -> ()
                n984 = local write "end"(w1518) -> ()
              }
            }
          }
          event "rough extra number \nof steps both sides": Value Change {
            w1534 = 1000.0 ("y")
            w1549 = 1000.0 ("y")
            # "recalculate rough stepsize in micrometer steps based on  rough extrascan depth and extra number of steps"
            n985 = event-data() -> ("NewVal"=w1536:dbl)  [unwired: 1 in, 5 out]
            n986 = local read "rough extra scan depth \nboth sides(mm)"() -> (w1535:dbl)
            n987 = Divide(x=w1535, y=w1536) -> (x/y=w1539:dbl)
            n988 = local read "number of steps"() -> (w1540:dbl)
            n989 = Multiply(x=w1539, y=w1534) -> (x*y=w1538:dbl)
            n990 = Round To Nearest(number=w1538) -> (nearest integer value=w1537:dbl)
            n991 = local read "scan depth (mm)"() -> (w1559:dbl)
            n992 = local read "focus point"() -> (w1545:dbl)
            n993 = Divide(x=w1537, y=w1534) -> (x/y=w1533:dbl)
            n994 = Divide(x=w1559, y=w1540) -> (x/y=w1564:dbl)
            n995 = Multiply(x=w1564, y=1000.0) -> (x*y=w1562:dbl)
            n996 = Multiply(x=2.0, y=w1536) -> (x*y=w1557:dbl)
            n997 = Round To Nearest(number=w1562) -> (nearest integer value=w1561:dbl)
            n998 = Add(x=w1540, y=w1557) -> (x+y=w1556:dbl)
            n999 = Multiply(x=w1536, y=w1533) -> (x*y=w1544:dbl)
            n1000 = Multiply(x=w1544, y=2.0) -> (x*y=w1553:dbl)
            n1001 = Divide(x=w1561, y=1000.0) -> (x/y=w1546:dbl)
            n1002 = Multiply(x=w1540, y=w1546) -> (x*y=w1554:dbl)
            n1003 = local write "stepsize (mm)"(w1546) -> ()
            n1004 = Add(x=w1554, y=w1553) -> (x+y=w1543:dbl)
            n1005 = local write "total nr of steps"(w1556) -> ()
            n1006 = Divide(x=w1543, y=2.0) -> (x/y=w1542:dbl)
            n1007 = Multiply(x=w1542, y=w1549) -> (x*y=w1552:dbl)
            n1008 = Round To Nearest(number=w1552) -> (nearest integer value=w1551:dbl)
            n1009 = Divide(x=w1551, y=w1549) -> (x/y=w1550:dbl)
            n1010 = Subtract(x=w1545, y=w1550) -> (x-y=w1548:dbl)
            n1011 = Add(x=w1550, y=w1545) -> (x+y=w1547:dbl)
            n1012 = local write "total scan depth"(w1543) -> ()
            n1013 = local write "start"(w1548) -> ()
            n1014 = local write "end"(w1547) -> ()
          }
          event "use nonlin steps": Value Change {
            n1015 = event-data() -> ("NewVal"=w1566:bool)  [unwired: 1 in, 5 out]
            n1016 = case shown="True" w1566 {
              frame True {
                w1567 = 1000.0 ("y")
                w1588 = T15."Enabled" ("Disabled")
                n1017 = property on="rough extra number \nof steps both sides" class="DigNum (strict)"("DisabledEnum"=w1588) -> ("Value"=w1583:dbl)  [unwired: 2 in, 2 out]
                n1018 = property on="rough stepsize (mm)" class="DigNum (strict)"("DisabledEnum"=w1588) -> ("Value"=w1584:dbl)  [unwired: 2 in, 2 out]
                n1019 = local read "stepsize (mm)"() -> (w1581:dbl)
                n1020 = local read "focus point"() -> (w1573:dbl)
                n1021 = Multiply(x=2.0, y=w1583) -> (x*y=w1585:dbl)
                n1022 = local read "number of steps"() -> (w1582:dbl)
                n1023 = Multiply(x=w1583, y=w1584) -> (x*y=w1580:dbl)
                n1024 = property on="rough extra scan depth \nboth sides(mm)" class="DigNum (strict)"("DisabledEnum"=w1588, "Value"=w1580) -> ()  [unwired: 2 in, 2 out]
                n1025 = Add(x=w1585, y=w1582) -> (x+y=w1587:dbl)
                n1026 = Multiply(x=w1580, y=2.0) -> (x*y=w1577:dbl)
                n1027 = local write "total nr of steps"(w1587) -> ()
                n1028 = Multiply(x=w1582, y=w1581) -> (x*y=w1578:dbl)
                n1029 = Add(x=w1578, y=w1577) -> (x+y=w1576:dbl)
                n1030 = Divide(x=w1576, y=2.0) -> (x/y=w1571:dbl)
                n1031 = Multiply(x=w1571, y=w1567) -> (x*y=w1570:dbl)
                n1032 = Round To Nearest(number=w1570) -> (nearest integer value=w1569:dbl)
                n1033 = Divide(x=w1569, y=w1567) -> (x/y=w1568:dbl)
                n1034 = local write "total scan depth"(w1576) -> ()
                n1035 = Subtract(x=w1573, y=w1568) -> (x-y=w1574:dbl)
                n1036 = Add(x=w1568, y=w1573) -> (x+y=w1572:dbl)
                n1037 = local write "start"(w1574) -> ()
                n1038 = local write "end"(w1572) -> ()
              }
              frame False {
                w1590 = 1000.0 ("y")
                w1601 = T15."Disabled and Grayed Out" ("Disabled")
                n1039 = property on="rough extra number \nof steps both sides" class="DigNum (strict)"("DisabledEnum"=w1601) -> ()  [unwired: 2 in, 2 out]
                n1040 = property on="rough stepsize (mm)" class="DigNum (strict)"("DisabledEnum"=w1601) -> ()  [unwired: 2 in, 2 out]
                n1041 = property on="rough extra scan depth \nboth sides(mm)" class="DigNum (strict)"("DisabledEnum"=w1601) -> ()  [unwired: 2 in, 2 out]
                n1042 = local read "stepsize (mm)"() -> (w1600:dbl)
                n1043 = local read "focus point"() -> (w1597:dbl)
                n1044 = local read "number of steps"() -> (w1595:dbl)
                n1045 = Multiply(x=w1595, y=w1600) -> (x*y=w1594:dbl)
                n1046 = local write "total nr of steps"(w1595) -> ()
                n1047 = local write "total scan depth"(w1594) -> ()
                n1048 = Divide(x=w1594, y=2.0) -> (x/y=w1593:dbl)
                n1049 = Multiply(x=w1593, y=w1590) -> (x*y=w1592:dbl)
                n1050 = Round To Nearest(number=w1592) -> (nearest integer value=w1591:dbl)
                n1051 = Divide(x=w1591, y=w1590) -> (x/y=w1589:dbl)
                n1052 = Subtract(x=w1597, y=w1589) -> (x-y=w1598:dbl)
                n1053 = Add(x=w1589, y=w1597) -> (x+y=w1596:dbl)
                n1054 = local write "start"(w1598) -> ()
                n1055 = local write "end"(w1596) -> ()
              }
            }
          }
          event "focus point": Value Change {
            n1056 = event-data() -> ("NewVal"=w1604:dbl)  [unwired: 1 in, 5 out]
            n1057 = local read "use nonlin steps"() -> (w1603:bool)
            n1058 = case shown="True" w1603 {
              tunnel: w1604 -> [w1613 w1632]
              frame True {
                w1616 = 1000.0 ("y")
                # "set focuspoint recalculate start and end based on\n stepsize and  number of steps of rough and fine"
                n1059 = local read "rough extra number \nof steps both sides"() -> (w1611:dbl)
                n1060 = local read "stepsize (mm)"() -> (w1612:dbl)
                n1061 = local read "rough stepsize (mm)"() -> (w1609:dbl)
                n1062 = local read "number of steps"() -> (w1605:dbl)
                n1063 = Divide(x=w1605, y=2.0) -> (x/y=w1625:dbl)
                n1064 = Round To Nearest(number=w1625) -> (nearest integer value=w1607:dbl)
                n1065 = Multiply(x=w1611, y=2.0) -> (x*y=w1608:dbl)
                n1066 = Multiply(x=w1608, y=w1609) -> (x*y=w1623:dbl)
                n1067 = Multiply(x=w1607, y=w1612) -> (x*y=w1624:dbl)
                n1068 = Add(x=w1624, y=w1623) -> (x+y=w1622:dbl)
                n1069 = Divide(x=w1622, y=2.0) -> (x/y=w1620:dbl)
                n1070 = Add(x=w1605, y=w1608) -> (x+y=w1606:dbl)
                n1071 = Multiply(x=w1620, y=w1616) -> (x*y=w1619:dbl)
                n1072 = Round To Nearest(number=w1619) -> (nearest integer value=w1618:dbl)
                n1073 = Divide(x=w1618, y=w1616) -> (x/y=w1617:dbl)
                n1074 = Subtract(x=w1613, y=w1617) -> (x-y=w1615:dbl)
                n1075 = Add(x=w1617, y=w1613) -> (x+y=w1614:dbl)
                n1076 = local write "total nr of steps"(w1606) -> ()
                n1077 = local write "start"(w1615) -> ()
                n1078 = local write "end"(w1614) -> ()
              }
              frame False {
                # "set focuspoint recalculate start and end based on\n stepsize and number of steps"
                n1079 = local read "stepsize (mm)"() -> (w1633:dbl)
                n1080 = local read "number of steps"() -> (w1630:dbl)
                n1081 = Divide(x=w1630, y=2.0) -> (x/y=w1635:dbl)
                n1082 = Round To Nearest(number=w1635) -> (nearest integer value=w1634:dbl)
                n1083 = Multiply(x=w1634, y=w1633) -> (x*y=w1631:dbl)
                n1084 = Subtract(x=w1632, y=w1631) -> (x-y=w1628:dbl)
                n1085 = Add(x=w1632, y=w1631) -> (x+y=w1627:dbl)
                n1086 = Subtract(x=w1627, y=w1628) -> (x-y=w1629:dbl)
                n1087 = local write "start"(w1628) -> ()
                n1088 = local write "end"(w1627) -> ()
                n1089 = local write "total scan depth"(w1629) -> ()
                n1090 = local write "total nr of steps"(w1630) -> ()
              }
            }
          }
          event "Microscope light on/off": Value Change {
            # "toggle port1 line 3 for triggering IR light"
            n1091 = event-data() -> ("NewVal"=w1639:bool)  [unwired: 1 in, 5 out]
            n1092 = local read "testrun without daq"() -> (w1637:bool)
            n1093 = case shown="False" w1637 {
              tunnel: w1639 -> [w1640 _]
              frame False {
                n1094 = case shown="True" w1640 {
                  frame False {
                    n1095 = call-poly <vilib>:"DAQmx Write.vi"("task/channels in"=refnum<k21> "ringlight(blue)", "data"=0.0) -> ()  [unwired: 11 in, 3 out]
                  }
                  frame True {
                    n1096 = call-poly <vilib>:"DAQmx Write.vi"("task/channels in"=refnum<k21> "ringlight(blue)", "data"=5.0) -> ()  [unwired: 11 in, 3 out]
                  }
                }
              }
              frame True {
              }
            }
          }
          event "scan depth (mm)": Value Change {
            n1097 = event-data() -> ("NewVal"=w1647:dbl)  [unwired: 1 in, 5 out]
            n1098 = local read "use nonlin steps"() -> (w1646:bool)
            n1099 = case shown="True" w1646 {
              tunnel: w1647 -> [w1653 w1667]
              frame False {
                w1649 = 1000.0 ("x")
                # "change scan depth  recalculate number of steps based \non stepsize change start and end, keep focus point"
                n1100 = Divide(x=w1653, y=2.0) -> (x/y=w1652:dbl)
                n1101 = Multiply(x=w1649, y=w1652) -> (x*y=w1651:dbl)
                n1102 = Round To Nearest(number=w1651) -> (nearest integer value=w1650:dbl)
                n1103 = Divide(x=w1650, y=w1649) -> (x/y=w1648:dbl)
                n1104 = local read "focus point"() -> (w1657:dbl)
                n1105 = local read "stepsize (mm)"() -> (w1659:dbl)
                n1106 = Subtract(x=w1657, y=w1648) -> (x-y=w1656:dbl)
                n1107 = Add(x=w1657, y=w1648) -> (x+y=w1655:dbl)
                n1108 = Divide(x=w1653, y=w1659) -> (x/y=w1658:dbl)
                n1109 = local write "start"(w1656) -> ()
                n1110 = local write "end"(w1655) -> ()
                n1111 = Round To Nearest(number=w1658) -> (nearest integer value=w1654:dbl)
                n1112 = local write "number of steps"(w1654) -> ()
                n1113 = local write "total scan depth"(w1653) -> ()
                n1114 = local write "total nr of steps"(w1654) -> ()
              }
              frame True {
                w1672 = 1000.0 ("y")
                # "change scan depth  recalculate number of steps based \non stepsize change start and end, keep focus point"
                n1115 = local read "rough extra scan depth \nboth sides(mm)"() -> (w1668:dbl)
                n1116 = local read "rough extra number \nof steps both sides"() -> (w1665:dbl)
                n1117 = local read "stepsize (mm)"() -> (w1681:dbl)
                n1118 = Divide(x=w1667, y=w1681) -> (x/y=w1680:dbl)
                n1119 = Round To Nearest(number=w1680) -> (nearest integer value=w1662:dbl)
                n1120 = local write "number of steps"(w1662) -> ()
                n1121 = Multiply(x=w1665, y=2.0) -> (x*y=w1663:dbl)
                n1122 = Multiply(x=w1668, y=2.0) -> (x*y=w1675:dbl)
                n1123 = Add(x=w1663, y=w1662) -> (x+y=w1661:dbl)
                n1124 = Add(x=w1667, y=w1675) -> (x+y=w1666:dbl)
                n1125 = local write "total nr of steps"(w1661) -> ()
                n1126 = local write "total scan depth"(w1666) -> ()
                n1127 = Divide(x=w1666, y=2.0) -> (x/y=w1676:dbl)
                n1128 = Multiply(x=w1676, y=w1672) -> (x*y=w1677:dbl)
                n1129 = Round To Nearest(number=w1677) -> (nearest integer value=w1678:dbl)
                n1130 = local read "focus point"() -> (w1669:dbl)
                n1131 = Divide(x=w1678, y=w1672) -> (x/y=w1679:dbl)
                n1132 = Add(x=w1679, y=w1669) -> (x+y=w1670:dbl)
                n1133 = Subtract(x=w1669, y=w1679) -> (x-y=w1671:dbl)
                n1134 = local write "start"(w1671) -> ()
                n1135 = local write "end"(w1670) -> ()
              }
            }
          }
          event "User Interface": Value Change {
            # "change the place of the tab splitter"
            n1136 = event-data() -> ("NewVal"=w1682:bool)  [unwired: 1 in, 5 out]
            n1137 = case shown="False" w1682 {
              frame True {
                n1138 = property on="Splitter 2" class="Splitter"("Position"=1 ("Splitter Position")) -> ()  [unwired: 2 in, 2 out]
              }
              frame False {
                n1139 = local read "Splitter Position"() -> (w1685:i32)
                n1140 = property on="Splitter 2" class="Splitter"("Position"=w1685) -> ()  [unwired: 2 in, 2 out]
              }
            }
          }
          event "plant light %": Value Change {
            # "set the intensity of the plant light"
            n1141 = event-data() -> ("NewVal"=w1686:dbl)  [unwired: 1 in, 5 out]
            n1142 = Divide(x=w1686, y=10.0) -> (x/y=w1687:dbl)
            n1143 = local write "plight [%]"(w1686) -> ()
            n1144 = call-poly <vilib>:"DAQmx Write.vi"("task/channels in"=refnum<k21> "plantlight(red)", "data"=w1687) -> ()  [unwired: 11 in, 3 out]
          }
          event "blue", "blue": Value Change {
            n1145 = event-data() -> ()  [unwired: 1 in, 6 out]
            n1146 = local read "testrun without psi light"() -> (w1691:bool)
            n1147 = case shown="True" w1691 {
              frame False {
              }
              frame True {
                # "set the intensity of the plant light"
                n1148 = local read "blue"() -> (w1696:dbl)
                n1149 = local read "blue"() -> (w1695:bool)
                n1150 = case shown="False" w1695 {
                  tunnel: ["ST\u0010\u00028\u0000-" ("write buffer") "ST\u0010\u00028\u0001," ("write buffer")] -> w1697
                  frame False {
                    # "switch blue channel off"
                  }
                  frame True {
                    # "switch blue channel on"
                  }
                }
                n1151 = Multiply(x=w1696, y=10.22) -> (x*y=w1700:dbl)
                n1152 = call "power command.vi"("channel"=chan_select."blue", "power [0-1022]"=w1700) -> ("resulting string incl crc"=w1699:string)
                n1153 = local read "serial psi channel"() -> (w1693:refnum<visa-resource-name>)
                n1154 = VISA Write(VISA resource name=w1693, write buffer=w1699) -> (VISA resource name out=w1694:refnum<visa-resource-name>)  [unwired: 1 in, 2 out]
                n1155 = VISA Write(VISA resource name=w1694, write buffer=w1697) -> (VISA resource name out=w1698:refnum<visa-resource-name>)  [unwired: 1 in, 2 out]
                n1156 = VISA Close(VISA resource name=w1698) -> ()  [unwired: 1 in, 1 out]
              }
            }
          }
          event "green", "green": Value Change {
            n1157 = event-data() -> ()  [unwired: 1 in, 6 out]
            n1158 = local read "testrun without psi light"() -> (w1705:bool)
            n1159 = case shown="True" w1705 {
              frame False {
              }
              frame True {
                # "set the intensity of the plant light"
                n1160 = local read "green"() -> (w1710:dbl)
                n1161 = local read "green"() -> (w1709:bool)
                n1162 = case shown="True" w1709 {
                  tunnel: ["ST\u0010\u0002\u0018\u0000\r" ("write buffer") "ST\u0010\u0002\u0018\u0001\f" ("write buffer")] -> w1711
                  frame False {
                    # "switch green channel off"
                  }
                  frame True {
                    # "switch green channel on"
                  }
                }
                n1163 = Multiply(x=w1710, y=10.22) -> (x*y=w1714:dbl)
                n1164 = call "power command.vi"("channel"=chan_select."green", "power [0-1022]"=w1714) -> ("resulting string incl crc"=w1713:string)
                n1165 = local read "serial psi channel"() -> (w1707:refnum<visa-resource-name>)
                n1166 = VISA Write(VISA resource name=w1707, write buffer=w1713) -> (VISA resource name out=w1708:refnum<visa-resource-name>)  [unwired: 1 in, 2 out]
                n1167 = VISA Write(VISA resource name=w1708, write buffer=w1711) -> (VISA resource name out=w1712:refnum<visa-resource-name>)  [unwired: 1 in, 2 out]
                n1168 = VISA Close(VISA resource name=w1712) -> ()  [unwired: 1 in, 1 out]
              }
            }
          }
          event "red", "red": Value Change {
            n1169 = event-data() -> ()  [unwired: 1 in, 6 out]
            n1170 = local read "testrun without psi light"() -> (w1719:bool)
            n1171 = case shown="False" w1719 {
              frame False {
                # "set the intensity of the plant light"
                n1172 = local read "red"() -> (w1721:bool)
                n1173 = local read "red"() -> (w1724:dbl)
                n1174 = case shown="False" w1721 {
                  tunnel: ["ST\u0010\u00028\u0000-" ("write buffer") "ST\u0010\u00028\u0001," ("write buffer")] -> w1725
                  frame False {
                    # "switch red channel off"
                  }
                  frame True {
                    # "switch red channel on"
                  }
                }
                n1175 = Multiply(x=w1724, y=10.22) -> (x*y=w1728:dbl)
                n1176 = call "power command.vi"("channel"=chan_select."red", "power [0-1022]"=w1728) -> ("resulting string incl crc"=w1727:string)
                n1177 = local read "serial psi channel"() -> (w1722:refnum<visa-resource-name>)
                n1178 = VISA Write(VISA resource name=w1722, write buffer=w1727) -> (VISA resource name out=w1723:refnum<visa-resource-name>)  [unwired: 1 in, 2 out]
                n1179 = VISA Write(VISA resource name=w1723, write buffer=w1725) -> (VISA resource name out=w1726:refnum<visa-resource-name>)  [unwired: 1 in, 2 out]
                n1180 = VISA Close(VISA resource name=w1726) -> ()  [unwired: 1 in, 1 out]
              }
              frame True {
              }
            }
          }
          event "Hide test feat.": Value Change {
            # "set the intensity of the plant light"
            n1181 = event-data() -> ("NewVal"=w1733:bool)  [unwired: 1 in, 5 out]
            n1182 = case shown="False" w1733 {
              frame False {
                w1735 = T34."Always Off" ("Vertical Scrollbar Visibility")
                w1738 = T34."Always Off" ("Vertical Scrollbar Visibility")
                # "hide test features"
                n1183 = property on="Splitter" class="Splitter"("Position"=47 ("Splitter Position")) -> ()  [unwired: 2 in, 2 out]
                n1184 = property on="Pane" class="Pane"("VertScrollbarVisibility"=w1738, "HorizScrollbarVisibility"=w1738, "PaneColor"=u32 14869218 ("Pane Color")) -> ()  [unwired: 2 in, 2 out]
                n1185 = property on="Pane 3" class="Pane"("VertScrollbarVisibility"=w1735, "HorizScrollbarVisibility"=w1735) -> ()  [unwired: 2 in, 2 out]
              }
              frame True {
                w1739 = T34."Always On" ("Vertical Scrollbar Visibility")
                w1742 = T34."Always On" ("Horizontal Scrollbar Visibility")
                # "show test features"
                n1186 = property on="Splitter" class="Splitter"("Position"=120 ("Splitter Position")) -> ()  [unwired: 2 in, 2 out]
                n1187 = property on="Pane" class="Pane"("HorizScrollbarVisibility"=w1742, "VertScrollbarVisibility"=w1742, "PaneColor"=u32 16774656 ("Pane Color")) -> ()  [unwired: 2 in, 2 out]
                n1188 = property on="Pane 3" class="Pane"("VertScrollbarVisibility"=w1739, "HorizScrollbarVisibility"=w1739) -> ()  [unwired: 2 in, 2 out]
              }
            }
          }
          event "rough extra scan depth \nboth sides(mm)": Value Change {
            w1757 = 1000.0 ("y")
            # "change extra  scan depth  recalculate number of steps based \non stepsize change start and end, keep focus point"
            n1189 = event-data() -> ("NewVal"=w1746:dbl)  [unwired: 1 in, 5 out]
            n1190 = local read "rough stepsize (mm)"() -> (w1747:dbl)
            n1191 = local read "scan depth (mm)"() -> (w1748:dbl)
            n1192 = Divide(x=w1746, y=w1747) -> (x/y=w1745:dbl)
            n1193 = local read "number of steps"() -> (w1750:dbl)
            n1194 = Multiply(x=w1746, y=2.0) -> (x*y=w1760:dbl)
            n1195 = Round To Nearest(number=w1745) -> (nearest integer value=w1744:dbl)
            n1196 = Add(x=w1748, y=w1760) -> (x+y=w1753:dbl)
            n1197 = local write "rough extra number \nof steps both sides"(w1744) -> ()
            n1198 = Multiply(x=w1744, y=2.0) -> (x*y=w1751:dbl)
            n1199 = local write "total scan depth"(w1753) -> ()
            n1200 = Divide(x=w1753, y=2.0) -> (x/y=w1761:dbl)
            n1201 = Add(x=w1751, y=w1750) -> (x+y=w1749:dbl)
            n1202 = Multiply(x=w1761, y=w1757) -> (x*y=w1762:dbl)
            n1203 = Round To Nearest(number=w1762) -> (nearest integer value=w1763:dbl)
            n1204 = local write "total nr of steps"(w1749) -> ()
            n1205 = local read "focus point"() -> (w1754:dbl)
            n1206 = Divide(x=w1763, y=w1757) -> (x/y=w1764:dbl)
            n1207 = Subtract(x=w1754, y=w1764) -> (x-y=w1756:dbl)
            n1208 = Add(x=w1764, y=w1754) -> (x+y=w1755:dbl)
            n1209 = local write "start"(w1756) -> ()
            n1210 = local write "end"(w1755) -> ()
          }
          event "Test scan\n(no pic. saved)": Value Change {
            n1211 = event-data() -> ("NewVal"=w1765:bool)  [unwired: 1 in, 5 out]
            n1212 = local write "step nr"(0.0 ("step nr")) -> ()
            n1213 = case shown="True" w1765 {
              tunnel: [w1771 w1777] -> w1770
              tunnel: [w1772 wobbe_statemachine."start scan timer" ("Initial State")] -> w1766
              frame False {
                w1772 = wobbe_statemachine."set up measurement" ("Initial State")
                n1214 = Build Array(w1772) -> (w1771:T1[])
              }
              frame True {
                # "start timer at begin of scan"
                n1215 = local read "use nonlin steps"() -> (w1776:bool)
                n1216 = case shown="False" w1776 {
                  tunnel: [w1782 w1787] -> w1777
                  frame True {
                    # "nonlin scan"
                    # "stop the scan timer"
                    # "back to menu"
                    # "move back to start position with backlash"
                    # "do nonlin scan without saving picture"
                    n1217 = Build Array(wobbe_statemachine."do non lin test scan" ("Initial State"), wobbe_statemachine."move to start " ("Initial State"), wobbe_statemachine."stop scan timer" ("Initial State"), wobbe_statemachine."set up measurement" ("Initial State")) -> (w1782:T1[])
                  }
                  frame False {
                    # "lineair scan"
                    # "stop the scan timer"
                    # "back to menu"
                    # "move back to start position with backlash"
                    # "do scan without saving picture"
                    n1218 = Build Array(wobbe_statemachine."do test scan" ("Initial State"), wobbe_statemachine."move to start " ("Initial State"), wobbe_statemachine."stop scan timer" ("Initial State"), wobbe_statemachine."set up measurement" ("Initial State")) -> (w1787:T1[])
                  }
                }
                n1219 = local write "Test scan\n(no pic. saved)"(FALSE ("Test scan\n(no pic. saved)")) -> ()
                n1220 = local write "temp test scan"(TRUE ("temp test scan")) -> ()
              }
            }
            n1221 = local write "waveform tab"(T12."setup measurement" ("waveform tab")) -> ()
          }
          event "start meas now": Value Change {
            # "back to menu"
            # "do n scans with measurement settings"
            # "select path to save scan"
            n1222 = event-data() -> ()  [unwired: 1 in, 6 out]
            n1223 = local write "waveform tab"(T12."measurement" ("waveform tab")) -> ()
            n1224 = Build Array(wobbe_statemachine."do multi point scan " ("Initial State"), wobbe_statemachine."set up measurement" ("Initial State")) -> (w1793:T1[])
          }
          event "Run with \nexternal \ntiming settings": Value Change {
            # "do scans with measurement settings from external file"
            n1225 = event-data() -> ("NewVal"=w1794:bool)  [unwired: 1 in, 5 out]
            n1226 = case shown="True" w1794 {
              tunnel: [w1803 w1808] -> w1797
              tunnel: [wobbe_statemachine."select save path" ("Initial State") wobbe_statemachine."set up measurement" ("Initial State")] -> w1796
              tunnel: [TRUE ("stop setup loop") FALSE ("stop setup loop")] -> w1795
              frame True {
                # "back to menu"
                # "select path to save scan"
                n1227 = local write "waveform tab"(T12."long wait timer" ("waveform tab")) -> ()
                n1228 = Build Array(wobbe_statemachine."timerscan" ("Initial State"), wobbe_statemachine."set up measurement" ("Initial State")) -> (w1803:T1[])
              }
              frame False {
                # "back to menu"
                # "select path to save scan"
                n1229 = local write "waveform tab"(T12."long wait timer" ("waveform tab")) -> ()
                n1230 = Build Array(wobbe_statemachine."set up measurement" ("Initial State")) -> (w1808:T1[])
              }
            }
          }
          event "start fast timer": Value Change {
            # "run simple wait  timer"
            # "back to menu"
            # "start fast timer and do n scans with measurement settings\nis canceled with pressing button again"
            # "select path to save scan"
            n1231 = event-data() -> ()  [unwired: 1 in, 6 out]
            n1232 = local write "waveform tab"(T12."measurement" ("waveform tab")) -> ()
            n1233 = Build Array(wobbe_statemachine."simple timer" ("Initial State"), wobbe_statemachine."do multi point scan " ("Initial State"), wobbe_statemachine."set up measurement" ("Initial State")) -> (w1815:T1[])
          }
        }
        n1234 = flat-sequence {
          tunnel: w1364 -> [w1371]
          tunnel: w1363 -> [w1370]
          tunnel: w1362 -> [w1372]
          frame #0 {
            "state array" <- w1371
            "Initial State" <- w1370
          }
          frame #1 {
            "stop setup loop" <- w1372
          }
        }
      }
      n1235 = local write "error in"(w1361) -> ()
    }
  }
  n1236 = flat-sequence {
    tunnel: w1 -> [w1817]
    frame #0 {
      n1237 = call <vilib>:"Simple Error Handler.vi"("error in (no error)"=w1817) -> ()  [unwired: 4 in, 5 out]
      n1238 = local write "stopprogram"(FALSE ("stopprogram")) -> ()
    }
  }
